vi "rio_veloster10.vi"() -> ()   [LabVIEW 2015]
uses:
  <vilib>/Analysis/Matrix/Datatypes/RealMatrix.ctl
  <vilib>/FPGAPlugInAG/cRIO-9113/niLvFpga_Open_cRIO-9113.vi
  <vilib>/rvi/interface/common/dynamic/niFpgaDynamicAddResources.vi
  <vilib>/FPGAPlugInAG/Dynamic/niLvFpga_Abort_Dynamic.vi
  <vilib>/FPGAPlugInAG/Dynamic/niLvFpga_Run_Dynamic.vi
  G_rio.vi
  <vilib>/Instr/_visa.llb/VISA Configure Serial Port (Instr).vi
  <vilib>/Utility/error.llb/Error Cluster From Error Code.vi
  <vilib>/rvi/errors/niLvFpgaAdjustHostInterfaceError.vi
  <vilib>/Analysis/Matrix/Numeric/Conversions/Array To Matrix - RA2.vi
  <vilib>/Analysis/Matrix/Numeric/Multiply/Multiply - RM,RM.vi
  <vilib>/Analysis/Matrix/Numeric/Add/Add - RM,RM.vi
  <vilib>/Analysis/baseanly.llb/Real Inverse Matrix.vi
  <vilib>/Analysis/Matrix/Numeric/Subtract/Subtract - RM,RM.vi
  <vilib>/Analysis/Matrix/Numeric/Conversions/Array To Matrix - RA.vi
  <vilib>/Analysis/Matrix/Numeric/Multiply/Multiply - R,RM.vi
  <vilib>/Analysis/Matrix/Numeric/Conversions/Matrix To Array - RM.vi
  <vilib>/rvi/interface/nirviOpenFPGA/nirviOpenFPGA.xnode
  FPGA Bitfiles/autonomous_FPGATarget2_fpga4_FZHAM7r+pqE.lvbitx
  fpga/fpga4.vi
  <vilib>/rvi/interface/nirviMethod/nirviMethod.xnode
  <vilib>/rvi/interface/nirviReadWriteControl/nirviReadWriteControl.xnode
  <vilib>/rvi/interface/Simulation/niFpgaSimulationCallBeginRW.vi
  <vilib>/rvi/errors/niLvFpgaMergeErrorWithErrorCode.vi
  NiFpgaLv.dll
  <vilib>/FPGAPlugInAG/Dynamic/niLvFpga_ReadFifo_Dynamic.vi
  <vilib>/Analysis/Matrix/NI_Matrix.lvlib
  <vilib>/Analysis/NI_AALBase.lvlib
panel:
  in  "map name":T1(ring)
  out "316H":u8[](array[numeric])
  out "FPGA":refnum<k20>
  out "Key":u8
  out "mdps torque":dbl(graph)
  out "battery voltage 2":dbl
  in  "steer limit":dbl=100.0
  in  "buzz":bool
  out "hcount":u64=1
  out "hbias":dbl
  out "vcount":u64=1
  out "vgain":dbl=1.0
  in  "heading gain":dbl=1.414
  in  "pos gain":dbl=4.0
  out "Pos_time 10":i32
  out "T PWM":u16
  out "B PWM":u16
  out "solenoid":bool
  out "brk enc":u8
  out "shift lever":dbl
  in  "LCM":bool=TRUE
  out "mobileye":u8[](array[numeric])
  out "timer":u32
  out "Mobileye_time 100":u32
  out "H_GPS":dbl
  out "pos":dbl[](array[numeric])
  out "pos error":dbl
  in  "GPS init":bool=TRUE
  in  "Gear Manual":i32(slide)=1 scale=-1.0..1.0
  out "map":i32=2
  out "P, R, D":i32
  out "heading error":dbl
  out "POS init":bool
  out "VS_CAN":dbl
  in  "brake":bool
  in  "Slide":dbl(slide)=1000.0 min=1000.0 max=2000.0 step=1500.0 scale=1000.0..2000.0
  out "novatel":refnum<visa-resource-name>
  in  "ublox":bool
  out "rest":u8[](array[numeric])
  out "GPS_novatel_time":u32
  out "GPS_time 100":u32
  out "Con_time 10":i32
  out "CAN_time 10":u32
  out "gps2":refnum<visa-resource-name>
  out "gps1":refnum<visa-resource-name>
  out "Heading":dbl
  out "ecef ref":dbl[](array[numeric])
  out "h_gps":dbl
  out "pos_gps":dbl[](array[numeric]) format="%#_19f"
  out "get heading":bool
  out "get position":bool
  out "dt":dbl
  out "rt":dbl
  out "CAN Comm Enabled":bool
  in  "SPAS Enable":bool=TRUE
  in  "file write":bool
  out "data write":refnum<file>
  out "file rw error":errorcluster
  out "Ref steer":dbl=1.0
  in  "Steer input":bool=TRUE
  in  "Ref steer manual":dbl(knob) scale=-550.0..550.0
  out "Ref vel":dbl=1.0
  in  "Ref vel manual":dbl
  in  "Velocity input":bool
  out "Auto":bool
  out "Run":bool
  out "E - STOP":bool
  out "Throttle Enable":bool=TRUE
  # "P"
  # "R"
  # "D"
  # "Ref steer manual"
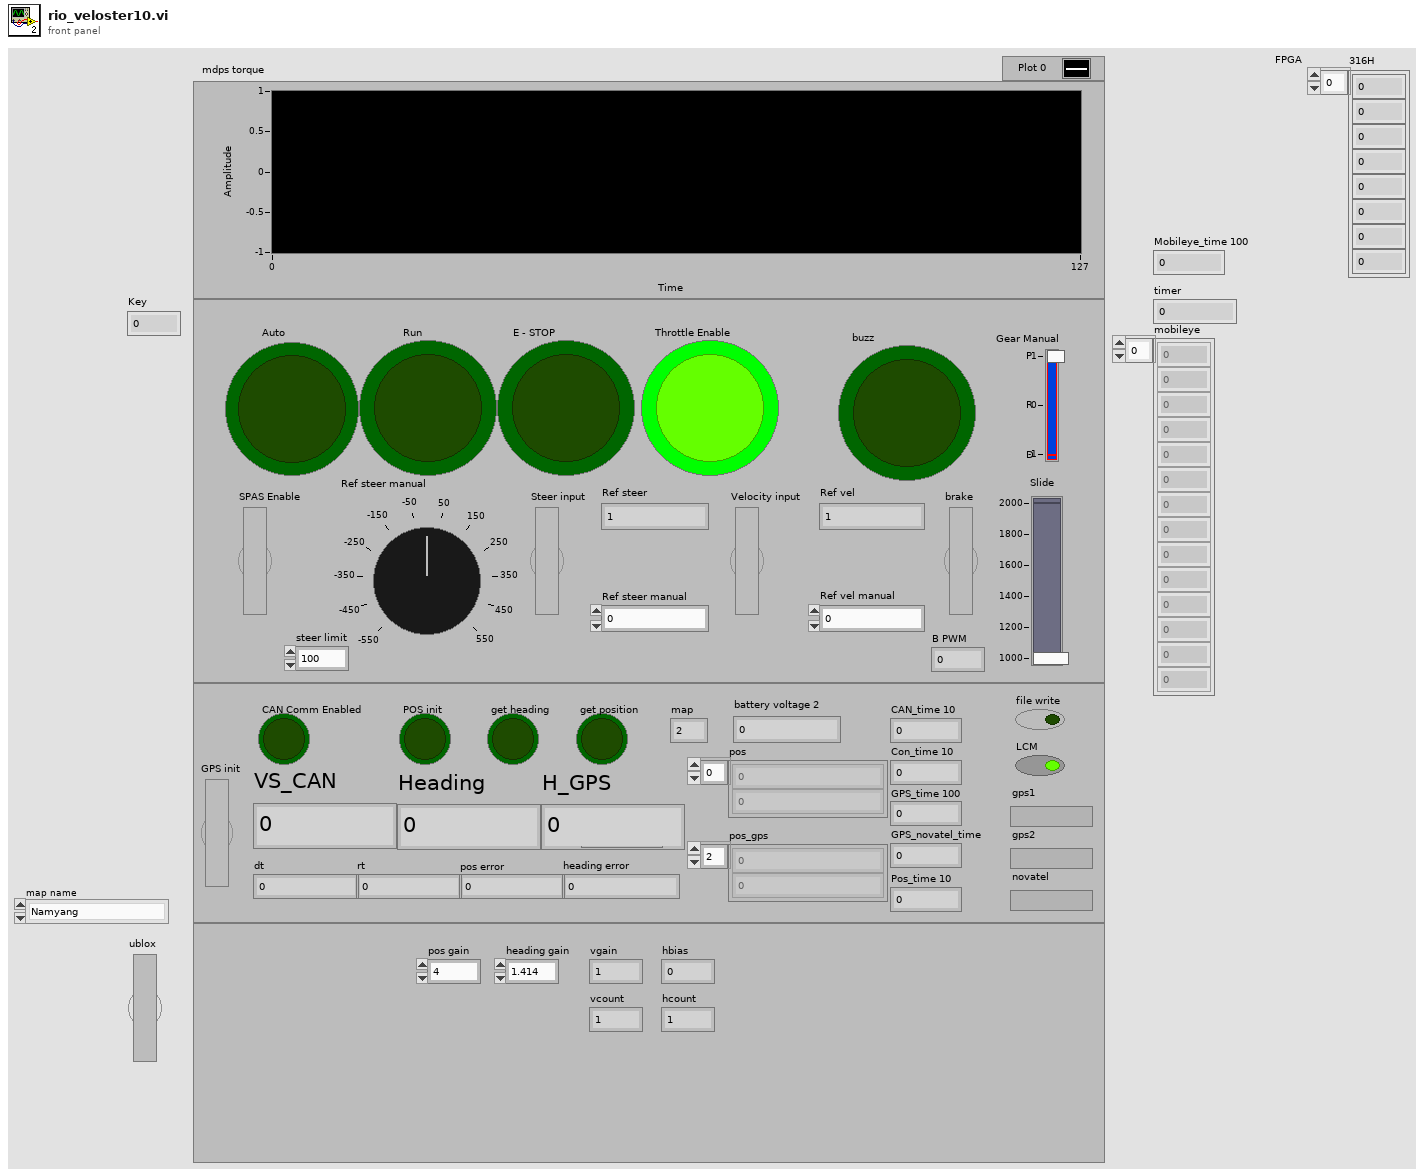
[diagram p1: front panel]
types:
  T1 = enum32{"Namyang", "Hyundai", "KAIST", "Ajou", "Munji", "Airforce", "Car", "KATRI", "Samsung", "Coex", "Gwangnaru", "Inje", "sinjin"}
  T2 = enum16{"open", "replace", "create", "open or create", "replace or create", "replace or create with confirmation"}
  T3 = cluster{"timestamp high":u32, "timestamp low":u32, "identifier":u32, "type":enum8{"Data Frame", "Remote Frame", "(reserved)", "(reserved) ", "(reserved)  ", "(reserved)   ", "Bus Error", "Transceiver Fault"}, "info A":u8, "info B":u8, "data length":u8, "data":u8[]}
  T4 = cluster{"connection ID":refnum<k16>, "net address":u32, "port":u16}
  T5 = cluster{"hash":i64, "sys time":i64, "mobileye":u8[]}
  T6 = cluster{"hash":i64, "sys time":i64, "n":i32, "error":i32[]}
  T7 = cluster{"hash":i64, "sys time":i64, "time":dbl, "yaw_rate":dbl, "mdps torque":dbl, "mdps str_ang":dbl, "VS_CAN":dbl, "lat_accel":dbl, "mcp":dbl, "accel pedal value":dbl, "tps":dbl, "odometer":dbl, "battery voltage":dbl, "WHL_SPD_RR":dbl, "WHL_SPD_RL":dbl, "WHL_SPD_FR":dbl, "WHL_SPD_FL":dbl}
  T8 = cluster{"hash":i64, "sys time":i64, "ref_vel":dbl, "ref_steer":dbl, "alert":u8}
  T9 = cluster{"hash":i64, "sys time":i64, "ref_vel":dbl, "ref_steer":dbl}
  T10 = cluster{"hash":i64, "sys time":i64, "Auto":bool, "Run":bool, "Solenoid":bool, "T lim":bool, "brk_enc":u8, "B PWM":u16, "T PWM":u16, "ref_vel":dbl, "ref_bkr_enc":dbl, "ref_apv":dbl, "ref_steer":dbl}
  T11 = typedef "NI_Matrix.lvlib/RealMatrix.ctl" = dbl[][]
  T12 = cluster{"hash":i64, "sys time":i64, "time":dbl, "x":dbl, "y":dbl, "h":dbl, "numSV":i32, "postype":i32, "lag":i32, "hordev":dbl, "lat":dbl, "lon":dbl, "hgt":dbl, "map_idx":i32}
  T13 = cluster{"LCC[0]":dbl, "LCC[1]":dbl, "LCC[2]":dbl, "LCC[3]":dbl, "LCC[4]":dbl, "LCC[5]":dbl, "LCC[6]":dbl, "LCC[7]":dbl, "LCC[8]":dbl, "LCC[9]":dbl, "LCC[10]":dbl, "LCC[11]":dbl, "LCC[12]":dbl, "LCC[13]":dbl, "LCC[14]":dbl}
  T14 = cluster{"hash":i64, "sys time":i64, "time":dbl, "speed":dbl, "heading":dbl, "lat":dbl, "lon":dbl}
  T15 = cluster{"vel[0]":dbl, "vel[1]":dbl, "vel[2]":dbl, "vel[3]":dbl, "vel[4]":dbl, "vel[5]":dbl, "vel[6]":dbl}
  T16 = cluster{"output[0]":dbl, "output[1]":dbl, "output[2]":dbl, "output[3]":dbl, "output[4]":dbl, "output[5]":dbl, "output[6]":dbl, "output[7]":dbl, "output[8]":dbl, "output[9]":dbl, "output[10]":dbl, "output[11]":dbl, "output[12]":dbl, "output[13]":dbl, "output[14]":dbl}
  T17 = cluster{"output[0]":dbl, "output[1]":dbl, "output[2]":dbl, "output[3]":dbl, "output[4]":dbl, "output[5]":dbl, "output[6]":dbl}
  T18 = cluster{"hash":i64, "sys time":i64, "dt":dbl, "x":dbl, "y":dbl, "speed":dbl, "heading":dbl, "yaw_rate":dbl}
  T19 = cluster{"Real 2D Array[0]":dbl, "Real 2D Array[1]":dbl, "Real 2D Array[2]":dbl, "Real 2D Array[3]":dbl, "Real 2D Array[4]":dbl}
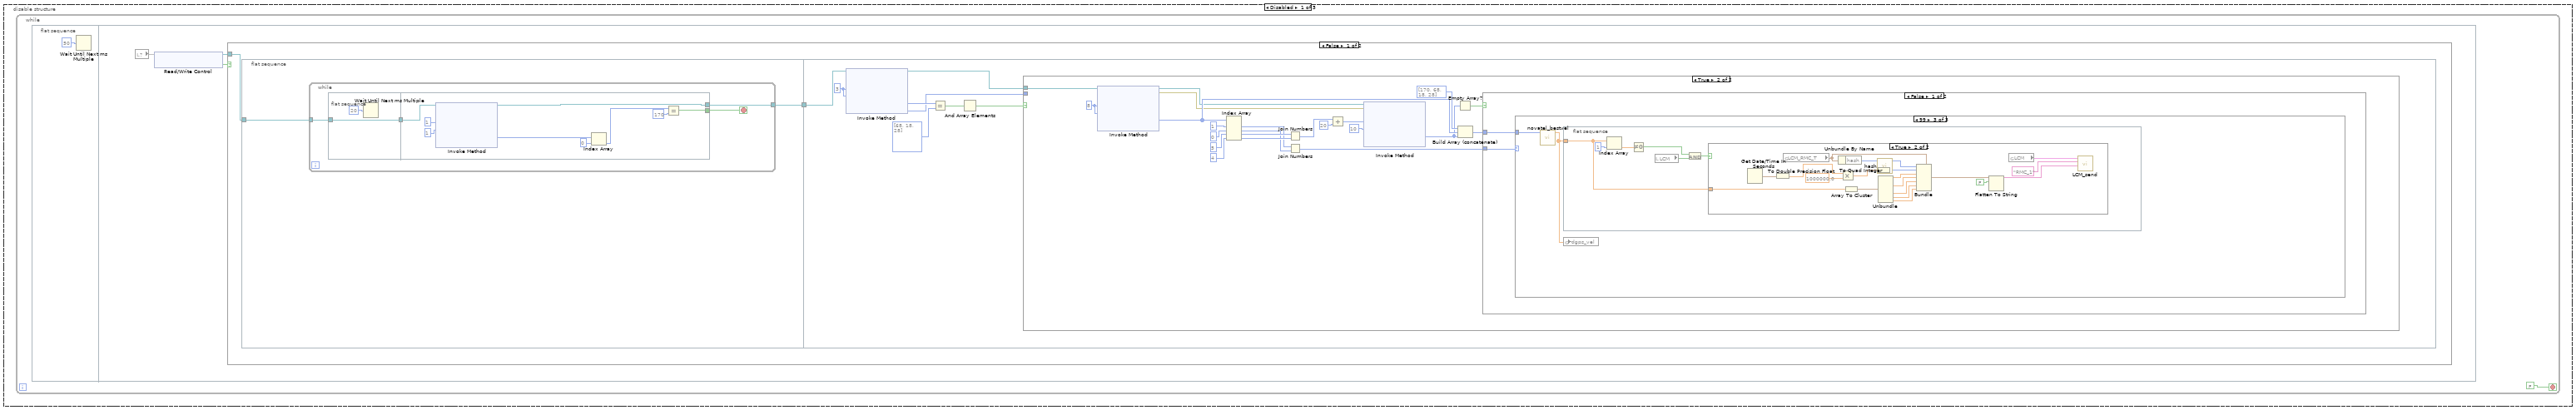
[diagram p2: hidden frame]
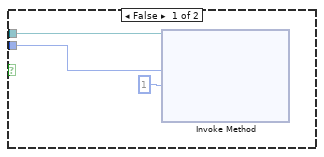
[diagram p3: hidden frame]
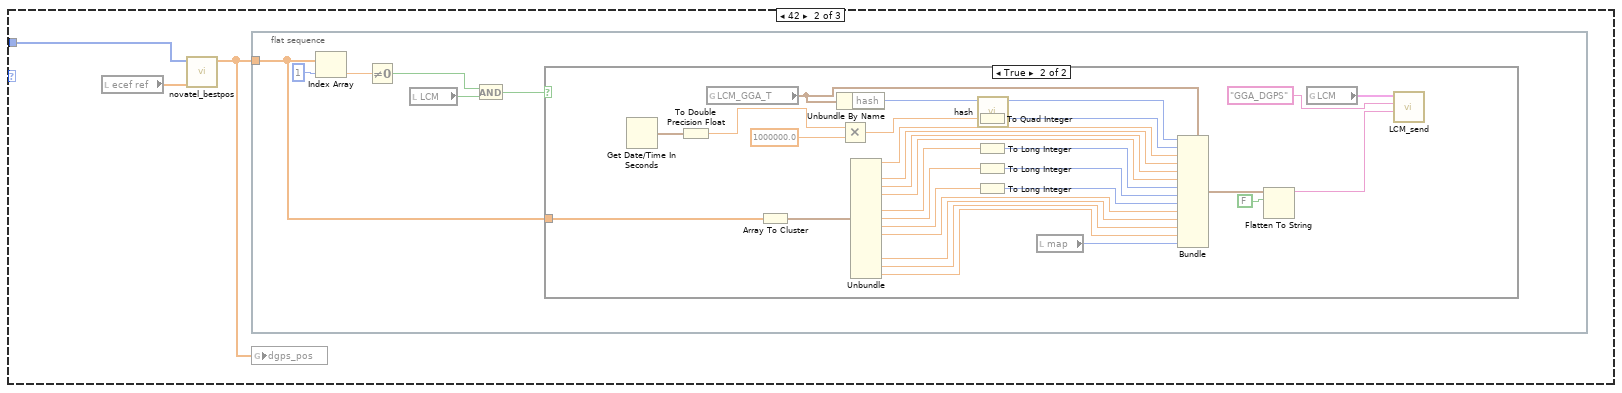
[diagram p5: hidden frame]
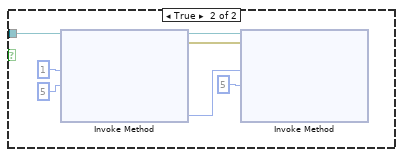
[diagram p9: hidden frame]
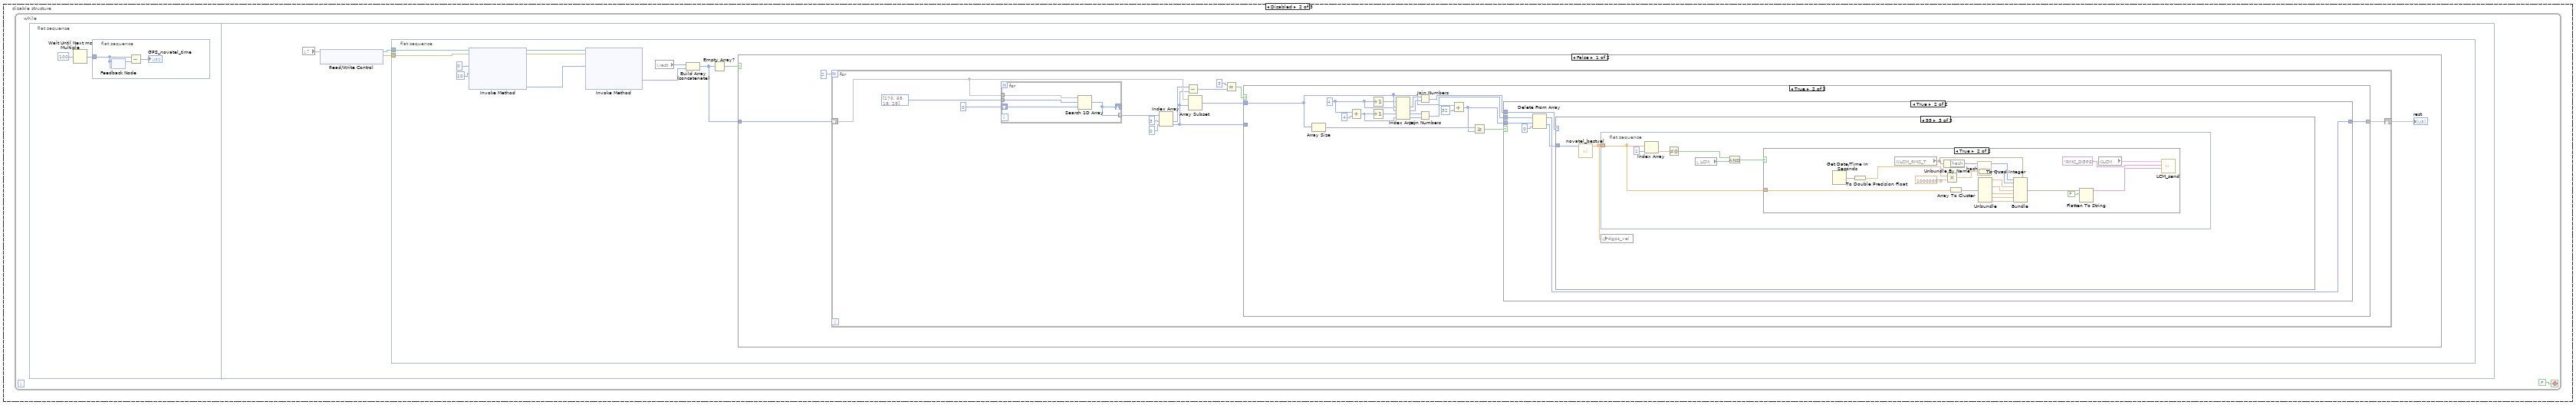
[diagram p10: hidden frame]
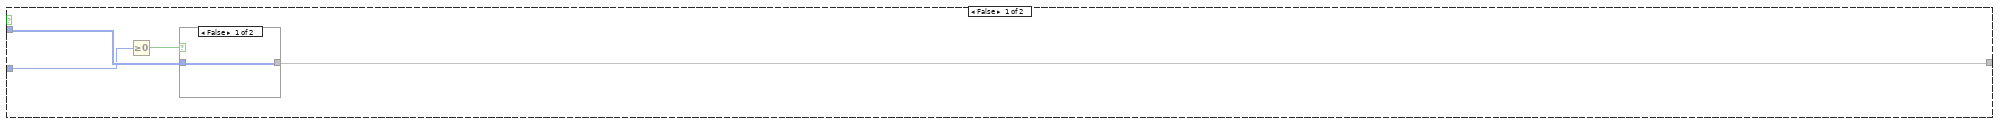
[diagram p11: hidden frame]
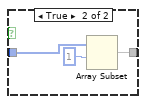
[diagram p12: hidden frame]
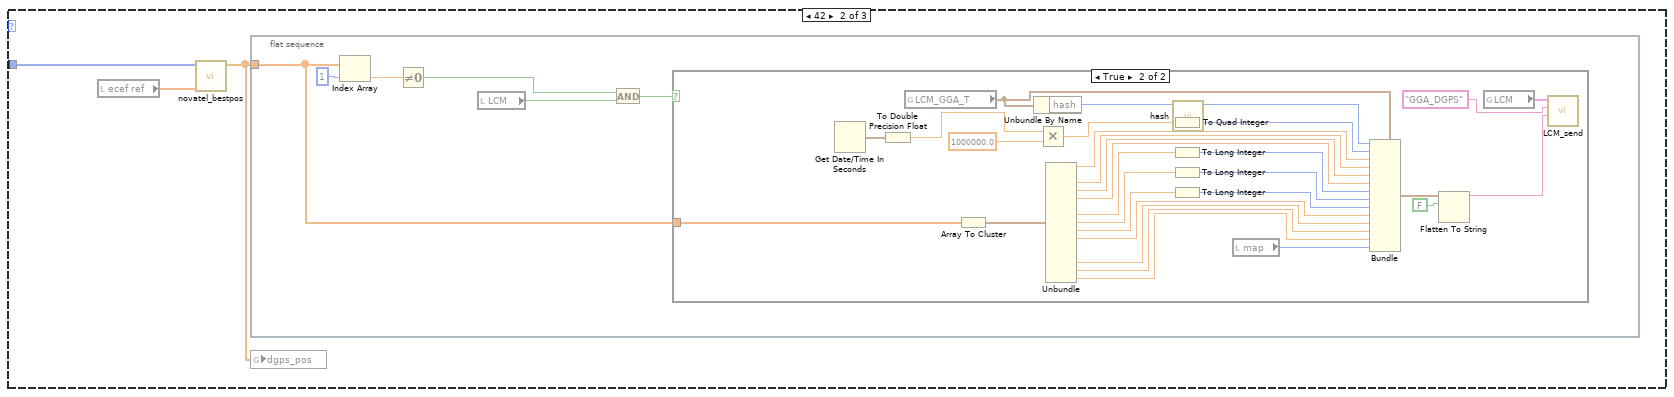
[diagram p15: hidden frame]
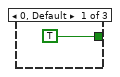
[diagram p19: hidden frame]
diagram:
  n1 = flat-sequence {
    frame #0 {
      w3 = u16 7668 ("port")
      w9 = u16 7667 ("port")
      n2 = xnode "Open FPGA VI Reference"() -> ("FPGA VI Reference Out"=w18:refnum<k20>, "error out"=w17:errorcluster)  [unwired: 2 in]
      n3 = global read "G_rio.vi" "LCM PC"() -> (w7:T4)
      n4 = Decrement(x=w9) -> (x-1=w8:u16)
      n5 = UDP Open(11:w3) -> (port=w5:refnum<k16>)  [unwired: 4 in, 2 out]
      n6 = xnode "Invoke Method"("FPGA VI Reference In"=w18, "error in"=w17) -> ("FPGA VI Reference Out"=w16:refnum<k20>, "error out"=w15:errorcluster)
      n7 = Bundle By Name(cluster=w7, "port"=w3, "connection ID"=w5, "net address"=u32 0) -> (w6:T4)
      n8 = UDP Open(11:w8) -> (port=w11:refnum<k16>)  [unwired: 4 in, 2 out]
      n9 = xnode "Invoke Method"("FPGA VI Reference In"=w16, "error in"=w15, "Wait Until Done (F)"=FALSE) -> ("FPGA VI Reference Out"=→"FPGA":refnum<k20>)  [unwired: 1 out]
      n10 = global read "G_rio.vi" "LCM"() -> (w13:T4)
      n11 = global write "G_rio.vi" "LCM PC"(w6) -> ()
      n12 = Bundle By Name(cluster=w13, "port"=w9, "connection ID"=w11, "net address"=u32 4294967295) -> (w12:T4)
      n13 = global write "G_rio.vi" "LCM"(w12) -> ()
    }
    frame #1 {
      n14 = flat-sequence {
        frame #0 {
          w60 = FALSE ("Auto")
          n15 = global write "G_rio.vi" "brake release"(FALSE ("brake release")) -> ()
          n16 = global write "G_rio.vi" "Auto"(w60) -> ()
          n17 = global write "G_rio.vi" "Auto SW"(w60) -> ()
        }
        frame #1 {
          w63 = FALSE ("GPS init")
          w64 = 0.0 ("Ref_vel_planner")
          n18 = global write "G_rio.vi" "T lim counter 2"(u16 300 ("T lim counter 2")) -> ()
          n19 = local write "Slide"(1500.0 ("Slide")) -> ()
          n20 = global write "G_rio.vi" "Ref_steer_planner"(w64) -> ()
          n21 = global write "G_rio.vi" "Ref_vel_planner"(w64) -> ()
          n22 = local write "brake"(w63) -> ()
          n23 = local write "rest"(u8[] [] ("rest")) -> ()
          n24 = local write "rest"(u8[] [] ("rest")) -> ()
          n25 = local write "Velocity input"(w63) -> ()
          n26 = local write "GPS init"(w63) -> ()
          "POS init" <- TRUE ("pos linit")
        }
      }
      n27 = disable-structure shown="Enabled" {
        frame Enabled {
          w23 = refnum<visa-resource-name> "ASRL1::INSTR" ("VISA resource name")
          w21 = refnum<visa-resource-name> "USB0::0x1546::0x01A6::NI-VISA-0::1::RAW" ("VISA resource name")
          w22 = refnum<visa-resource-name> "USB0::0x1546::0x01A6::NI-VISA-1::1::RAW" ("VISA resource name")
          n28 = call-poly "VISA Configure Serial Port"("VISA resource name"=w23, "timeout (10sec)"=u32 10, "baud rate (9600)"=u32 115200) -> ("VISA resource name out"=w25:refnum<visa-resource-name>, "error out"=w20:errorcluster)  [unwired: 11 in]
          n29 = case shown="Error" w20 {
            tunnel: [w38 w42] -> w24
            tunnel: w25 -> [w38 w41]
            tunnel: w23 -> [_ w39]
            frame No Error {
            }
            frame Error {
              n30 = VISA Close(VISA resource name=w41) -> (error out=w40:errorcluster)  [unwired: 1 in]
              n31 = call-poly "VISA Configure Serial Port"("VISA resource name"=w39, "timeout (10sec)"=u32 10, "baud rate (9600)"=u32 115200, "error in (no error)"=w40) -> ("VISA resource name out"=w42:refnum<visa-resource-name>)  [unwired: 10 in, 1 out]
            }
          }
          "novatel" <- w24
          n32 = call-poly "VISA Configure Serial Port"("VISA resource name"=w21, "timeout (10sec)"=u32 1, "baud rate (9600)"=u32 115200) -> ("VISA resource name out"=w28:refnum<visa-resource-name>, "error out"=w30:errorcluster)  [unwired: 11 in]
          n33 = call-poly "VISA Configure Serial Port"("VISA resource name"=w22, "timeout (10sec)"=u32 1, "baud rate (9600)"=u32 115200) -> ("VISA resource name out"=w26:refnum<visa-resource-name>, "error out"=w31:errorcluster)  [unwired: 11 in]
          n34 = case shown="Error" w30 {
            tunnel: [w45 w49] -> w29
            tunnel: w28 -> [w45 w48]
            tunnel: w21 -> [_ w46]
            frame No Error {
            }
            frame Error {
              n35 = VISA Close(VISA resource name=w48) -> (error out=w47:errorcluster)  [unwired: 1 in]
              n36 = call-poly "VISA Configure Serial Port"("VISA resource name"=w46, "timeout (10sec)"=u32 1, "baud rate (9600)"=u32 115200, "error in (no error)"=w47) -> ("VISA resource name out"=w49:refnum<visa-resource-name>)  [unwired: 10 in, 1 out]
            }
          }
          "gps2" <- w29
          n37 = case shown="Error" w31 {
            tunnel: [w52 w56] -> w27
            tunnel: w26 -> [w52 w55]
            tunnel: w22 -> [_ w53]
            frame No Error {
            }
            frame Error {
              n38 = VISA Close(VISA resource name=w55) -> (error out=w54:errorcluster)  [unwired: 1 in]
              n39 = call-poly "VISA Configure Serial Port"("VISA resource name"=w53, "timeout (10sec)"=u32 1, "baud rate (9600)"=u32 115200, "error in (no error)"=w54) -> ("VISA resource name out"=w56:refnum<visa-resource-name>)  [unwired: 10 in, 1 out]
            }
          }
          "gps1" <- w27
        }
        frame Disabled {
        }
      }
      n40 = case shown="True" "file write" {
        frame False {
        }
        frame True {
          n41 = Open/Create/Replace File(file path (use dialog)=path "c:/datasave", operation (0:open)=T2."replace or create", access (0:read/write)=enum16{"read/write", "read-only", "write-only"}."write-only") -> (refnum out=→"data write":refnum<file>, cancelled=w71:bool, error out=→"file rw error":errorcluster)  [unwired: 3 in]
          n42 = Not(x=w71) -> (.not. x?=w70:bool)
          n43 = local write "file write"(w70) -> ()
        }
      }
    }
    frame #2 {
      (unwired) FALSE
      n44 = disable-structure shown="Enabled" {
        frame Enabled {
          n45 = while {
            stop <- FALSE stop-if-true
            n46 = flat-sequence {
              frame #0 {
                n47 = Wait Until Next ms Multiple(millisecond multiple=u32 100) -> (millisecond timer value=w114:u32)
                n48 = flat-sequence {
                  tunnel: w114 -> [w116]
                  frame #0 {
                    n49 = feedback #1(w116) -> (w117:u32)
                    n50 = feedback-in #1(w116) -> ()
                    n51 = Subtract(x=w116, y=w117) -> (x-y=→"Mobileye_time 100":u32)
                  }
                }
              }
              frame #1 {
                n52 = local read "FPGA"() -> (w165:refnum<k20>)
                n53 = xnode "Read/Write Control"("FPGA VI Reference In"=w165) -> ("m 700"=w125:u8[], "m 760"=w161:u8[], "m 710"=w150:u8[], "m 711"=w146:u8[], "m 720"=w144:u8[], "m 721"=w143:u8[], "m 722"=w142:u8[], "m 723"=w141:u8[], "m 724"=w140:u8[], "m 725"=w139:u8[], "m 726"=w138:u8[], "m 727"=w137:u8[], "m 728"=w136:u8[], "m 729"=w135:u8[])  [unwired: 1 in, 2 out]
                n54 = Build Array(w144, w143, w142, w141, w140, w139, w138, w137, w136, w135) -> (w134:u8[][])
                n55 = Array Subset(array=w125, index=0, length=4) -> (w122:u8[])
                n56 = Array Subset(array=w146, index=6, length=6) -> (w145:u8[])
                n57 = Index Array(array=w125, index #1=4 ("index"), index #4=8 ("index"), index #5=11 ("index")) -> (element #1=w158:u8, element #2=w157:u8, element #3=w156:u8, element #4=w155:u8, element #5=w154:u8)  [unwired: 2 in]
                n58 = Index Array(array=w122, index #1=0 ("index")) -> (element #1=w131:u8, element #2=w130:u8, element #3=w129:u8, element #4=w128:u8)  [unwired: 3 in]
                n59 = Array Subset(array=w161, index=4, length=3) -> (w153:u8[])
                n60 = Array Subset(array=w150, index=5, length=7) -> (w149:u8[])
                n61 = Join Numbers(hi=w131, lo=w130) -> ((hi.lo)=w127:u16)
                n62 = Join Numbers(hi=w129, lo=w128) -> ((hi.lo)=w126:u16)
                n63 = Build Array (concatenate)(w122, w158, w157, w156, w155, w154, w153, w149, w145) -> (w133:u8[])
                n64 = for {
                  tunnel: w134 -> [w167] mode=indexing
                  shift-right: [w170] -> w121
                  shift-left: w133 -> [w171]
                  n65 = Array Subset(array=w167, index=4, length=8) -> (w166:u8[])
                  n66 = disable-structure shown="Enabled" {
                    disable-tunnel: [w174 TRUE ("lsb carry out")] -> w172
                    disable-tunnel: w166 -> [w173 _]
                    frame Disabled {
                      n67 = Index Array(array=w173, index=0) -> (element=w176:u8)
                      n68 = Rotate Right With Carry(2:w176, 3:FALSE ("carry")) -> (1:w174:bool)  [unwired: 1 out]
                    }
                    frame Enabled {
                    }
                  }
                  n69 = case shown="True" w172 {
                    tunnel: w171 -> [w179 w182]
                    tunnel: [w179 w181] -> w170
                    tunnel: w166 -> [_ w180]
                    frame False {
                    }
                    frame True {
                      n70 = Build Array (concatenate)(w182, w180) -> (w181:u8[])
                    }
                  }
                }
                "mobileye" <- w121
                n71 = Join Numbers(hi=w127, lo=w126) -> ((hi.lo)=w119:u32)
                "timer" <- w119
                n72 = feedback-in #2(w119) -> ()
                n73 = feedback #2(w119) -> (w120:u32)
                n74 = Not Equal?(x=w119, y=w120) -> (x != y?=w118:bool)
                n75 = global write "G_rio.vi" "A_camera"(w118) -> ()
              }
              frame #2 {
                n76 = local read "LCM"() -> (w183:bool)
                n77 = case shown="True" w183 {
                  frame False {
                    n78 = local read "mobileye"() -> (w184:u8[])
                    n79 = shared-variable "veloster\\sharedvari.lvlib\\mobileye"(w184) -> ()  [unwired: 1 in, 1 out]
                  }
                  frame True {
                    n80 = Get Date/Time In Seconds() -> (seconds since 1Jan1904=w189:timestamp)
                    n81 = To Double Precision Float(number=w189) -> (double precision float=w188:dbl)
                    n82 = global read "G_rio.vi" "LCM_EYE_RAW_T"() -> (w198:T5)
                    n83 = Unbundle By Name(w198) -> ("hash"=w197:i64)
                    n84 = Multiply(x=w188, y=1000000.0) -> (x*y=w186:dbl)
                    n85 = local read "mobileye"() -> (w190:u8[])
                    n86 = call "hash.vi"("input"=w197) -> ("output"=w196:i64)  [unwired: 10 in]
                    n87 = To Quad Integer(1:w186) -> (0:w185:i64)
                    n88 = Bundle By Name(cluster=w198, "hash"=w196, "sys time"=w185, "mobileye"=w190) -> (w195:T5)
                    n89 = Flatten To String(anything=w195, prepend array or string size? (T)=FALSE) -> (data string=w193:string)  [unwired: 2 in, 2 out]
                    n90 = global read "G_rio.vi" "LCM"() -> (w194:T4)
                    n91 = call "LCM_send.vi"("DATA"=w193, "ID"="EYE_RAW_T", "LCM"=w194) -> ()  [unwired: 7 in, 2 out]
                  }
                }
              }
            }
          }
        }
        frame Disabled {
        }
      }
      n92 = while {
        stop <- FALSE stop-if-true
        n93 = flat-sequence {
          frame #0 {
            n94 = global read "G_rio.vi" "PWM Brake"() -> (w76:dbl)
            n95 = global read "G_rio.vi" "PWM Brake"() -> (w92:dbl)
            n96 = Wait Until Next ms Multiple(millisecond multiple=u32 33 ("millisecond timer value")) -> ()  [unwired: 1 out]
            n97 = global read "G_rio.vi" "accel pedal value"() -> (w80:dbl)
            n98 = global read "G_rio.vi" "brake_act_can"() -> (w82:bool)
            n99 = global read "G_rio.vi" "Ref APS"() -> (w81:dbl)
            n100 = local read "Ref vel"() -> (w93:dbl)
            n101 = Greater?(x=w76, y=1000.0) -> (0:w84:bool)
            n102 = Greater?(x=w92, y=1000.0) -> (0:w89:bool)
            n103 = Not Equal To 0?(x=w81) -> (x != 0?=w79:bool)
            n104 = Equal To 0?(x=w80) -> (x = 0?=w78:bool)
            n105 = Not(x=w82) -> (.not. x?=w83:bool)
            n106 = Not Equal To 0?(x=w93) -> (x != 0?=w90:bool)
            n107 = Or(x=w90, y=w89) -> (x .or. y?=w88:bool)
            n108 = And(x=w79, y=w78) -> (x .and. y?=w85:bool)
            n109 = And(x=w84, y=w83) -> (x .and. y?=w86:bool)
            n110 = Not Or(1:w86, 2:w85) -> (0:w87:bool)
            n111 = global write "G_rio.vi" "Speed Cont"(w88) -> ()
            n112 = global write "G_rio.vi" "A_control"(w87) -> ()
          }
          frame #1 {
            n113 = disable-structure shown="Enabled" {
              frame Enabled {
                n114 = call "alertvisual.vi"() -> ()  [unwired: 12 in]
              }
              frame Disabled {
              }
            }
          }
          frame #2 {
            n115 = local read "LCM"() -> (w95:bool)
            n116 = case shown="True" w95 {
              frame False {
                n117 = local read "mobileye"() -> (w96:u8[])
                n118 = shared-variable "veloster\\sharedvari.lvlib\\mobileye"(w96) -> ()  [unwired: 1 in, 1 out]
              }
              frame True {
                n119 = Get Date/Time In Seconds() -> (seconds since 1Jan1904=w103:timestamp)
                n120 = To Double Precision Float(number=w103) -> (double precision float=w102:dbl)
                n121 = global read "G_rio.vi" "LCM_ERROR_T"() -> (w111:T6)
                n122 = global read "G_rio.vi" "error count"() -> (w97:i32[])
                n123 = Unbundle By Name(w111) -> ("hash"=w110:i64)
                n124 = Multiply(x=w102, y=1000000.0) -> (x*y=w100:dbl)
                n125 = Array Size(array=w97) -> (size(s)=w98:i32)
                n126 = To Quad Integer(1:w100) -> (0:w99:i64)
                n127 = call "hash.vi"("input"=w110) -> ("output"=w109:i64)  [unwired: 10 in]
                n128 = Bundle By Name(cluster=w111, "hash"=w109, "sys time"=w99, "n"=w98, "error"=w97) -> (w108:T6)
                n129 = Flatten To String(anything=w108, prepend array or string size? (T)=FALSE) -> (data string=w106:string)  [unwired: 2 in, 2 out]
                n130 = global read "G_rio.vi" "LCM"() -> (w107:T4)
                n131 = call "LCM_send.vi"("DATA"=w106, "ID"="ERROR_T", "LCM"=w107) -> ()  [unwired: 7 in, 2 out]
              }
            }
          }
        }
      }
      n132 = while {
        stop <- FALSE stop-if-true
        n133 = flat-sequence {
          frame #0 {
            n134 = Wait Until Next ms Multiple(millisecond multiple=u32 10) -> (millisecond timer value=w684:u32)
            n135 = flat-sequence {
              tunnel: w684 -> [w687]
              frame #0 {
                n136 = feedback #3(w687) -> (w688:u32)
                n137 = feedback-in #3(w687) -> ()
                n138 = Subtract(x=w687, y=w688) -> (x-y=→"CAN_time 10":u32)
              }
            }
          }
          frame #1 {
            n139 = disable-structure shown="Enabled" {
              disable-tunnel: [w691 _] -> w689
              frame Enabled {
                n140 = local read "FPGA"() -> (w690:refnum<k20>)
                n141 = for {
                  tunnel: u32[] [356, 544, 790, 809, 914, 1087, 1200, 1264, 1349, 1680] -> [w696] mode=indexing
                  tunnel: [w695] -> w692 mode=indexing
                  tunnel: w690 -> [w694]
                  n142 = case shown="4B0" w696 {
                    tunnel: [_ w698 w778 w810 w850 w910 w935 w1002 w1035 w1064] -> w695
                    tunnel: w694 -> [_ w697 w777 w809 w849 w909 w934 w1001 w1034 w1063]
                    frame 0, Default {
                    }
                    frame 544 {
                      n143 = flat-sequence {
                        tunnel: [w703] -> w698
                        tunnel: [w702] -> w699
                        tunnel: w697 -> [w700]
                        frame #0 {
                          n144 = xnode "Read/Write Control"("FPGA VI Reference In"=w700) -> ("can 220"=w707:u8[])  [unwired: 1 in, 2 out]
                          n145 = Index Array(array=w707, index #1=0 ("index")) -> (element #1=w713:u8, element #2=w712:u8, element #3=w711:u8, element #4=w710:u8)  [unwired: 3 in]
                          n146 = Join Numbers(hi=w713, lo=w712) -> ((hi.lo)=w709:u16)
                          n147 = Join Numbers(hi=w711, lo=w710) -> ((hi.lo)=w708:u16)
                          n148 = Join Numbers(hi=w709, lo=w708) -> ((hi.lo)=w701:u32)
                          n149 = disable-structure shown="Disabled" {
                            disable-tunnel: w701 -> [w715 _]
                            frame Disabled {
                              n150 = global write "G_rio.vi" "time"(w715) -> ()
                            }
                            frame Enabled {
                            }
                          }
                          n151 = feedback #4(u32 0) -> (w704:u32)
                          n152 = feedback-in #4(w701) -> ()
                          n153 = Not Equal?(x=w701, y=w704) -> (x != y?=w703:bool)
                          n154 = Array Subset(array=w707, index=4) -> (w702:u8[])  [unwired: 1 in]
                        }
                      }
                      n155 = case shown="True" w698 {
                        tunnel: w699 -> [_ w749]
                        frame False {
                        }
                        frame True {
                          w719 = u16 8191
                          w726 = u16 2047
                          n156 = Index Array(array=w749, index #1=5 ("index"), index #2=4 ("index"), index #3=1 ("index"), index #4=0 ("index"), index #5=7 ("index"), index #6=6 ("index")) -> (element #1=w742:u8, element #2=w741:u8, element #3=w740:u8, element #4=w739:u8, element #5=w738:u8, element #6=w737:u8)
                          n157 = Join Numbers(hi=w740, lo=w739) -> ((hi.lo)=w727:u16)
                          n158 = Join Numbers(hi=w738, lo=w737) -> ((hi.lo)=w718:u16)
                          n159 = And(x=w742, y=u8 15) -> (x .and. y?=w735:u8)
                          n160 = Logical Shift(y=i16 -6, x=w740) -> (x << y=w729:u8)
                          n161 = Logical Shift(y=i16 -6, x=w738) -> (x << y=w722:u8)
                          n162 = Equal To 0?(x=w729) -> (x = 0?=w730:bool)
                          n163 = Join Numbers(hi=w735, lo=w741) -> ((hi.lo)=w732:u16)
                          n164 = And(x=w726, y=w727) -> (x .and. y?=w725:u16)
                          n165 = And(x=w719, y=w718) -> (x .and. y?=w717:u16)
                          n166 = Not Equal?(x=w726, y=w725) -> (x != y?=w731:bool)
                          n167 = Not Equal?(x=w719, y=w717) -> (x != y?=w720:bool)
                          n168 = Equal To 0?(x=w722) -> (x = 0?=w721:bool)
                          n169 = Not Equal?(x=u16 4095, y=w732) -> (x != y?=w733:bool)
                          n170 = case shown="True" w733 {
                            tunnel: w732 -> [_ w776]
                            frame False {
                            }
                            frame True {
                              n171 = global write "G_rio.vi" "mcp"(w776) -> ()
                              n172 = Greater?(x=w776, y=u16 10) -> (0:w775:bool)
                              n173 = global write "G_rio.vi" "brake_act_can"(w775) -> ()
                            }
                          }
                          n174 = And(x=w730, y=w731) -> (x .and. y?=w724:bool)
                          n175 = And(x=w721, y=w720) -> (x .and. y?=w716:bool)
                          n176 = case shown="True" w724 {
                            tunnel: w725 -> [_ w773]
                            frame False {
                            }
                            frame True {
                              n177 = To Double Precision Float(number=w773) -> (double precision float=w772:dbl)
                              n178 = Multiply(x=w772, y=0.01) -> (x*y=w770:dbl)
                              n179 = Subtract(x=w770, y=10.23) -> (x-y=w768:dbl)
                              n180 = global write "G_rio.vi" "lat_accel"(w768) -> ()
                            }
                          }
                          n181 = case shown="True" w716 {
                            tunnel: w717 -> [_ w756]
                            frame False {
                            }
                            frame True {
                              n182 = To Double Precision Float(number=w756) -> (double precision float=w755:dbl)
                              n183 = Multiply(x=w755, y=0.01) -> (x*y=w753:dbl)
                              n184 = Subtract(x=w753, y=40.95) -> (x-y=w750:dbl)
                              n185 = disable-structure shown="Enabled" {
                                disable-tunnel: [w760 w765] -> w751
                                disable-tunnel: w750 -> [w758 w766]
                                frame Disabled {
                                n186 = Add(x=w758, y=-0.034) -> (x+y=w757:dbl)
                                n187 = Multiply(x=w757, y=1.045) -> (x*y=w761:dbl)
                                n188 = Add(x=w761, y=0.0) -> (x+y=w760:dbl)
                                }
                                frame Enabled {
                                n189 = Multiply(x=w766, y=1.007006684581104) -> (x*y=w765:dbl)
                                }
                              }
                              n190 = disable-structure shown="Enabled" {
                                disable-tunnel: w751 -> [w767 _]
                                frame Enabled {
                                n191 = global write "G_rio.vi" "yaw_rate"(w767) -> ()
                                }
                                frame Disabled {
                                }
                              }
                            }
                          }
                        }
                      }
                    }
                    frame 790 {
                      n192 = flat-sequence {
                        tunnel: [w783] -> w778
                        tunnel: [w782] -> w779
                        tunnel: w777 -> [w780]
                        frame #0 {
                          n193 = xnode "Read/Write Control"("FPGA VI Reference In"=w780) -> ("can 316"=w787:u8[])  [unwired: 1 in, 2 out]
                          n194 = Index Array(array=w787, index #1=0 ("index")) -> (element #1=w793:u8, element #2=w792:u8, element #3=w791:u8, element #4=w790:u8)  [unwired: 3 in]
                          n195 = Join Numbers(hi=w793, lo=w792) -> ((hi.lo)=w789:u16)
                          n196 = Join Numbers(hi=w791, lo=w790) -> ((hi.lo)=w788:u16)
                          n197 = Join Numbers(hi=w789, lo=w788) -> ((hi.lo)=w781:u32)
                          n198 = Array Subset(array=w787, index=4) -> (w782:u8[])  [unwired: 1 in]
                          n199 = feedback #5(u32 0) -> (w784:u32)
                          n200 = feedback-in #5(w781) -> ()
                          n201 = Not Equal?(x=w781, y=w784) -> (x != y?=w783:bool)
                        }
                      }
                      n202 = case shown="True" w778 {
                        tunnel: w779 -> [_ w807]
                        frame False {
                        }
                        frame True {
                          w798 = u8 1 ("x")
                          n203 = Index Array(array=w807, index #1=0 ("index"), index #2=3 ("index"), index #3=2 ("index")) -> (element #1=w801:u8, element #2=w804:u8, element #3=w803:u8)
                          n204 = Join Numbers(hi=w804, lo=w803) -> ((hi.lo)=w800:u16)
                          n205 = And(x=w798, y=w801) -> (x .and. y?=w799:u8)
                          n206 = Equal?(x=w798, y=w799) -> (x = y?=w797:bool)
                          n207 = Not Equal To 0?(x=w800) -> (x != 0?=w796:bool)
                          n208 = And(x=w797, y=w796) -> (x .and. y?=w795:bool)
                          n209 = case shown="False" w795 {
                            frame False {
                              n210 = global write "G_rio.vi" "Auto SW"(FALSE ("Auto SW")) -> ()
                            }
                            frame True {
                            }
                          }
                          "316H" <- w807
                        }
                      }
                    }
                    frame 809 {
                      n211 = flat-sequence {
                        tunnel: [w814] -> w810
                        tunnel: [w813] -> w811
                        tunnel: w809 -> [w812]
                        frame #0 {
                          n212 = xnode "Read/Write Control"("FPGA VI Reference In"=w812) -> ("can 329"=w819:u8[])  [unwired: 1 in, 2 out]
                          n213 = Index Array(array=w819, index #1=0 ("index")) -> (element #1=w825:u8, element #2=w824:u8, element #3=w823:u8, element #4=w822:u8)  [unwired: 3 in]
                          n214 = Join Numbers(hi=w825, lo=w824) -> ((hi.lo)=w821:u16)
                          n215 = Join Numbers(hi=w823, lo=w822) -> ((hi.lo)=w820:u16)
                          n216 = Join Numbers(hi=w821, lo=w820) -> ((hi.lo)=w815:u32)
                          n217 = Array Subset(array=w819, index=4) -> (w813:u8[])  [unwired: 1 in]
                          n218 = feedback #6(u32 0) -> (w816:u32)
                          n219 = feedback-in #6(w815) -> ()
                          n220 = Not Equal?(x=w815, y=w816) -> (x != y?=w814:bool)
                        }
                      }
                      n221 = case shown="True" w810 {
                        tunnel: w811 -> [_ w836]
                        frame False {
                        }
                        frame True {
                          # "10ms"
                          n222 = Index Array(array=w836, index #1=5 ("index"), index #2=6 ("index"), index #3=4 ("index")) -> (element #1=w833:u8, element #2=w830:u8)  [unwired: 1 out]
                          n223 = Not Equal?(x=w833, y=u8 255 ("x")) -> (x != y?=w829:bool)
                          n224 = Not Equal?(x=w830, y=u8 255 ("x")) -> (x != y?=w828:bool)
                          n225 = case shown="True" w829 {
                            tunnel: w833 -> [_ w848]
                            frame False {
                            }
                            frame True {
                              n226 = Subtract(x=w848, y=u8 32) -> (x-y=w846:u8)
                              n227 = To Double Precision Float(number=w846) -> (double precision float=w845:dbl)
                              n228 = Multiply(x=w845, y=100.0) -> (x*y=w843:dbl)
                              n229 = Divide(x=w843, y=213.0) -> (x/y=w841:dbl)
                              n230 = global write "G_rio.vi" "tps"(w841) -> ()
                            }
                          }
                          n231 = case shown="True" w828 {
                            tunnel: w830 -> [_ w840]
                            frame False {
                            }
                            frame True {
                              n232 = To Double Precision Float(number=w840) -> (double precision float=w839:dbl)
                              n233 = Multiply(x=w839, y=0.3906) -> (x*y=w838:dbl)
                              n234 = global write "G_rio.vi" "accel pedal value"(w838) -> ()
                            }
                          }
                        }
                      }
                    }
                    frame 914 {
                      n235 = flat-sequence {
                        tunnel: [w854] -> w850
                        tunnel: [w853] -> w851
                        tunnel: w849 -> [w852]
                        frame #0 {
                          n236 = xnode "Read/Write Control"("FPGA VI Reference In"=w852) -> ("can 392"=w859:u8[])  [unwired: 1 in, 2 out]
                          n237 = Index Array(array=w859, index #1=0 ("index")) -> (element #1=w865:u8, element #2=w864:u8, element #3=w863:u8, element #4=w862:u8)  [unwired: 3 in]
                          n238 = Join Numbers(hi=w865, lo=w864) -> ((hi.lo)=w861:u16)
                          n239 = Join Numbers(hi=w863, lo=w862) -> ((hi.lo)=w860:u16)
                          n240 = Join Numbers(hi=w861, lo=w860) -> ((hi.lo)=w855:u32)
                          n241 = feedback #7(u32 0) -> (w856:u32)
                          n242 = feedback-in #7(w855) -> ()
                          n243 = Not Equal?(x=w855, y=w856) -> (x != y?=w854:bool)
                          n244 = Array Subset(array=w859, index=4) -> (w853:u8[])  [unwired: 1 in]
                        }
                      }
                      n245 = case shown="True" w850 {
                        tunnel: w851 -> [_ w873]
                        frame False {
                        }
                        frame True {
                          # "20ms"
                          n246 = Array Subset(array=w873, index=0, length=7) -> (w870:u8[])
                          n247 = Index Array(array=w873, index #1=7 ("index"), index #2=2 ("index"), index #3=1 ("index"), index #4=4 ("index"), index #5=3 ("index")) -> (element #1=w867:u8, element #2=w879:u8, element #3=w878:u8, element #4=w875:u8, element #5=w874:u8)
                          n248 = Add Array Elements(numeric array=w870) -> (sum=w868:u8)
                          n249 = Equal?(x=w868, y=w867) -> (x = y?=w869:bool)
                          n250 = case shown="True" w869 {
                            tunnel: w879 -> [_ w893]
                            tunnel: w878 -> [_ w892]
                            tunnel: w875 -> [_ w889]
                            tunnel: w874 -> [_ w888]
                            frame False {
                            }
                            frame True {
                              w884 = u16 4095 ("y")
                              n251 = Join Numbers(hi=w893, lo=w892) -> ((hi.lo)=w885:u16)
                              n252 = Join Numbers(hi=w889, lo=w888) -> ((hi.lo)=w890:u16)
                              n253 = And(x=w884, y=w885) -> (x .and. y?=w883:u16)
                              n254 = Not Equal?(x=w890, y=u16 32767 ("x")) -> (x != y?=w886:bool)
                              n255 = Not Equal?(x=w884, y=w883) -> (x != y?=w887:bool)
                              n256 = case shown="True" w887 {
                                tunnel: w883 -> [_ w905]
                                frame False {
                                }
                                frame True {
                                n257 = To Double Precision Float(number=w905) -> (double precision float=w904:dbl)
                                n258 = Subtract(x=w904, y=2048.0) -> (x-y=w903:dbl)
                                n259 = Multiply(x=w903, y=0.01) -> (x*y=w906:dbl)
                                n260 = global write "G_rio.vi" "mdps torque"(w906) -> ()
                                }
                              }
                              n261 = case shown="True" w886 {
                                tunnel: w890 -> [_ w900]
                                frame False {
                                }
                                frame True {
                                n262 = To Double Precision Float(number=w900) -> (double precision float=w897:dbl)
                                n263 = Subtract(x=w897, y=65536.0) -> (x-y=w898:dbl)
                                n264 = Greater?(x=w897, y=32767.0 ("x")) -> (0:w901:bool)
                                n265 = Select(t=w898, s=w901, f=w897) -> (s? t:f=w896:dbl)
                                n266 = Multiply(x=w896, y=0.1) -> (x*y=w894:dbl)
                                n267 = global write "G_rio.vi" "mdps str_ang"(w894) -> ()
                                }
                              }
                            }
                          }
                        }
                      }
                    }
                    frame 1087 {
                      n268 = flat-sequence {
                        tunnel: [w914] -> w910
                        tunnel: [w913] -> w911
                        tunnel: w909 -> [w912]
                        frame #0 {
                          n269 = xnode "Read/Write Control"("FPGA VI Reference In"=w912) -> ("can 43F"=w919:u8[])  [unwired: 1 in, 2 out]
                          n270 = Index Array(array=w919, index #1=0 ("index")) -> (element #1=w925:u8, element #2=w924:u8, element #3=w923:u8, element #4=w922:u8)  [unwired: 3 in]
                          n271 = Join Numbers(hi=w925, lo=w924) -> ((hi.lo)=w921:u16)
                          n272 = Join Numbers(hi=w923, lo=w922) -> ((hi.lo)=w920:u16)
                          n273 = Join Numbers(hi=w921, lo=w920) -> ((hi.lo)=w915:u32)
                          n274 = Array Subset(array=w919, index=4) -> (w913:u8[])  [unwired: 1 in]
                          n275 = feedback #8(u32 0) -> (w916:u32)
                          n276 = feedback-in #8(w915) -> ()
                          n277 = Not Equal?(x=w915, y=w916) -> (x != y?=w914:bool)
                        }
                      }
                      n278 = case shown="True" w910 {
                        tunnel: w911 -> [_ w932]
                        frame False {
                        }
                        frame True {
                          w929 = u8 15 ("y")
                          # "10ms"
                          n279 = Index Array(array=w932, index=1) -> (element=w930:u8)
                          n280 = And(x=w930, y=w929) -> (x .and. y?=w928:u8)
                          n281 = Not Equal?(x=w928, y=w929) -> (x != y?=w927:bool)
                          n282 = case shown="True" w927 {
                            tunnel: w928 -> [_ w933]
                            frame False {
                            }
                            frame True {
                              n283 = global write "G_rio.vi" "gear selector disp"(w933) -> ()
                            }
                          }
                        }
                      }
                    }
                    frame 1200 {
                      n284 = flat-sequence {
                        tunnel: [w940] -> w935
                        tunnel: [w939] -> w936
                        tunnel: w934 -> [w938]
                        frame #0 {
                          n285 = xnode "Read/Write Control"("FPGA VI Reference In"=w938) -> ("can 4B0"=w944:u8[])  [unwired: 1 in, 2 out]
                          n286 = Index Array(array=w944, index #1=0 ("index")) -> (element #1=w950:u8, element #2=w949:u8, element #3=w948:u8, element #4=w947:u8)  [unwired: 3 in]
                          n287 = Join Numbers(hi=w950, lo=w949) -> ((hi.lo)=w946:u16)
                          n288 = Join Numbers(hi=w948, lo=w947) -> ((hi.lo)=w945:u16)
                          n289 = Join Numbers(hi=w946, lo=w945) -> ((hi.lo)=w937:u32)
                          n290 = Array Subset(array=w944, index=4) -> (w939:u8[])  [unwired: 1 in]
                          n291 = global write "G_rio.vi" "time"(w937) -> ()
                          n292 = feedback #9(u32 0) -> (w941:u32)
                          n293 = feedback-in #9(w937) -> ()
                          n294 = Not Equal?(x=w937, y=w941) -> (x != y?=w940:bool)
                        }
                      }
                      n295 = case shown="True" w935 {
                        tunnel: w936 -> [_ w981]
                        frame False {
                        }
                        frame True {
                          w955 = u16 16383 ("x")
                          w968 = u16 16383 ("x")
                          # "20ms"
                          n296 = Index Array(array=w981, index #1=1 ("index"), index #2=0 ("index"), index #3=3 ("index"), index #4=2 ("index"), index #5=5 ("index"), index #6=4 ("index"), index #7=7 ("index"), index #8=6 ("index")) -> (element #1=w960:u8, element #2=w959:u8, element #3=w958:u8, element #4=w957:u8, element #5=w978:u8, element #6=w977:u8, element #7=w973:u8, element #8=w972:u8)
                          n297 = Join Numbers(hi=w960, lo=w959) -> ((hi.lo)=w956:u16)
                          n298 = Join Numbers(hi=w958, lo=w957) -> ((hi.lo)=w954:u16)
                          n299 = Join Numbers(hi=w978, lo=w977) -> ((hi.lo)=w976:u16)
                          n300 = Join Numbers(hi=w973, lo=w972) -> ((hi.lo)=w969:u16)
                          n301 = And(x=w956, y=w955) -> (x .and. y?=w953:u16)
                          n302 = And(x=w955, y=w954) -> (x .and. y?=w952:u16)
                          n303 = And(x=w976, y=w968) -> (x .and. y?=w967:u16)
                          n304 = And(x=w968, y=w969) -> (x .and. y?=w966:u16)
                          n305 = Not Equal?(x=w967, y=w968) -> (x != y?=w971:bool)
                          n306 = Not Equal?(x=w968, y=w966) -> (x != y?=w970:bool)
                          n307 = And(x=w971, y=w970) -> (x .and. y?=w965:bool)
                          n308 = case shown="True" w965 {
                            tunnel: w967 -> [_ w1000]
                            tunnel: w966 -> [_ w999]
                            tunnel: w953 -> [_ w992]
                            tunnel: w952 -> [_ w991]
                            frame False {
                            }
                            frame True {
                              w987 = 0.03125 ("y")
                              w998 = 0.03125 ("y")
                              n309 = To Double Precision Float(number=w992) -> (double precision float=w989:dbl)
                              n310 = To Double Precision Float(number=w991) -> (double precision float=w986:dbl)
                              n311 = To Double Precision Float(number=w1000) -> (double precision float=w990:dbl)
                              n312 = To Double Precision Float(number=w999) -> (double precision float=w984:dbl)
                              n313 = Multiply(x=w989, y=w987) -> (x*y=w988:dbl)
                              n314 = Multiply(x=w987, y=w986) -> (x*y=w985:dbl)
                              n315 = Multiply(x=w990, y=w998) -> (x*y=w982:dbl)
                              n316 = Multiply(x=w998, y=w984) -> (x*y=w983:dbl)
                              n317 = global write "G_rio.vi" "WHL_SPD_FL"(w988) -> ()
                              n318 = global write "G_rio.vi" "WHL_SPD_FR"(w985) -> ()
                              n319 = global write "G_rio.vi" "WHL_SPD_RL"(w982) -> ()
                              n320 = global write "G_rio.vi" "WHL_SPD_RR"(w983) -> ()
                              n321 = Add(x=w982, y=w983) -> (x+y=w997:dbl)
                              n322 = Multiply(x=w997, y=0.5) -> (x*y=w994:dbl)
                              n323 = Multiply(x=w994, y=1.028) -> (x*y=w993:dbl)
                              n324 = global write "G_rio.vi" "vs_esc"(w993) -> ()
                            }
                          }
                        }
                      }
                    }
                    frame 1264 {
                      n325 = flat-sequence {
                        tunnel: [w1006] -> w1002
                        tunnel: [w1005] -> w1003
                        tunnel: w1001 -> [w1004]
                        frame #0 {
                          n326 = xnode "Read/Write Control"("FPGA VI Reference In"=w1004) -> ("can 4F0"=w1011:u8[])  [unwired: 1 in, 2 out]
                          n327 = Index Array(array=w1011, index #1=0 ("index")) -> (element #1=w1017:u8, element #2=w1016:u8, element #3=w1015:u8, element #4=w1014:u8)  [unwired: 3 in]
                          n328 = Join Numbers(hi=w1017, lo=w1016) -> ((hi.lo)=w1013:u16)
                          n329 = Join Numbers(hi=w1015, lo=w1014) -> ((hi.lo)=w1012:u16)
                          n330 = Join Numbers(hi=w1013, lo=w1012) -> ((hi.lo)=w1007:u32)
                          n331 = Array Subset(array=w1011, index=4) -> (w1005:u8[])  [unwired: 1 in]
                          n332 = feedback #10(u32 0) -> (w1008:u32)
                          n333 = feedback-in #10(w1007) -> ()
                          n334 = Not Equal?(x=w1007, y=w1008) -> (x != y?=w1006:bool)
                        }
                      }
                      n335 = case shown="True" w1002 {
                        tunnel: w1003 -> [_ w1031]
                        frame False {
                        }
                        frame True {
                          # "20 ms"
                          n336 = Index Array(array=w1031, index #1=7 ("index"), index #2=6 ("index"), index #3=5 ("index")) -> (element #1=w1025:u8, element #2=w1027:u8, element #3=w1026:u8)
                          n337 = Join Numbers(hi=w1027, lo=w1026) -> ((hi.lo)=w1022:u16)
                          n338 = Join Numbers(hi=u8 0, lo=w1025) -> ((hi.lo)=w1023:u16)
                          n339 = Join Numbers(hi=w1023, lo=w1022) -> ((hi.lo)=w1020:u32)
                          n340 = Not Equal?(x=u32 16777215, y=w1020) -> (x != y?=w1019:bool)
                          n341 = case shown="True" w1019 {
                            tunnel: w1020 -> [_ w1033]
                            frame False {
                            }
                            frame True {
                              n342 = To Double Precision Float(number=w1033) -> (double precision float=w1032:dbl)
                              n343 = global write "G_rio.vi" "odometer"(w1032) -> ()
                            }
                          }
                        }
                      }
                    }
                    frame 1349 {
                      n344 = flat-sequence {
                        tunnel: [w1039] -> w1035
                        tunnel: [w1038] -> w1036
                        tunnel: w1034 -> [w1037]
                        frame #0 {
                          n345 = xnode "Read/Write Control"("FPGA VI Reference In"=w1037) -> ("can 545"=w1044:u8[])  [unwired: 1 in, 2 out]
                          n346 = Index Array(array=w1044, index #1=0 ("index")) -> (element #1=w1050:u8, element #2=w1049:u8, element #3=w1048:u8, element #4=w1047:u8)  [unwired: 3 in]
                          n347 = Join Numbers(hi=w1050, lo=w1049) -> ((hi.lo)=w1046:u16)
                          n348 = Join Numbers(hi=w1048, lo=w1047) -> ((hi.lo)=w1045:u16)
                          n349 = Join Numbers(hi=w1046, lo=w1045) -> ((hi.lo)=w1040:u32)
                          n350 = Array Subset(array=w1044, index=4) -> (w1038:u8[])  [unwired: 1 in]
                          n351 = feedback #11(u32 0) -> (w1041:u32)
                          n352 = feedback-in #11(w1040) -> ()
                          n353 = Not Equal?(x=w1040, y=w1041) -> (x != y?=w1039:bool)
                        }
                      }
                      n354 = case shown="True" w1035 {
                        tunnel: w1036 -> [_ w1052]
                        frame False {
                        }
                        frame True {
                          n355 = Index Array(array=w1052, index=3) -> (element=w1054:u8)
                          n356 = Not Equal?(x=w1054, y=u8 255 ("x")) -> (x != y?=w1056:bool)
                          n357 = case shown="True" w1056 {
                            tunnel: w1054 -> [_ w1062]
                            frame False {
                            }
                            frame True {
                              n358 = To Double Precision Float(number=w1062) -> (double precision float=w1061:dbl)
                              n359 = Multiply(x=26.0, y=w1061) -> (x*y=w1059:dbl)
                              n360 = Divide(x=w1059, y=256.0) -> (x/y=w1057:dbl)
                              "battery voltage 2" <- w1057
                              n361 = global write "G_rio.vi" "battery voltage"(w1057) -> ()
                            }
                          }
                        }
                      }
                    }
                    frame 1680 {
                      n362 = flat-sequence {
                        tunnel: [w1068] -> w1064
                        tunnel: [w1067] -> w1065
                        tunnel: w1063 -> [w1066]
                        frame #0 {
                          n363 = xnode "Read/Write Control"("FPGA VI Reference In"=w1066) -> ("can 690"=w1073:u8[])  [unwired: 1 in, 2 out]
                          n364 = Index Array(array=w1073, index #1=0 ("index")) -> (element #1=w1079:u8, element #2=w1078:u8, element #3=w1077:u8, element #4=w1076:u8)  [unwired: 3 in]
                          n365 = Join Numbers(hi=w1079, lo=w1078) -> ((hi.lo)=w1075:u16)
                          n366 = Join Numbers(hi=w1077, lo=w1076) -> ((hi.lo)=w1074:u16)
                          n367 = Join Numbers(hi=w1075, lo=w1074) -> ((hi.lo)=w1069:u32)
                          n368 = Array Subset(array=w1073, index=4) -> (w1067:u8[])  [unwired: 1 in]
                          n369 = feedback #12(u32 0) -> (w1070:u32)
                          n370 = feedback-in #12(w1069) -> ()
                          n371 = Not Equal?(x=w1069, y=w1070) -> (x != y?=w1068:bool)
                        }
                      }
                      n372 = case shown="True" w1064 {
                        tunnel: w1065 -> [_ w1085]
                        frame False {
                        }
                        frame True {
                          n373 = Index Array(array=w1085, index=0) -> (element=w1082:u8)
                          n374 = And(x=u8 3, y=w1082) -> (x .and. y?=→"Key":u8)
                        }
                      }
                    }
                  }
                }
                n375 = Or Array Elements(Boolean array=w692) -> (logical OR=w691:bool)
              }
              frame Disabled {
              }
            }
            "CAN Comm Enabled" <- w689
            n376 = global write "G_rio.vi" "A_CAN"(w689) -> ()
          }
          frame #2 {
            n377 = global read "G_rio.vi" "gear selector disp"() -> (w1090:i8)
            n378 = global read "G_rio.vi" "vs_esc"() -> (w1086:dbl)
            n379 = Negate(x=w1086) -> (-x=w1088:dbl)
            n380 = Equal?(x=w1090, y=u8 7) -> (x = y?=w1089:bool)
            n381 = Select(t=w1088, s=w1089, f=w1086) -> (s? t:f=w1087:dbl)
            "VS_CAN" <- w1087
            n382 = global write "G_rio.vi" "VS_CAN"(w1087) -> ()
          }
          frame #3 {
            n383 = local read "CAN Comm Enabled"() -> (w1093:bool)
            n384 = local read "LCM"() -> (w1094:bool)
            n385 = And(x=w1094, y=w1093) -> (x .and. y?=w1092:bool)
            n386 = case shown="True" w1092 {
              frame False {
              }
              frame True {
                n387 = Get Date/Time In Seconds() -> (seconds since 1Jan1904=w1103:timestamp)
                n388 = global read "G_rio.vi" "LCM_CAN_T"() -> (w1120:T7)
                n389 = To Double Precision Float(number=w1103) -> (double precision float=w1102:dbl)
                n390 = global read "G_rio.vi" "accel pedal value"() -> (w1110:dbl)
                n391 = global read "G_rio.vi" "battery voltage"() -> (w1109:dbl)
                n392 = global read "G_rio.vi" "time"() -> (w1122:u32)
                n393 = global read "G_rio.vi" "mcp"() -> (w1121:u16)
                n394 = Unbundle By Name(w1120) -> ("hash"=w1119:i64)
                n395 = global read "G_rio.vi" "mdps str_ang"() -> (w1114:dbl)
                n396 = global read "G_rio.vi" "WHL_SPD_RR"() -> (w1098:dbl)
                n397 = global read "G_rio.vi" "WHL_SPD_RL"() -> (w1097:dbl)
                n398 = global read "G_rio.vi" "WHL_SPD_FR"() -> (w1096:dbl)
                n399 = global read "G_rio.vi" "WHL_SPD_FL"() -> (w1095:dbl)
                n400 = Multiply(x=w1102, y=1000000.0) -> (x*y=w1100:dbl)
                n401 = global read "G_rio.vi" "mdps torque"() -> (w1115:dbl)
                n402 = global read "G_rio.vi" "odometer"() -> (w1107:dbl)
                n403 = global read "G_rio.vi" "yaw_rate"() -> (w1116:dbl)
                n404 = global read "G_rio.vi" "lat_accel"() -> (w1113:dbl)
                n405 = global read "G_rio.vi" "VS_CAN"() -> (w1108:dbl)
                n406 = call "hash.vi"("input"=w1119) -> ("output"=w1118:i64)  [unwired: 10 in]
                n407 = To Quad Integer(1:w1100) -> (0:w1099:i64)
                n408 = To Double Precision Float(number=w1122) -> (double precision float=w1117:dbl)
                n409 = To Double Precision Float(number=w1121) -> (double precision float=w1112:dbl)
                n410 = global read "G_rio.vi" "tps"() -> (w1111:dbl)
                n411 = Bundle By Name(cluster=w1120, "hash"=w1118, "sys time"=w1099, "time"=w1117, "yaw_rate"=w1116, "mdps torque"=w1115, "mdps str_ang"=w1114, "VS_CAN"=w1108, "lat_accel"=w1113, "mcp"=w1112, "accel pedal value"=w1110, "tps"=w1111, "odometer"=w1107, "battery voltage"=w1109, "WHL_SPD_RR"=w1098, "WHL_SPD_RL"=w1097, "WHL_SPD_FR"=w1096, "WHL_SPD_FL"=w1095) -> (w1106:T7)
                n412 = Flatten To String(anything=w1106, prepend array or string size? (T)=FALSE) -> (data string=w1105:string)  [unwired: 2 in, 2 out]
                n413 = disable-structure shown="Enabled" {
                  disable-tunnel: w1105 -> [w1124 _]
                  frame Enabled {
                    n414 = global read "G_rio.vi" "LCM"() -> (w1125:T4)
                    n415 = call "LCM_send.vi"("DATA"=w1124, "ID"="CAN_T", "LCM"=w1125) -> ()  [unwired: 7 in, 2 out]
                  }
                  frame Disabled {
                  }
                }
              }
            }
          }
        }
      }
      n416 = while {
        stop <- FALSE stop-if-true
        n417 = flat-sequence {
          frame #0 {
            n418 = Wait Until Next ms Multiple(millisecond multiple=u32 10) -> (millisecond timer value=w200:u32)
            n419 = flat-sequence {
              tunnel: w200 -> [w204]
              frame #0 {
                n420 = feedback #13(w204) -> (w205:u32)
                n421 = feedback-in #13(w204) -> ()
                n422 = Subtract(x=w204, y=w205) -> (x-y=w203:u32)
                n423 = To Long Integer(number=w203) -> (32bit integer=→"Con_time 10":i32)
              }
            }
          }
          frame #1 {
            n424 = disable-structure shown="Enabled" {
              disable-tunnel: [w228 TRUE ("Auto SW")] -> w209
              frame Disabled {
                n425 = global read "G_rio.vi" "Auto SW"() -> (w228:bool)
              }
              frame Enabled {
              }
            }
            n426 = flat-sequence {
              frame #0 {
                n427 = local read "LCM"() -> (w240:bool)
                n428 = case shown="True" w240 {
                  frame False {
                    n429 = shared-variable "veloster\\sharedvari.lvlib\\vs_des"() -> (w247:dbl)  [unwired: 1 in, 1 out]
                    n430 = global read "G_rio.vi" "Ref_vel_planner"() -> (w246:dbl)
                    n431 = shared-variable "veloster\\sharedvari.lvlib\\steer_input"() -> (w244:dbl)  [unwired: 1 in, 1 out]
                    n432 = global read "G_rio.vi" "Ref_steer_planner"() -> (w245:dbl)
                    n433 = Not A Number/Path/Refnum?(number/path/refnum=w247) -> (NaN/Path/Refnum?=w248:bool)
                    n434 = Select(t=w246, s=w248, f=w247) -> (s? t:f=w241:dbl)
                    n435 = Not A Number/Path/Refnum?(number/path/refnum=w244) -> (NaN/Path/Refnum?=w243:bool)
                    n436 = global write "G_rio.vi" "Ref_vel_planner"(w241) -> ()
                    n437 = Select(t=w245, s=w243, f=w244) -> (s? t:f=w242:dbl)
                    n438 = global write "G_rio.vi" "Ref_steer_planner"(w242) -> ()
                  }
                  frame True {
                    n439 = global read "G_rio.vi" "LCM PC"() -> (w251:T4)
                    n440 = call "LCM_read.vi"("LCM"=w251) -> ("data"=w249:string, "ID"=w250:string)  [unwired: 7 in, 2 out]
                    n441 = case shown="\"CON_INPUT_T\"" w250 {
                      tunnel: w249 -> [_ w252]
                      frame "False", Default {
                      }
                      frame "CON_INPUT_T" {
                        n442 = global read "G_rio.vi" "CON_INPUT_T 2"() -> (w254:T8)
                        n443 = Unflatten From String(type=w254, binary string=w252, data includes array or string size? (T)=FALSE) -> (value=w253:T8, error out=w255:errorcluster)  [unwired: 2 in, 1 out]
                        n444 = case shown="No Error" w255 {
                          tunnel: w253 -> [w263 _]
                          tunnel: w252 -> [_ w264]
                          frame No Error {
                            w259 = u8 1 ("y")
                            n445 = Unbundle By Name(w263) -> ("ref_vel"=w262:dbl, "ref_steer"=w261:dbl, "alert"=w260:u8)
                            n446 = And(x=w260, y=w259) -> (x .and. y?=w258:u8)
                            n447 = global write "G_rio.vi" "Ref_vel_planner"(w262) -> ()
                            n448 = global write "G_rio.vi" "Ref_steer_planner"(w261) -> ()
                            n449 = Equal?(x=w258, y=w259) -> (x = y?=w257:bool)
                            n450 = global write "G_rio.vi" "A_laser"(w257) -> ()
                          }
                          frame Error {
                            n451 = global read "G_rio.vi" "CON_INPUT_T"() -> (w267:T9)
                            n452 = Unflatten From String(type=w267, binary string=w264, data includes array or string size? (T)=FALSE) -> (value=w269:T9)  [unwired: 2 in, 2 out]
                            n453 = Unbundle By Name(w269) -> ("ref_vel"=w266:dbl, "ref_steer"=w265:dbl)
                            n454 = global write "G_rio.vi" "Ref_vel_planner"(w266) -> ()
                            n455 = global write "G_rio.vi" "Ref_steer_planner"(w265) -> ()
                          }
                        }
                      }
                    }
                  }
                }
              }
            }
            n456 = global read "G_rio.vi" "Throttle_Enable"() -> (→"Throttle Enable":bool)
            n457 = local read "FPGA"() -> (w225:refnum<k20>)
            n458 = xnode "Read/Write Control"("FPGA VI Reference In"=w225) -> ("Auto"=w208:bool, "Run"=w224:bool, "T Lim"=w226:bool, "brk enc"=w214:u8)  [unwired: 1 in, 2 out]
            "brk enc" <- w214
            n459 = global write "G_rio.vi" "T Lim"(w226) -> ()
            n460 = case shown="True" w209 {
              tunnel: w208 -> [w235 w238]
              tunnel: [_ w237] -> w207
              frame False {
                n461 = case shown="False" w235 {
                  frame False {
                    n462 = global write "G_rio.vi" "Auto SW"(TRUE ("Auto SW")) -> ()
                  }
                  frame True {
                  }
                }
              }
              frame True {
                n463 = case shown="True" w238 {
                  tunnel: [_ TRUE] -> w237
                  frame False {
                  }
                  frame True {
                  }
                }
              }
            }
            "Auto" <- w207
            n464 = To Double Precision Float(number=w214) -> (double precision float=w222:dbl)
            n465 = Subtract(x=w222, y=220.0) -> (x-y=w220:dbl)
            n466 = Multiply(x=w220, y=-100.0) -> (x*y=w217:dbl)
            n467 = Divide(x=w217, y=175.0) -> (x/y=w216:dbl)
            n468 = In Range and Coerce(upper limit=100.0, x=w216, lower limit=0.0) -> (coerced(x)=w213:dbl)  [unwired: 1 out]
            n469 = global write "G_rio.vi" "Auto"(w207) -> ()
            n470 = global write "G_rio.vi" "brake encoder"(w213) -> ()
            n471 = case shown="False" w207 {
              tunnel: [_ w231] -> w206
              frame False {
                n472 = global write "G_rio.vi" "Auto SW counter"(u16 0 ("Auto SW counter")) -> ()
              }
              frame True {
                n473 = global read "G_rio.vi" "brake_act_can"() -> (w234:bool)
                n474 = global read "G_rio.vi" "brake release"() -> (w232:bool)
                n475 = Not(x=w234) -> (.not. x?=w233:bool)
                n476 = Or(x=w232, y=w233) -> (x .or. y?=w231:bool)
              }
            }
            n477 = And(x=w207, y=w224) -> (x .and. y?=w211:bool)
            "Run" <- w211
            n478 = global write "G_rio.vi" "Run"(w211) -> ()
            n479 = Not(x=w211) -> (.not. x?=w210:bool)
            n480 = And(x=w207, y=w210) -> (x .and. y?=→"E - STOP":bool)
            n481 = global write "G_rio.vi" "brake release"(w206) -> ()
          }
          frame #2 {
            n482 = flat-sequence {
              frame #0 {
                n483 = global read "G_rio.vi" "Ref_vel_planner"() -> (w328:dbl)
                n484 = Select(t=w328, s="Velocity input", f="Ref vel manual") -> (s? t:f=w331:dbl)
                n485 = To Long Integer(number=w331) -> (32bit integer=w330:i32)
                n486 = Sign(1:w330) -> (0:w329:i32)
                "P, R, D" <- w329
                n487 = case shown="1" w329 {
                  tunnel: [w335 _ w342] -> w332
                  tunnel: w331 -> [w337 _ w341]
                  frame -1 {
                    n488 = global read "G_rio.vi" "gear selector disp"() -> (w340:i8)
                    n489 = Equal?(x=w340, y=u8 7) -> (x = y?=w338:bool)
                    n490 = Select(t=w337, s=w338, f=0.0) -> (s? t:f=w335:dbl)
                  }
                  frame 0, Default {
                  }
                  frame 1 {
                    n491 = global read "G_rio.vi" "gear selector disp"() -> (w343:i8)
                    n492 = case shown="4, 5" w343 {
                      tunnel: [_ w344] -> w342
                      tunnel: w341 -> [_ w344]
                      frame 0, Default {
                      }
                      frame 4, 5 {
                      }
                    }
                  }
                }
                "Ref vel" <- w332
              }
            }
            n493 = disable-structure shown="Enabled" {
              disable-tunnel: [w272 TRUE ("Steer input")] -> w270
              frame Disabled {
                n494 = feedback #14(FALSE ("Steer input")) -> (w272:bool)
                n495 = Not(x=w272) -> (.not. x?=w271:bool)
                n496 = feedback-in #14(w271) -> ()
              }
              frame Enabled {
              }
            }
            n497 = case shown="True" w270 {
              frame False {
              }
              frame True {
                n498 = flat-sequence {
                  frame #0 {
                    n499 = global read "G_rio.vi" "Ref_steer_planner"() -> (w278:dbl)
                    n500 = global read "G_rio.vi" "mdps str_ang"() -> (w281:dbl)
                    n501 = global read "G_rio.vi" "mdps str_ang"() -> (w280:dbl)
                    n502 = Negate(x="Ref steer manual") -> (-x=w276:dbl)
                    n503 = Add(x=w281, y="steer limit") -> (x+y=w283:dbl)
                    n504 = Select(t=w278, s="Steer input", f=w276) -> (s? t:f=w279:dbl)
                    n505 = Subtract(x=w280, y="steer limit") -> (x-y=w282:dbl)
                    n506 = In Range and Coerce(upper limit=w283, x=w279, lower limit=w282) -> (coerced(x)=→"Ref steer":dbl)  [unwired: 1 out]
                  }
                  frame #1 {
                    w289 = u8 0 ("element")
                    n507 = local read "Ref steer"() -> (w291:dbl)
                    n508 = Multiply(x=w291, y=10.0) -> (x*y=w300:dbl)
                    n509 = Greater Than 0?(x=w300) -> (x > 0?=w301:bool)
                    n510 = Add(x=w300, y=65536.0) -> (x+y=w298:dbl)
                    n511 = Select(t=w300, s=w301, f=w298) -> (s? t:f=w297:dbl)
                    n512 = To Unsigned Word Integer(number=w297) -> (unsigned 16bit integer=w288:u16)
                    n513 = Split Number(x=w288) -> (hi(x)=w296:u8, lo(x)=w295:u8)
                    n514 = Build Array(u8 0 ("Con steer status"), w295, w296, w289, w289, w289, w289) -> (w293:u8[])
                    n515 = global read "G_rio.vi" "Auto"() -> (w303:bool)
                    n516 = Add Array Elements(numeric array=w293) -> (sum=w294:u8)
                    n517 = And(x=w303, y="SPAS Enable") -> (x .and. y?=w286:bool)
                    n518 = Build Array (concatenate)(w293, w294) -> (w290:u8[])
                    n519 = global write "G_rio.vi" "Steering Cont"(w286) -> ()
                    n520 = local read "FPGA"() -> (w287:refnum<k20>)
                    n521 = case shown="True" w286 {
                      tunnel: w290 -> [_ w308]
                      tunnel: w287 -> [w305 w307]
                      frame False {
                        n522 = xnode "Read/Write Control"("FPGA VI Reference In"=w305, "send can"=FALSE) -> ()  [unwired: 1 in, 2 out]
                      }
                      frame True {
                        n523 = disable-structure shown="Enabled" {
                          disable-tunnel: w308 -> [w313 _]
                          disable-tunnel: w307 -> [w309 _]
                          frame Enabled {
                            n524 = flat-sequence {
                              tunnel: w313 -> [w317]
                              tunnel: [w317] -> w312
                              tunnel: [w315] -> w311
                              tunnel: w309 -> [w314]
                              tunnel: w312 -> [w322]
                              tunnel: w311 -> [w320]
                              tunnel: [w319] -> w310
                              tunnel: w310 -> [w325]
                              frame #0 {
                                n525 = xnode "Read/Write Control"("FPGA VI Reference In"=w314, "send can"=TRUE) -> ("FPGA VI Reference Out"=w315:refnum<k20>)  [unwired: 1 in, 1 out]
                              }
                              frame #1 {
                                n526 = Bundle By Name(cluster=T3 {"timestamp high"=0, "timestamp low"=0, "identifier"=0, "type"=enum."Data Frame", "info A"=0, "info B"=0, "data length"=8, "data"=[0, 0, 0, 0, 0, 0, 0, 0]} ("Mod4/CAN1 input"), "identifier"=u32 912, "data"=w322, "data length"=u8 8) -> (w321:T3)
                                n527 = xnode "Read/Write Control"("FPGA VI Reference In"=w320, "Mod4/CAN1 input"=w321) -> ("FPGA VI Reference Out"=w319:refnum<k20>)  [unwired: 1 in, 1 out]
                              }
                              frame #2 {
                                n528 = disable-structure shown="Disabled" {
                                disable-tunnel: w325 -> [w327 _]
                                frame Disabled {
                                n529 = xnode "Read/Write Control"("FPGA VI Reference In"=w327, "send can"=FALSE) -> ()  [unwired: 1 in, 2 out]
                                }
                                frame Enabled {
                                }
                                }
                              }
                            }
                          }
                          frame Disabled {
                          }
                        }
                      }
                    }
                  }
                }
              }
            }
          }
          frame #3 {
            n530 = flat-sequence {
              frame #0 {
                n531 = global read "G_rio.vi" "VS_CAN"() -> (w399:dbl)
                n532 = local read "Ref vel"() -> (w398:dbl)
                n533 = call "T_control.vi"("Ref vel"=w398, "VS_CAN"=w399, "pid gain"=dbl[] [3.0, 0.0, 0.10000000000000003] ("pid gain 1")) -> ("Ref APS"=w401:dbl)  [unwired: 16 in]
                n534 = global write "G_rio.vi" "Ref APS"(w401) -> ()
              }
            }
            n535 = global read "G_rio.vi" "Auto"() -> (w345:bool)
            n536 = case shown="False" w345 {
              tunnel: [w347 w381] -> w346
              frame False {
                n537 = global read "G_rio.vi" "VS_CAN"() -> (w351:dbl)
                n538 = Absolute Value(x=w351) -> (abs(x)=w350:dbl)
                n539 = Less?(x=w350, y=0.05) -> (x < y?=w348:bool)
                n540 = case shown="True" w348 {
                  tunnel: [_ w354] -> w347
                  frame False {
                  }
                  frame True {
                    n541 = Sign(1:"Gear Manual") -> (0:w355:i32)
                    n542 = To Long Integer(number=w355) -> (32bit integer=w353:i32)
                    n543 = case shown="0" w353 {
                      tunnel: [w362 w366 w370] -> w354
                      frame 0 {
                        n544 = global read "G_rio.vi" "gear selector disp"() -> (w360:i8)
                        n545 = Equal To 0?(x=w360) -> (x = 0?=w359:bool)
                        n546 = Equal?(x=u8 7 ("y"), y=w360) -> (x = y?=w364:bool)
                        n547 = Select(t=-1.0, s=w359, f=1.0) -> (s? t:f=w358:dbl)
                        n548 = Select(t=0.0, s=w364, f=w358) -> (s? t:f=w362:dbl)
                      }
                      frame 1, Default {
                        n549 = global read "G_rio.vi" "gear selector disp"() -> (w369:i8)
                        n550 = Equal To 0?(x=w369) -> (x = 0?=w368:bool)
                        n551 = Select(t=0.0, s=w368, f=1.0 ("t")) -> (s? t:f=w366:dbl)
                      }
                      frame -1 {
                        n552 = global read "G_rio.vi" "gear selector disp"() -> (w371:i8)
                        n553 = case shown="3..5, Default" w371 {
                          tunnel: [-1.0 1.0 0.0] -> w370
                          frame 0, 6, 7 {
                          }
                          frame 1, 2 {
                          }
                          frame 3..5, Default {
                          }
                        }
                      }
                    }
                  }
                }
              }
              frame True {
                n554 = global read "G_rio.vi" "VS_CAN"() -> (w378:dbl)
                n555 = Absolute Value(x=w378) -> (abs(x)=w377:dbl)
                n556 = Less?(x=w377, y=0.05) -> (x < y?=w375:bool)
                n557 = global read "G_rio.vi" "Run"() -> (w380:bool)
                n558 = And(x=w375, y=w380) -> (x .and. y?=w379:bool)
                n559 = case shown="True" w379 {
                  tunnel: [_ w383] -> w381
                  frame False {
                  }
                  frame True {
                    n560 = local read "P, R, D"() -> (w382:i32)
                    n561 = case shown="-1" w382 {
                      tunnel: [w384 w389 w393] -> w383
                      frame -1 {
                        n562 = global read "G_rio.vi" "gear selector disp"() -> (w385:i8)
                        n563 = case shown="0" w385 {
                          tunnel: [-1.0 ("t") 1.0 ("t") _ _] -> w384
                          frame 0 {
                          }
                          frame 1, Default {
                          }
                          frame 4, 8 {
                          }
                          frame 7 {
                          }
                        }
                      }
                      frame 0, Default {
                        n564 = global read "G_rio.vi" "gear selector disp"() -> (w392:i8)
                        n565 = Equal To 0?(x=w392) -> (x = 0?=w391:bool)
                        n566 = Select(t=0.0, s=w391, f=1.0 ("t")) -> (s? t:f=w389:dbl)
                      }
                      frame 1 {
                        n567 = global read "G_rio.vi" "gear selector disp"() -> (w394:i8)
                        n568 = case shown="1, 2" w394 {
                          tunnel: [-1.0 1.0 0.0] -> w393
                          frame 0, 6, 7 {
                          }
                          frame 1, 2 {
                          }
                          frame 3..5, Default {
                          }
                        }
                      }
                    }
                  }
                }
              }
            }
            "shift lever" <- w346
          }
          frame #4 {
            n569 = flat-sequence {
              tunnel: [w407] -> w403
              tunnel: [w406] -> w402
              tunnel: w403 -> [w630]
              tunnel: w402 -> [w631]
              frame #0 {
                n570 = flat-sequence {
                  tunnel: [w463] -> w408
                  frame #0 {
                    n571 = global read "G_rio.vi" "accel pedal value"() -> (w455:dbl)
                    n572 = Equal To 0?(x=w455) -> (x = 0?=w454:bool)
                    n573 = case shown="True" w454 {
                      tunnel: [TRUE w466] -> w457
                      frame False {
                        n574 = global write "G_rio.vi" "T lim counter 2"(u16 300 ("T lim counter 2")) -> ()
                      }
                      frame True {
                        n575 = global read "G_rio.vi" "T lim counter 2"() -> (w468:u16)
                        n576 = Decrement(x=w468) -> (x-1=w469:u16)
                        n577 = Max & Min(x=u16 0, y=w469) -> (max(x,y)=w467:u16)  [unwired: 1 out]
                        n578 = global write "G_rio.vi" "T lim counter 2"(w467) -> ()
                        n579 = Not Equal To 0?(x=w467) -> (x != 0?=w466:bool)
                      }
                    }
                    n580 = global read "G_rio.vi" "brake_act_can"() -> (w456:bool)
                    n581 = global read "G_rio.vi" "Throttle_Enable"() -> (w460:bool)
                    n582 = local read "Ref vel"() -> (w453:dbl)
                    n583 = Not Equal To 0?(x=w453) -> (x != 0?=w462:bool)
                    n584 = Not(x=w456) -> (.not. x?=w461:bool)
                    n585 = global read "G_rio.vi" "Auto"() -> (w458:bool)
                    n586 = global read "G_rio.vi" "Run"() -> (w459:bool)
                    n587 = Compound Arithmetic op=AND(w458, w459, w462, w461, w460, w457) -> (w463:bool)
                  }
                }
                n588 = global read "G_rio.vi" "Auto"() -> (w404:bool)
                n589 = case shown="True" w404 {
                  tunnel: [1000.0 ("f") w413] -> w405
                  frame False {
                  }
                  frame True {
                    n590 = global read "G_rio.vi" "VS_CAN"() -> (w411:dbl)
                    n591 = local read "Ref vel"() -> (w416:dbl)
                    n592 = Subtract(x=w416, y=w411) -> (x-y=w415:dbl)
                    n593 = Less?(x=w415, y=-2.0 ("lower limit")) -> (x < y?=w417:bool)
                    n594 = case shown="True" w417 {
                      tunnel: w415 -> [w420 w450]
                      tunnel: [w421 w440] -> w414
                      tunnel: w416 -> [w425 w441]
                      frame False {
                        n595 = Equal To 0?(x=w425) -> (x = 0?=w424:bool)
                        n596 = global read "G_rio.vi" "PWM Brake"() -> (w419:dbl)
                        n597 = Greater?(x=w420, y=1.0) -> (0:w429:bool)
                        n598 = Multiply(x=w419, y=0.999) -> (x*y=w431:dbl)
                        n599 = Max & Min(x=w431, y=1000.0) -> (max(x,y)=w427:dbl)  [unwired: 1 out]
                        n600 = Select(t=1000.0, s=w429, f=w427) -> (s? t:f=w422:dbl)
                        n601 = Select(t=2000.0, s=w424, f=w422) -> (s? t:f=w421:dbl)
                      }
                      frame True {
                        w438 = 0.5 ("gain brake")
                        w447 = 10.0 ("y")
                        n602 = Absolute Value(x=w450) -> (abs(x)=w449:dbl)
                        n603 = Add(x=w449, y=w447) -> (x+y=w448:dbl)
                        n604 = Multiply(x=w448, y=w447) -> (x*y=w446:dbl)
                        n605 = Threshold 1D Array(2:w446, 3:dbl[] [10.0, 15.0, 25.0, 50.0, 80.0, 120.0, 170.0, 230.0, 290.0, 350.0, 420.0]) -> (0:w444:dbl)  [unwired: 1 in]
                        n606 = global read "G_rio.vi" "PWM Brake"() -> (w433:dbl)
                        n607 = Interpolate 1D Array(1:w444, 2:dbl[] [1000.0, 1100.0, 1200.0, 1300.0, 1400.0, 1500.0, 1600.0, 1700.0, 1800.0, 1900.0, 2000.0]) -> (0:w439:dbl)
                        n608 = Decrement(x=w438) -> (x-1=w437:dbl)
                        n609 = Multiply(x=w439, y=w438) -> (x*y=w435:dbl)
                        n610 = Multiply(x=w437, y=w433) -> (x*y=w436:dbl)
                        n611 = Subtract(x=w435, y=w436) -> (x-y=w434:dbl)
                        n612 = Equal To 0?(x=w441) -> (x = 0?=w442:bool)
                        n613 = Select(t=2000.0, s=w442, f=w434) -> (s? t:f=w440:dbl)
                      }
                    }
                    n614 = global read "G_rio.vi" "Run"() -> (w410:bool)
                    n615 = Select(t=w414, s=w410, f=2000.0) -> (s? t:f=w413:dbl)
                  }
                }
                n616 = case shown="True" w408 {
                  tunnel: [_ TRUE] -> w407
                  tunnel: [w471 w490] -> w406
                  frame False {
                    n617 = flat-sequence {
                      tunnel: [w481] -> w471
                      frame #0 {
                        n618 = global read "G_rio.vi" "T Lim"() -> (w472:bool)
                        n619 = case shown="True" w472 {
                          selector: w472 -> [_ w479]
                          frame False {
                            n620 = global write "G_rio.vi" "T lim counter"(u16 0 ("T lim counter")) -> ()
                          }
                          frame True {
                            n621 = global write "G_rio.vi" "T lim once"(w479) -> ()
                            n622 = global write "G_rio.vi" "T lim counter 2"(u16 300 ("T lim counter 2")) -> ()
                            n623 = global read "G_rio.vi" "T lim counter"() -> (w478:u16)
                            n624 = Increment(x=w478) -> (x+1=w477:u16)
                            n625 = Max & Min(x=u16 100, y=w477) -> (min(x,y)=w476:u16)  [unwired: 1 out]
                            n626 = global write "G_rio.vi" "T lim counter"(w476) -> ()
                          }
                        }
                      }
                      frame #1 {
                        n627 = global read "G_rio.vi" "T lim once"() -> (w480:bool)
                        n628 = case shown="True" w480 {
                          tunnel: [-1.0 ("t") w486] -> w481
                          frame False {
                          }
                          frame True {
                            n629 = global read "G_rio.vi" "T lim counter"() -> (w485:u16)
                            n630 = Equal?(x=w485, y=u16 100) -> (x = y?=w484:bool)
                            n631 = Select(t=0.0, s=w484, f=-0.15) -> (s? t:f=w486:dbl)
                          }
                        }
                        n632 = global write "G_rio.vi" "Throttle_Enable"(w480) -> ()
                      }
                    }
                  }
                  frame True {
                    n633 = disable-structure shown="Enabled" {
                      disable-tunnel: [w509 w565] -> w490
                      frame Enabled {
                        n634 = global read "G_rio.vi" "accel pedal value"() -> (w513:dbl)
                        n635 = global read "G_rio.vi" "Ref APS"() -> (w514:dbl)
                        n636 = global read "G_rio.vi" "accel pedal value"() -> (w512:dbl)
                        n637 = global read "G_rio.vi" "accel pedal value"() -> (w501:dbl)
                        n638 = Subtract(x=w514, y=w513) -> (x-y=w500:dbl)
                        n639 = flat-sequence {
                          tunnel: w500 -> [w535]
                          tunnel: [w532] -> w508
                          frame #0 {
                            n640 = feedback #15(0.0) -> (w540:dbl)
                            n641 = feedback-in #15(w535) -> ()
                            n642 = Multiply(x=w535, y=0.01) -> (x*y=w536:dbl)
                            n643 = Subtract(x=w535, y=w540) -> (x-y=w539:dbl)
                            n644 = feedback #16(0.0) -> (w531:dbl)
                            n645 = Multiply(x=0.999, y=w531) -> (x*y=w530:dbl)
                            n646 = Divide(x=w539, y=0.01) -> (x/y=w526:dbl)
                            n647 = Add(x=w536, y=w530) -> (x+y=w527:dbl)
                            n648 = feedback-in #16(w527) -> ()
                            n649 = Build Array(w535, w527, w526) -> (w534:dbl[])
                            n650 = Multiply(x=w534, y=dbl[] [8.0, 0.02, 0.4] ("pid gain 2")) -> (x*y=w533:dbl[])
                            n651 = Add Array Elements(numeric array=w533) -> (sum=w532:dbl)
                          }
                        }
                        n652 = Greater Than 0?(x=w500) -> (x > 0?=w502:bool)
                        n653 = Less Than 0?(x=w500) -> (x < 0?=w494:bool)
                        n654 = Equal To 0?(x=w501) -> (x = 0?=w493:bool)
                        n655 = Greater?(x=w512, y=95.0) -> (0:w503:bool)
                        n656 = And(x=w503, y=w502) -> (x .and. y?=w498:bool)
                        n657 = And(x=w493, y=w494) -> (x .and. y?=w499:bool)
                        n658 = Or(x=w498, y=w499) -> (x .or. y?=w497:bool)
                        n659 = Multiply(x=w508, y=0.01) -> (x*y=w506:dbl)
                        n660 = In Range and Coerce(upper limit=1.0 ("x"), x=w506, lower limit=-1.0) -> (coerced(x)=w496:dbl)  [unwired: 1 out]
                        n661 = flat-sequence {
                          tunnel: w496 -> [w516]
                          tunnel: [w522] -> w495
                          frame #0 {
                            w515 = 0.5 ("x")
                            n662 = Multiply(x=w516, y=w515) -> (x*y=w520:dbl)
                            n663 = Subtract(x=1.0, y=w515) -> (x-y=w518:dbl)
                            n664 = feedback #17(0.0) -> (w517:dbl)
                            n665 = Multiply(x=w518, y=w517) -> (x*y=w519:dbl)
                            n666 = Add(x=w520, y=w519) -> (x+y=w522:dbl)
                            n667 = feedback-in #17(w522) -> ()
                          }
                        }
                        n668 = Select(t=0.0 ("f"), s=w497, f=w495) -> (s? t:f=w509:dbl)
                      }
                      frame Disabled {
                        n669 = global read "G_rio.vi" "VS_CAN"() -> (w567:dbl)
                        n670 = global read "G_rio.vi" "VS_CAN"() -> (w553:dbl)
                        n671 = local read "Ref vel"() -> (w568:dbl)
                        n672 = Divide(x=w553, y=3.6) -> (x/y=w551:dbl)
                        n673 = Subtract(x=w568, y=w567) -> (x-y=w546:dbl)
                        n674 = feedback #18(0.0 ("y")) -> (w558:dbl)
                        n675 = feedback-in #18(w551) -> ()
                        n676 = Subtract(x=w551, y=w558) -> (x-y=w557:dbl)
                        n677 = Divide(x=w546, y=3.6) -> (x/y=w542:dbl)
                        n678 = Divide(x=dbl[] [-100.0, -3.0, -1.0, 1.0, 3.0, 100.0] ("array_x"), y=3.6) -> (x/y=w543:dbl[])
                        n679 = call "lookuptable.vi"("array_y"=dbl[] [-0.5, -0.1, -0.01, 0.01, 0.1, 0.5] ("array_x"), "array_x"=w543, "x"=w542) -> ("y"=w561:dbl)  [unwired: 8 in]
                        n680 = Multiply(x=100.0, y=w557) -> (x*y=w555:dbl)
                        n681 = Multiply(x=1.0 ("P_gain"), y=w561) -> (x*y=w550:dbl)
                        n682 = Multiply(x=0.0 ("D_gain"), y=w555) -> (x*y=w549:dbl)
                        n683 = Subtract(x=w550, y=w549) -> (x-y=w548:dbl)
                        n684 = flat-sequence {
                          tunnel: w548 -> [w570]
                          tunnel: [w569] -> w541
                          frame #0 {
                            n685 = feedback #19(0.0 ("y")) -> (w577:dbl)
                            n686 = Multiply(x=-0.01, y=999.0) -> (x*y=w576:dbl)
                            n687 = Multiply(x=0.7 ("Rate"), y=0.01 ("x")) -> (x*y=w572:dbl)
                            n688 = Add(x=w577, y=w576) -> (x+y=w578:dbl)
                            n689 = Add(x=w572, y=w577) -> (x+y=w579:dbl)
                            n690 = In Range and Coerce(upper limit=w579, x=w570, lower limit=w578) -> (coerced(x)=w569:dbl)  [unwired: 1 out]
                            n691 = feedback-in #19(w569) -> ()
                          }
                        }
                        n692 = In Range and Coerce(upper limit=1.0, x=w541, lower limit=-1.0) -> (coerced(x)=w562:dbl)  [unwired: 1 out]
                        n693 = flat-sequence {
                          tunnel: w562 -> [w582]
                          tunnel: [w581] -> w565
                          frame #0 {
                            n694 = Greater Than 0?(x=w582) -> (x > 0?=w590:bool)
                            n695 = global read "G_rio.vi" "accel pedal value"() -> (w593:dbl)
                            n696 = global read "G_rio.vi" "accel pedal value"() -> (w589:dbl)
                            n697 = Less Than 0?(x=w582) -> (x < 0?=w588:bool)
                            n698 = Equal To 0?(x=w589) -> (x = 0?=w587:bool)
                            n699 = Greater?(x=w593, y=95.0) -> (0:w591:bool)
                            n700 = And(x=w591, y=w590) -> (x .and. y?=w586:bool)
                            n701 = And(x=w588, y=w587) -> (x .and. y?=w585:bool)
                            n702 = Or(x=w586, y=w585) -> (x .or. y?=w584:bool)
                            n703 = Select(t=0.0, s=w584, f=w582) -> (s? t:f=w581:dbl)
                          }
                        }
                      }
                    }
                    n704 = global write "G_rio.vi" "T lim counter"(u16 0 ("T lim counter")) -> ()
                    n705 = global write "G_rio.vi" "T lim once"(FALSE ("T lim once")) -> ()
                  }
                }
                n706 = disable-structure shown="Enabled" {
                  disable-tunnel: w405 -> [w452 _]
                  frame Enabled {
                    n707 = global write "G_rio.vi" "PWM Brake"(w452) -> ()
                  }
                  frame Disabled {
                  }
                }
              }
              frame #1 {
                n708 = local read "shift lever"() -> (w610:dbl)
                n709 = disable-structure shown="Enabled" {
                  disable-tunnel: [w632 w637] -> w599
                  frame Disabled {
                    n710 = global read "G_rio.vi" "accel pedal value"() -> (w635:dbl)
                    n711 = global read "G_rio.vi" "Ref APS"() -> (w636:dbl)
                    n712 = Equal To 0?(x=w636) -> (x = 0?=w633:bool)
                    n713 = Not Equal To 0?(x=w635) -> (x != 0?=w634:bool)
                    n714 = And(x=w633, y=w634) -> (x .and. y?=w632:bool)
                  }
                  frame Enabled {
                    n715 = global read "G_rio.vi" "accel pedal value"() -> (w638:dbl)
                    n716 = global read "G_rio.vi" "Ref APS"() -> (w639:dbl)
                    n717 = Subtract(x=w638, y=w639) -> (x-y=w640:dbl)
                    n718 = Greater?(x=w640, y=5.0) -> (0:w637:bool)
                  }
                }
                n719 = Multiply(x=w631, y=500.0 ("T gain")) -> (x*y=w628:dbl)
                n720 = disable-structure shown="Enabled" {
                  disable-tunnel: [w649 _] -> w609
                  frame Enabled {
                    n721 = global read "G_rio.vi" "Auto"() -> (w653:bool)
                    n722 = global read "G_rio.vi" "Run"() -> (w652:bool)
                    n723 = Compound Arithmetic op=AND(w653, w652) -> (w651:bool)
                    n724 = And(x=w651, y="buzz") -> (x .and. y?=w649:bool)
                  }
                  frame Disabled {
                  }
                }
                n725 = Multiply(x=w610, y=250.0 ("S gain")) -> (x*y=w618:dbl)
                n726 = In Range and Coerce(upper limit=500.0, x=w628, lower limit=-500.0) -> (coerced(x)=w612:dbl)  [unwired: 1 out]
                n727 = global read "G_rio.vi" "PWM Brake"() -> (w605:dbl)
                n728 = global read "G_rio.vi" "PWM Brake"() -> (w607:dbl)
                n729 = In Range and Coerce(upper limit=500.0, x=w618, lower limit=-500.0) -> (coerced(x)=w621:dbl)  [unwired: 1 out]
                n730 = global read "G_rio.vi" "mdps torque"() -> (w597:dbl)
                n731 = Add(x=w612, y=1500.0) -> (x+y=w624:dbl)
                n732 = global read "G_rio.vi" "brake_act_can"() -> (w602:bool)
                n733 = global read "G_rio.vi" "brake release"() -> (w601:bool)
                n734 = Equal?(x=w605, y=1000.0) -> (x = y?=w603:bool)
                n735 = Add(x=w621, y=1500.0) -> (x+y=w623:dbl)
                n736 = Select(t=w607, s="brake", f="Slide") -> (s? t:f=w606:dbl)
                n737 = Absolute Value(x=w597) -> (abs(x)=w594:dbl)
                "mdps torque" <- w594
                n738 = To Unsigned Word Integer(number=w624) -> (unsigned 16bit integer=w608:u16)
                "T PWM" <- w608
                n739 = Compound Arithmetic op=AND(w603, w602, w601) -> (w600:bool)
                n740 = To Unsigned Word Integer(number=w623) -> (unsigned 16bit integer=w611:u16)
                n741 = To Unsigned Word Integer(number=w606) -> (unsigned 16bit integer=w615:u16)
                "B PWM" <- w615
                n742 = Greater?(x=w594, y=5.0) -> (0:w595:bool)
                n743 = local read "FPGA"() -> (w616:refnum<k20>)
                n744 = Compound Arithmetic op=OR(w595, w600, w599) -> (w598:bool)
                n745 = case shown="True" w598 {
                  frame False {
                    n746 = global write "G_rio.vi" "Auto SW counter"(u16 0 ("Auto SW counter")) -> ()
                  }
                  frame True {
                    w645 = u16 40 ("x")
                    n747 = global read "G_rio.vi" "Auto SW counter"() -> (w647:u16)
                    n748 = Increment(x=w647) -> (x+1=w646:u16)
                    n749 = Max & Min(x=w645, y=w646) -> (min(x,y)=w644:u16)  [unwired: 1 out]
                    n750 = Equal?(x=w645, y=w644) -> (x = y?=w643:bool)
                    n751 = global write "G_rio.vi" "Auto SW counter"(w644) -> ()
                    n752 = case shown="True" w643 {
                      frame False {
                      }
                      frame True {
                        n753 = global write "G_rio.vi" "Auto SW"(FALSE ("Auto SW")) -> ()
                      }
                    }
                  }
                }
                n754 = xnode "Read/Write Control"("FPGA VI Reference In"=w616, "Buzz"=w609, "S Pwm 1"=w611, "S Pwm 2"=w611, "B Pwm"=w615, "T Pwm"=w608, "Solenoid"=w630) -> ()  [unwired: 1 in, 2 out]
                "solenoid" <- w630
              }
              frame #2 {
                n755 = local read "LCM"() -> (w654:bool)
                n756 = case shown="True" w654 {
                  frame False {
                    n757 = global read "G_rio.vi" "Auto"() -> (w655:bool)
                    n758 = global read "G_rio.vi" "Run"() -> (w656:bool)
                    n759 = global read "G_rio.vi" "VS_CAN"() -> (w658:dbl)
                    n760 = global read "G_rio.vi" "mdps str_ang"() -> (w657:dbl)
                    n761 = shared-variable "veloster\\sharedvari.lvlib\\run"(w656) -> ()  [unwired: 1 in, 1 out]
                    n762 = shared-variable "veloster\\sharedvari.lvlib\\auto"(w655) -> ()  [unwired: 1 in, 1 out]
                    n763 = shared-variable "veloster\\sharedvari.lvlib\\vs_can"(w658) -> ()  [unwired: 1 in, 1 out]
                    n764 = shared-variable "veloster\\sharedvari.lvlib\\steer_output"(w657) -> ()  [unwired: 1 in, 1 out]
                  }
                  frame True {
                    n765 = Get Date/Time In Seconds() -> (seconds since 1Jan1904=w663:timestamp)
                    n766 = global read "G_rio.vi" "LCM_CON_T"() -> (w682:T10)
                    n767 = To Double Precision Float(number=w663) -> (double precision float=w662:dbl)
                    n768 = Unbundle By Name(w682) -> ("hash"=w680:i64)
                    n769 = Multiply(x=w662, y=1000000.0) -> (x*y=w660:dbl)
                    n770 = global read "G_rio.vi" "Ref Brk Enc"() -> (w666:dbl)
                    n771 = local read "solenoid"() -> (w671:bool)
                    n772 = local read "Ref steer"() -> (w664:dbl)
                    n773 = global read "G_rio.vi" "Ref APS"() -> (w665:dbl)
                    n774 = local read "brk enc"() -> (w670:u8)
                    n775 = local read "B PWM"() -> (w669:u16)
                    n776 = local read "T PWM"() -> (w668:u16)
                    n777 = To Quad Integer(1:w660) -> (0:w659:i64)
                    n778 = call "hash.vi"("input"=w680) -> ("output"=w679:i64)  [unwired: 10 in]
                    n779 = local read "Ref vel"() -> (w667:dbl)
                    n780 = global read "G_rio.vi" "T Lim"() -> (w672:bool)
                    n781 = global read "G_rio.vi" "Auto"() -> (w674:bool)
                    n782 = global read "G_rio.vi" "Run"() -> (w673:bool)
                    n783 = Bundle(cluster=w682, "hash"=w679, "sys time"=w659, "Auto"=w674, "Run"=w673, "Solenoid"=w671, "T lim"=w672, "brk_enc"=w670, "B PWM"=w669, "T PWM"=w668, "ref_vel"=w667, "ref_bkr_enc"=w666, "ref_apv"=w665, "ref_steer"=w664) -> (w675:T10)
                    n784 = Flatten To String(anything=w675, prepend array or string size? (T)=FALSE) -> (data string=w677:string)  [unwired: 2 in, 2 out]
                    n785 = global read "G_rio.vi" "LCM"() -> (w676:T4)
                    n786 = call "LCM_send.vi"("DATA"=w677, "ID"="CON_T", "LCM"=w676) -> ()  [unwired: 7 in, 2 out]
                  }
                }
              }
            }
          }
        }
      }
    }
  }
  n787 = flat-sequence {
    tunnel: [dbl[] [0.0, 0.0, 0.0, 0.0, 0.0] ("pos(i)")] -> w1
    tunnel: w1 -> [w1134]
    frame #0 {
      w1130 = FALSE ("get heading")
      w1133 = u64 1
      w1132 = 0.0 ("dh_hat")
      n788 = local write "GPS init"(w1130) -> ()
      n789 = call "getecefdcmref.vi"("map name"="map name") -> ("XYZ"=→"ecef ref":dbl[])  [unwired: 10 in, 4 out]
      "vgain" <- 1.0 ("initH")
      "vcount" <- w1133
      "hbias" <- 0.02314872284554697 ("hbias")
      "hcount" <- w1133
      "get heading" <- w1130
      "get position" <- w1130
      "heading error" <- w1132
      "h_gps" <- w1132
      "rt" <- w1132
      "pos error" <- w1132
      "map" <- "map name"
    }
    frame #1 {
      n790 = disable-structure shown="Enabled" {
        frame Disabled {
          n791 = while {
            stop <- FALSE stop-if-true
            n792 = flat-sequence {
              frame #0 {
                n793 = Wait Until Next ms Multiple(millisecond multiple=u32 50) -> ()  [unwired: 1 out]
              }
              frame #1 {
                n794 = local read item#-1() -> (w1139)
                n795 = xnode "Read/Write Control"("FPGA VI Reference In"=w1139) -> ("FPGA VI Reference Out"=w1137:refnum<k20>, "Connection error GPS 1"=w1138:bool)  [unwired: 1 in, 1 out]
                n796 = case shown="False" w1138 {
                  tunnel: w1137 -> [w1141 w1261]
                  frame False {
                    n797 = flat-sequence {
                      tunnel: w1141 -> [w1143]
                      tunnel: [w1142] -> w1140
                      tunnel: w1140 -> [w1162]
                      frame #0 {
                        n798 = while {
                          tunnel: w1143 -> [w1147]
                          tunnel: [w1145] -> w1142
                          stop <- w1146 stop-if-true
                          n799 = flat-sequence {
                            tunnel: w1147 -> [w1149]
                            tunnel: [w1149] -> w1144
                            tunnel: [w1152] -> w1146
                            tunnel: [w1151] -> w1145
                            tunnel: w1144 -> [w1158]
                            frame #0 {
                              n800 = Wait Until Next ms Multiple(millisecond multiple=u32 20) -> ()  [unwired: 1 out]
                            }
                            frame #1 {
                              n801 = xnode "Invoke Method"("FPGA VI Reference In"=w1158, "Number of Elements"=u32 1, "Timeout (ms)"=1) -> ("FPGA VI Reference Out"=w1151:refnum<k20>, "Data"=w1153:u8[])  [unwired: 1 in, 2 out]
                              n802 = Index Array(array=w1153, index=0) -> (element=w1155:u8)
                              n803 = Equal?(x=w1155, y=u8 170) -> (x = y?=w1152:bool)
                            }
                          }
                        }
                      }
                      frame #1 {
                        w1163 = u32 3 ("Number of Elements")
                        n804 = xnode "Invoke Method"("FPGA VI Reference In"=w1162, "Number of Elements"=w1163, "Timeout (ms)"=w1163) -> ("FPGA VI Reference Out"=w1161:refnum<k20>, "Data"=w1165:u8[], "Elements Remaining"=w1159:u32)  [unwired: 1 in, 1 out]
                        n805 = Equal?(x=w1165, y=u8[] [68, 18, 28]) -> (x = y?=w1166:bool[])
                        n806 = And Array Elements(Boolean array=w1166) -> (logical AND=w1160:bool)
                        n807 = case shown="True" w1160 {
                          tunnel: w1161 -> [w1169 w1174]
                          tunnel: w1159 -> [w1168 _]
                          frame False {
                            n808 = xnode "Invoke Method"("FPGA VI Reference In"=w1169, "Number of Elements"=w1168, "Timeout (ms)"=1) -> ()  [unwired: 1 in, 4 out]
                          }
                          frame True {
                            w1170 = u32 8 ("Number of Elements")
                            n809 = xnode "Invoke Method"("FPGA VI Reference In"=w1174, "Number of Elements"=w1170, "Timeout (ms)"=w1170) -> ("FPGA VI Reference Out"=w1187:refnum<k20>, "error out"=w1188:errorcluster, "Data"=w1190:u8[])  [unwired: 1 in, 1 out]
                            n810 = Index Array(array=w1190, index #1=1 ("index"), index #2=0 ("index"), index #3=5 ("index"), index #4=4 ("index")) -> (element #1=w1177:u8, element #2=w1178:u8, element #3=w1182:u8, element #4=w1183:u8)
                            n811 = Join Numbers(hi=w1182, lo=w1183) -> ((hi.lo)=w1184:u16)
                            n812 = Join Numbers(hi=w1177, lo=w1178) -> ((hi.lo)=w1179:u16)
                            n813 = Add(x=w1184, y=u16 20) -> (x+y=w1186:u16)
                            n814 = xnode "Invoke Method"("FPGA VI Reference In"=w1187, "error in"=w1188, "Number of Elements"=w1186, "Timeout (ms)"=10) -> ("Data"=w1172:u8[])  [unwired: 3 out]
                            n815 = Empty Array?(array=w1172) -> (empty?=w1171:bool)
                            n816 = Build Array (concatenate)(u8[] [170, 68, 18, 28], w1190, w1172) -> (w1191:u8[])
                            n817 = case shown="False" w1171 {
                              tunnel: w1191 -> [w1193 _]
                              tunnel: w1179 -> [w1192 _]
                              frame False {
                                n818 = case shown="99" w1192 {
                                tunnel: w1193 -> [_ w1196 w1234]
                                frame 0, Default {
                                }
                                frame 42 {
                                n819 = local read "ecef ref"() -> (w1195:dbl[])
                                n820 = call "novatel_bestpos.vi"("ecef ref"=w1195, "gps_data"=w1196) -> ("LCC"=w1194:dbl[])  [unwired: 9 in]
                                n821 = flat-sequence {
                                tunnel: w1194 -> [w1199]
                                frame #0 {
                                n822 = Index Array(array=w1199, index=1) -> (element=w1202:dbl)
                                n823 = Not Equal To 0?(x=w1202) -> (x != 0?=w1198:bool)
                                n824 = local read "LCM"() -> (w1201:bool)
                                n825 = And(x=w1198, y=w1201) -> (x .and. y?=w1197:bool)
                                n826 = case shown="True" w1197 {
                                tunnel: w1199 -> [_ w1222]
                                frame False {
                                }
                                frame True {
                                n827 = Get Date/Time In Seconds() -> (seconds since 1Jan1904=w1207:timestamp)
                                n828 = To Double Precision Float(number=w1207) -> (double precision float=w1206:dbl)
                                n829 = global read "G_rio.vi" "LCM_GGA_T"() -> (w1231:T12)
                                n830 = Array To Cluster(array=w1222) -> (cluster=w1230:T13)
                                n831 = Unbundle By Name(w1231) -> ("hash"=w1227:i64)
                                n832 = Multiply(x=w1206, y=1000000.0) -> (x*y=w1204:dbl)
                                n833 = Unbundle(w1230) -> ("LCC[0]"=w1232:dbl, "LCC[2]"=w1221:dbl, "LCC[3]"=w1220:dbl, "LCC[4]"=w1219:dbl, "LCC[6]"=w1218:dbl, "LCC[7]"=w1216:dbl, "LCC[8]"=w1214:dbl, "LCC[9]"=w1212:dbl, "LCC[12]"=w1211:dbl, "LCC[13]"=w1210:dbl, "LCC[14]"=w1209:dbl)  [unwired: 4 out]
                                n834 = To Quad Integer(1:w1204) -> (0:w1203:i64)
                                n835 = To Long Integer(number=w1218) -> (32bit integer=w1217:i32)
                                n836 = To Long Integer(number=w1216) -> (32bit integer=w1215:i32)
                                n837 = To Long Integer(number=w1214) -> (32bit integer=w1213:i32)
                                n838 = call "hash.vi"("input"=w1227) -> ("output"=w1226:i64)  [unwired: 10 in]
                                n839 = local read "map"() -> (w1208:i32)
                                n840 = Bundle(cluster=w1231, "hash"=w1226, "sys time"=w1203, "time"=w1232, "x"=w1221, "y"=w1220, "h"=w1219, "numSV"=w1217, "postype"=w1215, "lag"=w1213, "hordev"=w1212, "lat"=w1211, "lon"=w1210, "hgt"=w1209, "map_idx"=w1208) -> (w1228:T12)
                                n841 = Flatten To String(anything=w1228, prepend array or string size? (T)=FALSE) -> (data string=w1224:string)  [unwired: 2 in, 2 out]
                                n842 = global read "G_rio.vi" "LCM"() -> (w1223:T4)
                                n843 = call "LCM_send.vi"("DATA"=w1224, "ID"="GGA_DGPS", "LCM"=w1223) -> ()  [unwired: 7 in, 2 out]
                                }
                                }
                                }
                                }
                                n844 = global write "G_rio.vi" "dgps_pos"(w1194) -> ()
                                }
                                frame 99 {
                                n845 = call "novatel_bestvel.vi"("gps_data"=w1234) -> ("vel"=w1233:dbl[])  [unwired: 10 in]
                                n846 = flat-sequence {
                                tunnel: w1233 -> [w1236]
                                frame #0 {
                                n847 = Index Array(array=w1236, index=1) -> (element=w1239:dbl)
                                n848 = Not Equal To 0?(x=w1239) -> (x != 0?=w1240:bool)
                                n849 = local read "LCM"() -> (w1238:bool)
                                n850 = And(x=w1240, y=w1238) -> (x .and. y?=w1235:bool)
                                n851 = case shown="True" w1235 {
                                tunnel: w1236 -> [_ w1259]
                                frame False {
                                }
                                frame True {
                                n852 = Get Date/Time In Seconds() -> (seconds since 1Jan1904=w1245:timestamp)
                                n853 = To Double Precision Float(number=w1245) -> (double precision float=w1244:dbl)
                                n854 = global read "G_rio.vi" "LCM_RMC_T"() -> (w1260:T14)
                                n855 = Unbundle By Name(w1260) -> ("hash"=w1256:i64)
                                n856 = Multiply(x=w1244, y=1000000.0) -> (x*y=w1242:dbl)
                                n857 = Array To Cluster(array=w1259) -> (cluster=w1258:T15)
                                n858 = To Quad Integer(1:w1242) -> (0:w1241:i64)
                                n859 = call "hash.vi"("input"=w1256) -> ("output"=w1255:i64)  [unwired: 10 in]
                                n860 = Unbundle(w1258) -> ("vel[0]"=w1250:dbl, "vel[2]"=w1249:dbl, "vel[4]"=w1248:dbl, "vel[5]"=w1247:dbl, "vel[6]"=w1246:dbl)  [unwired: 2 out]
                                n861 = Bundle(cluster=w1260, "hash"=w1255, "sys time"=w1241, "time"=w1250, "speed"=w1249, "heading"=w1248, "lat"=w1247, "lon"=w1246) -> (w1251:T14)
                                n862 = Flatten To String(anything=w1251, prepend array or string size? (T)=FALSE) -> (data string=w1253:string)  [unwired: 2 in, 2 out]
                                n863 = global read "G_rio.vi" "LCM"() -> (w1252:T4)
                                n864 = call "LCM_send.vi"("DATA"=w1253, "ID"="RMC_1", "LCM"=w1252) -> ()  [unwired: 7 in, 2 out]
                                }
                                }
                                }
                                }
                                n865 = global write "G_rio.vi" "dgps_vel"(w1233) -> ()
                                }
                                }
                              }
                              frame True {
                              }
                            }
                          }
                        }
                      }
                    }
                  }
                  frame True {
                    n866 = xnode "Invoke Method"("FPGA VI Reference In"=w1261, "Number of Elements"=u32 1, "Timeout (ms)"=5) -> ("FPGA VI Reference Out"=w1265:refnum<k20>, "error out"=w1266:errorcluster, "Elements Remaining"=w1267:u32)  [unwired: 1 in, 1 out]
                    n867 = xnode "Invoke Method"("FPGA VI Reference In"=w1265, "error in"=w1266, "Number of Elements"=w1267, "Timeout (ms)"=5) -> ()  [unwired: 4 out]
                  }
                }
              }
            }
          }
        }
        frame Disabled {
          n868 = while {
            stop <- FALSE stop-if-true
            n869 = flat-sequence {
              frame #0 {
                n870 = Wait Until Next ms Multiple(millisecond multiple=u32 100) -> (millisecond timer value=w1269:u32)
                n871 = flat-sequence {
                  tunnel: w1269 -> [w1272]
                  frame #0 {
                    n872 = feedback #20(w1272) -> (w1273:u32)
                    n873 = feedback-in #20(w1272) -> ()
                    n874 = Subtract(x=w1272, y=w1273) -> (x-y=→"GPS_novatel_time":u32)
                  }
                }
              }
              frame #1 {
                n875 = local read item#-1() -> (w1276)
                n876 = xnode "Read/Write Control"("FPGA VI Reference In"=w1276) -> ("FPGA VI Reference Out"=w1275:refnum<k20>, "error out"=w1274:errorcluster)  [unwired: 1 in, 1 out]
                n877 = flat-sequence {
                  tunnel: w1275 -> [w1287]
                  tunnel: w1274 -> [w1286]
                  frame #0 {
                    n878 = xnode "Invoke Method"("FPGA VI Reference In"=w1287, "error in"=w1286, "Number of Elements"=u32 0, "Timeout (ms)"=10) -> ("FPGA VI Reference Out"=w1285:refnum<k20>, "error out"=w1284:errorcluster, "Elements Remaining"=w1283:u32)  [unwired: 1 out]
                    n879 = xnode "Invoke Method"("FPGA VI Reference In"=w1285, "error in"=w1284, "Number of Elements"=w1283) -> ("Data"=w1277:u8[])  [unwired: 1 in, 3 out]
                    n880 = local read "rest"() -> (w1279:u8[])
                    n881 = Build Array (concatenate)(w1279, w1277) -> (w1278:u8[])
                    n882 = Empty Array?(array=w1278) -> (empty?=w1280:bool)
                    n883 = case shown="False" w1280 {
                      tunnel: w1278 -> [w1290 _]
                      frame False {
                        n884 = for {
                          N: 2 -> [_]
                          shift-right: [w1294] -> w1288
                          shift-left: w1290 -> [w1292]
                          n885 = for {
                            tunnel: w1292 -> [w1405]
                            tunnel: u8[] [170, 68, 18, 28] -> [w1403] mode=indexing
                            shift-right: [w1402] -> _
                            shift-left: 0 ("start index (0)") -> [w1404]
                            tunnel: [w1402] -> w1301 mode=indexing
                            n886 = Search 1D Array(1D array=w1405, element=w1403, start index (0)=w1404) -> (index of element=w1402:i32)
                          }
                          n887 = Index Array(array=w1301, index #1=3 ("index"), index #2=0 ("index")) -> (element #1=w1298:i32, element #2=w1291:i32)
                          n888 = Subtract(x=w1298, y=w1291) -> (x-y=w1297:i32)
                          n889 = Array Subset(array=w1292, index=w1291) -> (w1293:u8[])  [unwired: 1 in]
                          n890 = Equal?(x=3, y=w1297) -> (x = y?=w1295:bool)
                          n891 = case shown="True" w1295 {
                            tunnel: w1293 -> [w1307 w1316]
                            tunnel: [w1306 w1313] -> w1294
                            tunnel: w1291 -> [w1305 _]
                            frame False {
                              n892 = Greater Or Equal To 0?(x=w1305) -> (x >= 0?=w1304:bool)
                              n893 = case shown="False" w1304 {
                                tunnel: w1307 -> [w1308 w1311]
                                tunnel: [w1308 w1309] -> w1306
                                frame False {
                                }
                                frame True {
                                n894 = Array Subset(array=w1311, index=1 ("length")) -> (w1309:u8[])  [unwired: 1 in]
                                }
                              }
                            }
                            frame True {
                              w1312 = 4 ("index")
                              n895 = Array Size(array=w1316) -> (size(s)=w1318:i32)
                              n896 = Add(x=w1312, y=4) -> (x+y=w1325:i32)
                              n897 = Increment(x=w1312) -> (x+1=w1328:i32)
                              n898 = Increment(x=w1325) -> (x+1=w1326:i32)
                              n899 = Index Array(array=w1316, index #1=w1328, index #2=w1312, index #3=w1326, index #4=w1325) -> (element #1=w1324:u8, element #2=w1323:u8, element #3=w1322:u8, element #4=w1321:u8)
                              n900 = Join Numbers(hi=w1324, lo=w1323) -> ((hi.lo)=w1314:u16)
                              n901 = Join Numbers(hi=w1322, lo=w1321) -> ((hi.lo)=w1320:u16)
                              n902 = Add(x=w1320, y=u16 32) -> (x+y=w1315:u16)
                              n903 = Greater Or Equal?(x=w1318, y=w1315) -> (x >= y?=w1317:bool)
                              n904 = case shown="True" w1317 {
                                tunnel: w1316 -> [_ w1334]
                                tunnel: w1315 -> [_ w1333]
                                tunnel: w1314 -> [_ w1330]
                                tunnel: [_ w1329] -> w1313
                                frame False {
                                }
                                frame True {
                                n905 = Delete From Array(array=w1334, length=w1333, index=0) -> (deleted portion=w1331:u8[], array with subset deleted=w1329:u8[])
                                n906 = case shown="99" w1330 {
                                tunnel: w1331 -> [_ w1337 w1375]
                                frame 0, Default {
                                }
                                frame 42 {
                                n907 = local read "ecef ref"() -> (w1336:dbl[])
                                n908 = call "novatel_bestpos.vi"("ecef ref"=w1336, "gps_data"=w1337) -> ("LCC"=w1335:dbl[])  [unwired: 9 in]
                                n909 = flat-sequence {
                                tunnel: w1335 -> [w1340]
                                frame #0 {
                                n910 = Index Array(array=w1340, index=1) -> (element=w1343:dbl)
                                n911 = Not Equal To 0?(x=w1343) -> (x != 0?=w1339:bool)
                                n912 = local read "LCM"() -> (w1342:bool)
                                n913 = And(x=w1339, y=w1342) -> (x .and. y?=w1338:bool)
                                n914 = case shown="True" w1338 {
                                tunnel: w1340 -> [_ w1363]
                                frame False {
                                }
                                frame True {
                                n915 = Get Date/Time In Seconds() -> (seconds since 1Jan1904=w1348:timestamp)
                                n916 = To Double Precision Float(number=w1348) -> (double precision float=w1347:dbl)
                                n917 = global read "G_rio.vi" "LCM_GGA_T"() -> (w1372:T12)
                                n918 = Array To Cluster(array=w1363) -> (cluster=w1371:T13)
                                n919 = Unbundle By Name(w1372) -> ("hash"=w1368:i64)
                                n920 = Multiply(x=w1347, y=1000000.0) -> (x*y=w1345:dbl)
                                n921 = Unbundle(w1371) -> ("LCC[0]"=w1373:dbl, "LCC[2]"=w1362:dbl, "LCC[3]"=w1361:dbl, "LCC[4]"=w1360:dbl, "LCC[6]"=w1359:dbl, "LCC[7]"=w1357:dbl, "LCC[8]"=w1355:dbl, "LCC[9]"=w1353:dbl, "LCC[12]"=w1352:dbl, "LCC[13]"=w1351:dbl, "LCC[14]"=w1350:dbl)  [unwired: 4 out]
                                n922 = To Quad Integer(1:w1345) -> (0:w1344:i64)
                                n923 = To Long Integer(number=w1359) -> (32bit integer=w1358:i32)
                                n924 = To Long Integer(number=w1357) -> (32bit integer=w1356:i32)
                                n925 = To Long Integer(number=w1355) -> (32bit integer=w1354:i32)
                                n926 = call "hash.vi"("input"=w1368) -> ("output"=w1367:i64)  [unwired: 10 in]
                                n927 = local read "map"() -> (w1349:i32)
                                n928 = Bundle(cluster=w1372, "hash"=w1367, "sys time"=w1344, "time"=w1373, "x"=w1362, "y"=w1361, "h"=w1360, "numSV"=w1358, "postype"=w1356, "lag"=w1354, "hordev"=w1353, "lat"=w1352, "lon"=w1351, "hgt"=w1350, "map_idx"=w1349) -> (w1369:T12)
                                n929 = Flatten To String(anything=w1369, prepend array or string size? (T)=FALSE) -> (data string=w1365:string)  [unwired: 2 in, 2 out]
                                n930 = global read "G_rio.vi" "LCM"() -> (w1364:T4)
                                n931 = call "LCM_send.vi"("DATA"=w1365, "ID"="GGA_DGPS", "LCM"=w1364) -> ()  [unwired: 7 in, 2 out]
                                }
                                }
                                }
                                }
                                n932 = global write "G_rio.vi" "dgps_pos"(w1335) -> ()
                                }
                                frame 99 {
                                n933 = call "novatel_bestvel.vi"("gps_data"=w1375) -> ("vel"=w1374:dbl[])  [unwired: 10 in]
                                n934 = flat-sequence {
                                tunnel: w1374 -> [w1378]
                                frame #0 {
                                n935 = Index Array(array=w1378, index=1) -> (element=w1380:dbl)
                                n936 = Not Equal To 0?(x=w1380) -> (x != 0?=w1381:bool)
                                n937 = local read "LCM"() -> (w1376:bool)
                                n938 = And(x=w1381, y=w1376) -> (x .and. y?=w1377:bool)
                                n939 = case shown="True" w1377 {
                                tunnel: w1378 -> [_ w1400]
                                frame False {
                                }
                                frame True {
                                n940 = Get Date/Time In Seconds() -> (seconds since 1Jan1904=w1386:timestamp)
                                n941 = To Double Precision Float(number=w1386) -> (double precision float=w1385:dbl)
                                n942 = global read "G_rio.vi" "LCM_RMC_T"() -> (w1401:T14)
                                n943 = Unbundle By Name(w1401) -> ("hash"=w1397:i64)
                                n944 = Multiply(x=w1385, y=1000000.0) -> (x*y=w1383:dbl)
                                n945 = Array To Cluster(array=w1400) -> (cluster=w1399:T15)
                                n946 = To Quad Integer(1:w1383) -> (0:w1382:i64)
                                n947 = call "hash.vi"("input"=w1397) -> ("output"=w1396:i64)  [unwired: 10 in]
                                n948 = Unbundle(w1399) -> ("vel[0]"=w1391:dbl, "vel[2]"=w1390:dbl, "vel[4]"=w1389:dbl, "vel[5]"=w1388:dbl, "vel[6]"=w1387:dbl)  [unwired: 2 out]
                                n949 = Bundle(cluster=w1401, "hash"=w1396, "sys time"=w1382, "time"=w1391, "speed"=w1390, "heading"=w1389, "lat"=w1388, "lon"=w1387) -> (w1392:T14)
                                n950 = Flatten To String(anything=w1392, prepend array or string size? (T)=FALSE) -> (data string=w1394:string)  [unwired: 2 in, 2 out]
                                n951 = global read "G_rio.vi" "LCM"() -> (w1393:T4)
                                n952 = call "LCM_send.vi"("DATA"=w1394, "ID"="RMC_DGPS", "LCM"=w1393) -> ()  [unwired: 7 in, 2 out]
                                }
                                }
                                }
                                }
                                n953 = global write "G_rio.vi" "dgps_vel"(w1374) -> ()
                                }
                                }
                                }
                              }
                            }
                          }
                        }
                        "rest" <- w1288
                      }
                      frame True {
                      }
                    }
                  }
                }
              }
            }
          }
        }
        frame Enabled {
          n954 = while {
            stop <- FALSE stop-if-true
            n955 = flat-sequence {
              tunnel: [w1408] -> w1406
              tunnel: w1406 -> [w1413]
              frame #0 {
                n956 = Wait Until Next ms Multiple(millisecond multiple=u32 50) -> (millisecond timer value=w1411:u32)
                n957 = feedback #21(w1411) -> (w1410:u32)
                n958 = feedback-in #21(w1411) -> ()
                n959 = Subtract(x=w1411, y=w1410) -> (x-y=→"GPS_time 100":u32)
                n960 = local read "ublox"() -> (w1408:bool)
              }
              frame #1 {
                n961 = case shown="False" w1413 {
                  frame False {
                    n962 = First Call?() -> (First Call?: T/F=w1414:bool)
                    n963 = case shown="False" w1414 {
                      frame False {
                        n964 = for {
                          N: 5 -> [_]
                          stop <- w1420 stop-if-true
                          n965 = local read "novatel"() -> (w1416:refnum<visa-resource-name>)
                          n966 = VISA Read(VISA resource name=w1416, byte count=u32 150) -> (read buffer=w1422:string, error out=w1421:errorcluster)  [unwired: 1 in, 2 out]
                          n967 = local read "ecef ref"() -> (w1423:dbl[])
                          n968 = Unbundle By Name(w1421) -> ("code"=w1419:i32, "status"=w1420:bool)
                          n969 = call "nmea.vi"("ecef ref"=w1423, "NMEA"=w1422) -> ("output"=w1425:dbl[], "type"=w1424:u32)  [unwired: 8 in]
                          n970 = case shown="1" w1424 {
                            tunnel: w1425 -> [_ w1434 w1469]
                            frame 0, Default {
                            }
                            frame 1 {
                              n971 = global write "G_rio.vi" "dgps_pos"(w1434) -> ()
                              n972 = Index Array(array=w1434, index=1) -> (element=w1437:dbl)
                              n973 = Not Equal To 0?(x=w1437) -> (x != 0?=w1438:bool)
                              n974 = local read "LCM"() -> (w1436:bool)
                              n975 = And(x=w1438, y=w1436) -> (x .and. y?=w1433:bool)
                              n976 = case shown="True" w1433 {
                                tunnel: w1434 -> [_ w1458]
                                frame False {
                                }
                                frame True {
                                n977 = Get Date/Time In Seconds() -> (seconds since 1Jan1904=w1443:timestamp)
                                n978 = To Double Precision Float(number=w1443) -> (double precision float=w1442:dbl)
                                n979 = global read "G_rio.vi" "LCM_GGA_T"() -> (w1467:T12)
                                n980 = Array To Cluster(array=w1458) -> (cluster=w1466:T16)
                                n981 = Unbundle By Name(w1467) -> ("hash"=w1463:i64)
                                n982 = Multiply(x=w1442, y=1000000.0) -> (x*y=w1440:dbl)
                                n983 = Unbundle(w1466) -> ("output[0]"=w1468:dbl, "output[2]"=w1457:dbl, "output[3]"=w1456:dbl, "output[4]"=w1455:dbl, "output[6]"=w1454:dbl, "output[7]"=w1452:dbl, "output[8]"=w1450:dbl, "output[9]"=w1448:dbl, "output[12]"=w1447:dbl, "output[13]"=w1446:dbl, "output[14]"=w1445:dbl)  [unwired: 4 out]
                                n984 = call "hash.vi"("input"=w1463) -> ("output"=w1462:i64)  [unwired: 10 in]
                                n985 = To Quad Integer(1:w1440) -> (0:w1439:i64)
                                n986 = To Long Integer(number=w1454) -> (32bit integer=w1453:i32)
                                n987 = To Long Integer(number=w1452) -> (32bit integer=w1451:i32)
                                n988 = To Long Integer(number=w1450) -> (32bit integer=w1449:i32)
                                n989 = local read "map"() -> (w1444:i32)
                                n990 = Bundle(cluster=w1467, "hash"=w1462, "sys time"=w1439, "time"=w1468, "x"=w1457, "y"=w1456, "h"=w1455, "numSV"=w1453, "postype"=w1451, "lag"=w1449, "hordev"=w1448, "lat"=w1447, "lon"=w1446, "hgt"=w1445, "map_idx"=w1444) -> (w1464:T12)
                                n991 = Flatten To String(anything=w1464, prepend array or string size? (T)=FALSE) -> (data string=w1460:string)  [unwired: 2 in, 2 out]
                                n992 = global read "G_rio.vi" "LCM"() -> (w1459:T4)
                                n993 = call "LCM_send.vi"("DATA"=w1460, "ID"="GGA_1", "LCM"=w1459) -> ()  [unwired: 7 in, 2 out]
                                }
                              }
                            }
                            frame 2 {
                              n994 = flat-sequence {
                                tunnel: w1469 -> [w1471]
                                frame #0 {
                                n995 = Index Array(array=w1471, index=1) -> (element=w1474:dbl)
                                n996 = Not Equal To 0?(x=w1474) -> (x != 0?=w1475:bool)
                                n997 = local read "LCM"() -> (w1473:bool)
                                n998 = And(x=w1475, y=w1473) -> (x .and. y?=w1470:bool)
                                n999 = case shown="True" w1470 {
                                tunnel: w1471 -> [_ w1494]
                                frame False {
                                }
                                frame True {
                                n1000 = Get Date/Time In Seconds() -> (seconds since 1Jan1904=w1480:timestamp)
                                n1001 = To Double Precision Float(number=w1480) -> (double precision float=w1479:dbl)
                                n1002 = global read "G_rio.vi" "LCM_RMC_T"() -> (w1495:T14)
                                n1003 = Unbundle By Name(w1495) -> ("hash"=w1491:i64)
                                n1004 = Multiply(x=w1479, y=1000000.0) -> (x*y=w1477:dbl)
                                n1005 = Array To Cluster(array=w1494) -> (cluster=w1493:T17)
                                n1006 = To Quad Integer(1:w1477) -> (0:w1476:i64)
                                n1007 = call "hash.vi"("input"=w1491) -> ("output"=w1490:i64)  [unwired: 10 in]
                                n1008 = Unbundle(w1493) -> ("output[0]"=w1485:dbl, "output[2]"=w1484:dbl, "output[4]"=w1483:dbl, "output[5]"=w1482:dbl, "output[6]"=w1481:dbl)  [unwired: 2 out]
                                n1009 = Bundle(cluster=w1495, "hash"=w1490, "sys time"=w1476, "time"=w1485, "speed"=w1484, "heading"=w1483, "lat"=w1482, "lon"=w1481) -> (w1486:T14)
                                n1010 = Flatten To String(anything=w1486, prepend array or string size? (T)=FALSE) -> (data string=w1488:string)  [unwired: 2 in, 2 out]
                                n1011 = global read "G_rio.vi" "LCM"() -> (w1487:T4)
                                n1012 = call "LCM_send.vi"("DATA"=w1488, "ID"="RMC_1", "LCM"=w1487) -> ()  [unwired: 7 in, 2 out]
                                }
                                }
                                }
                              }
                              n1013 = global write "G_rio.vi" "dgps_vel"(w1469) -> ()
                            }
                          }
                          n1014 = case shown="-1073807194" w1419 {
                            tunnel: w1416 -> [_ _ w1429]
                            tunnel: [TRUE _ _] -> w1418
                            frame 0, Default {
                            }
                            frame -1073807343 {
                            }
                            frame -1073807194 {
                              n1015 = VISA Close(VISA resource name=w1429) -> (error out=w1430:errorcluster)  [unwired: 1 in]
                              n1016 = call-poly "VISA Configure Serial Port"("VISA resource name"=refnum<visa-resource-name> "ASRL1::INSTR", "timeout (10sec)"=u32 10, "baud rate (9600)"=u32 115200, "error in (no error)"=w1430) -> ("VISA resource name out"=w1428:refnum<visa-resource-name>)  [unwired: 10 in, 1 out]
                              n1017 = local write "novatel"(w1428) -> ()
                            }
                          }
                          n1018 = global write "G_rio.vi" "A_GPS 2"(w1418) -> ()
                          n1019 = global write "G_rio.vi" "A_GPS"(w1418) -> ()
                        }
                      }
                      frame True {
                        n1020 = global write "G_rio.vi" "R"(T11 [[5.0, 0.0, 0.0], [0.0, 5.0, 0.0], [0.0, 0.0, 0.5]] ("R")) -> ()
                      }
                    }
                  }
                  frame True {
                    n1021 = First Call?() -> (First Call?: T/F=w1497:bool)
                    n1022 = case shown="False" w1497 {
                      frame False {
                        n1023 = for {
                          N: 5 -> [_]
                          stop <- w1583 stop-if-true
                          n1024 = local read "gps2"() -> (w1584:refnum<visa-resource-name>)
                          n1025 = VISA Read(VISA resource name=w1584, byte count=u32 100) -> (VISA resource name out=w1581:refnum<visa-resource-name>, read buffer=w1590:string, error out=w1585:errorcluster)  [unwired: 1 in, 1 out]
                          n1026 = local read "ecef ref"() -> (w1589:dbl[])
                          n1027 = Unbundle By Name(w1585) -> ("code"=w1582:i32, "status"=w1583:bool)
                          n1028 = call "nmea.vi"("ecef ref"=w1589, "NMEA"=w1590) -> ("output"=w1587:dbl[], "type"=w1588:u32)  [unwired: 8 in]
                          n1029 = case shown="1" w1588 {
                            tunnel: w1587 -> [_ w1601 w1641]
                            frame 0, Default {
                            }
                            frame 1 {
                              n1030 = global write "G_rio.vi" "gps_pos 2"(w1601) -> ()
                              n1031 = Index Array(array=w1601, index=1) -> (element=w1602:dbl)
                              n1032 = Not Equal To 0?(x=w1602) -> (x != 0?=w1600:bool)
                              n1033 = local read "LCM"() -> (w1603:bool)
                              n1034 = And(x=w1600, y=w1603) -> (x .and. y?=w1605:bool)
                              n1035 = case shown="True" w1605 {
                                tunnel: w1601 -> [_ w1625]
                                frame False {
                                }
                                frame True {
                                n1036 = Get Date/Time In Seconds() -> (seconds since 1Jan1904=w1610:timestamp)
                                n1037 = To Double Precision Float(number=w1610) -> (double precision float=w1609:dbl)
                                n1038 = global read "G_rio.vi" "LCM_GGA_T"() -> (w1634:T12)
                                n1039 = Array To Cluster(array=w1625) -> (cluster=w1633:T16)
                                n1040 = Unbundle By Name(w1634) -> ("hash"=w1630:i64)
                                n1041 = Multiply(x=w1609, y=1000000.0) -> (x*y=w1607:dbl)
                                n1042 = Unbundle(w1633) -> ("output[0]"=w1635:dbl, "output[2]"=w1624:dbl, "output[3]"=w1623:dbl, "output[4]"=w1622:dbl, "output[6]"=w1621:dbl, "output[7]"=w1619:dbl, "output[8]"=w1617:dbl, "output[9]"=w1615:dbl, "output[12]"=w1614:dbl, "output[13]"=w1613:dbl, "output[14]"=w1612:dbl)  [unwired: 4 out]
                                n1043 = call "hash.vi"("input"=w1630) -> ("output"=w1629:i64)  [unwired: 10 in]
                                n1044 = To Quad Integer(1:w1607) -> (0:w1606:i64)
                                n1045 = To Long Integer(number=w1621) -> (32bit integer=w1620:i32)
                                n1046 = To Long Integer(number=w1619) -> (32bit integer=w1618:i32)
                                n1047 = To Long Integer(number=w1617) -> (32bit integer=w1616:i32)
                                n1048 = local read "map"() -> (w1611:i32)
                                n1049 = Bundle(cluster=w1634, "hash"=w1629, "sys time"=w1606, "time"=w1635, "x"=w1624, "y"=w1623, "h"=w1622, "numSV"=w1620, "postype"=w1618, "lag"=w1616, "hordev"=w1615, "lat"=w1614, "lon"=w1613, "hgt"=w1612, "map_idx"=w1611) -> (w1631:T12)
                                n1050 = Flatten To String(anything=w1631, prepend array or string size? (T)=FALSE) -> (data string=w1627:string)  [unwired: 2 in, 2 out]
                                n1051 = global read "G_rio.vi" "LCM"() -> (w1626:T4)
                                n1052 = call "LCM_send.vi"("DATA"=w1627, "ID"="GGA_2", "LCM"=w1626) -> ()  [unwired: 7 in, 2 out]
                                }
                              }
                            }
                            frame 2 {
                              n1053 = global write "G_rio.vi" "gps_vel 2"(w1641) -> ()
                              n1054 = Index Array(array=w1641, index=1) -> (element=w1638:dbl)
                              n1055 = Not Equal To 0?(x=w1638) -> (x != 0?=w1637:bool)
                              n1056 = local read "LCM"() -> (w1639:bool)
                              n1057 = And(x=w1637, y=w1639) -> (x .and. y?=w1636:bool)
                              n1058 = case shown="True" w1636 {
                                tunnel: w1641 -> [_ w1652]
                                frame False {
                                }
                                frame True {
                                n1059 = Get Date/Time In Seconds() -> (seconds since 1Jan1904=w1646:timestamp)
                                n1060 = To Double Precision Float(number=w1646) -> (double precision float=w1645:dbl)
                                n1061 = global read "G_rio.vi" "LCM_RMC_T"() -> (w1653:T14)
                                n1062 = Unbundle By Name(w1653) -> ("hash"=w1657:i64)
                                n1063 = Multiply(x=w1645, y=1000000.0) -> (x*y=w1643:dbl)
                                n1064 = Array To Cluster(array=w1652) -> (cluster=w1654:T17)
                                n1065 = call "hash.vi"("input"=w1657) -> ("output"=w1658:i64)  [unwired: 10 in]
                                n1066 = To Quad Integer(1:w1643) -> (0:w1642:i64)
                                n1067 = Unbundle(w1654) -> ("output[0]"=w1651:dbl, "output[2]"=w1650:dbl, "output[4]"=w1649:dbl, "output[5]"=w1648:dbl, "output[6]"=w1647:dbl)  [unwired: 2 out]
                                n1068 = Bundle(cluster=w1653, "hash"=w1658, "sys time"=w1642, "time"=w1651, "speed"=w1650, "heading"=w1649, "lat"=w1648, "lon"=w1647) -> (w1656:T14)
                                n1069 = Flatten To String(anything=w1656, prepend array or string size? (T)=FALSE) -> (data string=w1660:string)  [unwired: 2 in, 2 out]
                                n1070 = global read "G_rio.vi" "LCM"() -> (w1661:T4)
                                n1071 = call "LCM_send.vi"("DATA"=w1660, "ID"="RMC_2", "LCM"=w1661) -> ()  [unwired: 7 in, 2 out]
                                }
                              }
                            }
                          }
                          n1072 = case shown="0, Default" w1582 {
                            tunnel: w1581 -> [_ _ w1595]
                            tunnel: [TRUE FALSE FALSE] -> w1580
                            frame 0, Default {
                            }
                            frame -1073807343 {
                            }
                            frame -1073807194 {
                              n1073 = VISA Close(VISA resource name=w1595) -> (error out=w1596:errorcluster)  [unwired: 1 in]
                              n1074 = call-poly "VISA Configure Serial Port"("VISA resource name"=refnum<visa-resource-name> "USB0::0x1546::0x01A6::NI-VISA-0::1::RAW", "timeout (10sec)"=u32 1, "baud rate (9600)"=u32 115200, "error in (no error)"=w1596) -> ("VISA resource name out"=w1594:refnum<visa-resource-name>)  [unwired: 10 in, 1 out]
                              n1075 = local write "gps2"(w1594) -> ()
                            }
                          }
                          n1076 = global write "G_rio.vi" "A_GPS 2"(w1580) -> ()
                        }
                        n1077 = for {
                          N: 5 -> [_]
                          stop <- w1503 stop-if-true
                          n1078 = local read "gps1"() -> (w1502:refnum<visa-resource-name>)
                          n1079 = VISA Read(VISA resource name=w1502, byte count=u32 100) -> (read buffer=w1506:string, error out=w1504:errorcluster)  [unwired: 1 in, 2 out]
                          n1080 = local read "ecef ref"() -> (w1507:dbl[])
                          n1081 = Unbundle By Name(w1504) -> ("code"=w1501:i32, "status"=w1503:bool)
                          n1082 = call "nmea.vi"("ecef ref"=w1507, "NMEA"=w1506) -> ("output"=w1509:dbl[], "type"=w1508:u32)  [unwired: 8 in]
                          n1083 = case shown="0, Default" w1508 {
                            tunnel: w1509 -> [_ w1518 w1553]
                            frame 0, Default {
                            }
                            frame 1 {
                              n1084 = global write "G_rio.vi" "gps_pos 1"(w1518) -> ()
                              n1085 = Index Array(array=w1518, index=1) -> (element=w1521:dbl)
                              n1086 = Not Equal To 0?(x=w1521) -> (x != 0?=w1522:bool)
                              n1087 = local read "LCM"() -> (w1520:bool)
                              n1088 = And(x=w1522, y=w1520) -> (x .and. y?=w1517:bool)
                              n1089 = case shown="True" w1517 {
                                tunnel: w1518 -> [_ w1542]
                                frame False {
                                }
                                frame True {
                                n1090 = Get Date/Time In Seconds() -> (seconds since 1Jan1904=w1527:timestamp)
                                n1091 = To Double Precision Float(number=w1527) -> (double precision float=w1526:dbl)
                                n1092 = global read "G_rio.vi" "LCM_GGA_T"() -> (w1551:T12)
                                n1093 = Array To Cluster(array=w1542) -> (cluster=w1550:T16)
                                n1094 = Unbundle By Name(w1551) -> ("hash"=w1547:i64)
                                n1095 = Multiply(x=w1526, y=1000000.0) -> (x*y=w1524:dbl)
                                n1096 = Unbundle(w1550) -> ("output[0]"=w1552:dbl, "output[2]"=w1541:dbl, "output[3]"=w1540:dbl, "output[4]"=w1539:dbl, "output[6]"=w1538:dbl, "output[7]"=w1536:dbl, "output[8]"=w1534:dbl, "output[9]"=w1532:dbl, "output[12]"=w1531:dbl, "output[13]"=w1530:dbl, "output[14]"=w1529:dbl)  [unwired: 4 out]
                                n1097 = call "hash.vi"("input"=w1547) -> ("output"=w1546:i64)  [unwired: 10 in]
                                n1098 = To Quad Integer(1:w1524) -> (0:w1523:i64)
                                n1099 = To Long Integer(number=w1538) -> (32bit integer=w1537:i32)
                                n1100 = To Long Integer(number=w1536) -> (32bit integer=w1535:i32)
                                n1101 = To Long Integer(number=w1534) -> (32bit integer=w1533:i32)
                                n1102 = local read "map"() -> (w1528:i32)
                                n1103 = Bundle(cluster=w1551, "hash"=w1546, "sys time"=w1523, "time"=w1552, "x"=w1541, "y"=w1540, "h"=w1539, "numSV"=w1537, "postype"=w1535, "lag"=w1533, "hordev"=w1532, "lat"=w1531, "lon"=w1530, "hgt"=w1529, "map_idx"=w1528) -> (w1548:T12)
                                n1104 = Flatten To String(anything=w1548, prepend array or string size? (T)=FALSE) -> (data string=w1544:string)  [unwired: 2 in, 2 out]
                                n1105 = global read "G_rio.vi" "LCM"() -> (w1543:T4)
                                n1106 = call "LCM_send.vi"("DATA"=w1544, "ID"="GGA_1", "LCM"=w1543) -> ()  [unwired: 7 in, 2 out]
                                }
                              }
                            }
                            frame 2 {
                              n1107 = flat-sequence {
                                tunnel: w1553 -> [w1555]
                                frame #0 {
                                n1108 = Index Array(array=w1555, index=1) -> (element=w1558:dbl)
                                n1109 = Not Equal To 0?(x=w1558) -> (x != 0?=w1559:bool)
                                n1110 = local read "LCM"() -> (w1557:bool)
                                n1111 = And(x=w1559, y=w1557) -> (x .and. y?=w1554:bool)
                                n1112 = case shown="True" w1554 {
                                tunnel: w1555 -> [_ w1578]
                                frame False {
                                }
                                frame True {
                                n1113 = Get Date/Time In Seconds() -> (seconds since 1Jan1904=w1564:timestamp)
                                n1114 = To Double Precision Float(number=w1564) -> (double precision float=w1563:dbl)
                                n1115 = global read "G_rio.vi" "LCM_RMC_T"() -> (w1579:T14)
                                n1116 = Unbundle By Name(w1579) -> ("hash"=w1575:i64)
                                n1117 = Multiply(x=w1563, y=1000000.0) -> (x*y=w1561:dbl)
                                n1118 = Array To Cluster(array=w1578) -> (cluster=w1577:T17)
                                n1119 = call "hash.vi"("input"=w1575) -> ("output"=w1574:i64)  [unwired: 10 in]
                                n1120 = To Quad Integer(1:w1561) -> (0:w1560:i64)
                                n1121 = Unbundle(w1577) -> ("output[0]"=w1569:dbl, "output[2]"=w1568:dbl, "output[4]"=w1567:dbl, "output[5]"=w1566:dbl, "output[6]"=w1565:dbl)  [unwired: 2 out]
                                n1122 = Bundle(cluster=w1579, "hash"=w1574, "sys time"=w1560, "time"=w1569, "speed"=w1568, "heading"=w1567, "lat"=w1566, "lon"=w1565) -> (w1570:T14)
                                n1123 = Flatten To String(anything=w1570, prepend array or string size? (T)=FALSE) -> (data string=w1572:string)  [unwired: 2 in, 2 out]
                                n1124 = global read "G_rio.vi" "LCM"() -> (w1571:T4)
                                n1125 = call "LCM_send.vi"("DATA"=w1572, "ID"="RMC_1", "LCM"=w1571) -> ()  [unwired: 7 in, 2 out]
                                }
                                }
                                }
                              }
                              n1126 = global write "G_rio.vi" "gps_vel 1"(w1553) -> ()
                            }
                          }
                          n1127 = case shown="-1073807343" w1501 {
                            tunnel: w1502 -> [_ _ w1512]
                            tunnel: [TRUE _ _] -> w1500
                            frame 0, Default {
                            }
                            frame -1073807343 {
                            }
                            frame -1073807194 {
                              n1128 = VISA Close(VISA resource name=w1512) -> (error out=w1513:errorcluster)  [unwired: 1 in]
                              n1129 = call-poly "VISA Configure Serial Port"("VISA resource name"=refnum<visa-resource-name> "USB0::0x1546::0x01A6::NI-VISA-1::1::RAW", "timeout (10sec)"=u32 1, "baud rate (9600)"=u32 115200, "error in (no error)"=w1513) -> ("VISA resource name out"=w1511:refnum<visa-resource-name>)  [unwired: 10 in, 1 out]
                              n1130 = local write "gps1"(w1511) -> ()
                            }
                          }
                          n1131 = global write "G_rio.vi" "A_GPS"(w1500) -> ()
                        }
                      }
                      frame True {
                        n1132 = global write "G_rio.vi" "R"(T11 [[10.0, 0.0, 0.0], [0.0, 10.0, 0.0], [0.0, 0.0, 0.5]] ("R")) -> ()
                      }
                    }
                  }
                }
              }
            }
          }
        }
      }
      n1133 = while {
        shift-right: [w1668] -> _
        shift-left: w1134 -> [w1667]
        stop <- FALSE stop-if-true
        n1134 = flat-sequence {
          tunnel: [w1677] -> w1664
          tunnel: w1667 -> [w1677]
          tunnel: w1664 -> [w1683]
          tunnel: [w1684] -> w1665
          tunnel: [w1682] -> w1663
          tunnel: [w2383] -> w1668
          tunnel: w1665 -> [w2384]
          tunnel: w1663 -> [w2383]
          frame #0 {
            n1135 = global read "G_rio.vi" "time"() -> (w1670:u32)
            n1136 = Wait Until Next ms Multiple(millisecond multiple=u32 10) -> (millisecond timer value=w1675:u32)
            n1137 = feedback #22(w1670) -> (w1669:u32)
            n1138 = feedback-in #22(w1670) -> ()
            n1139 = Subtract(x=w1670, y=w1669) -> (x-y=w1671:u32)
            n1140 = flat-sequence {
              tunnel: w1675 -> [w1680]
              frame #0 {
                n1141 = feedback #23(w1680) -> (w1681:u32)
                n1142 = feedback-in #23(w1680) -> ()
                n1143 = Subtract(x=w1680, y=w1681) -> (x-y=w1679:u32)
                n1144 = To Long Integer(number=w1679) -> (32bit integer=→"Pos_time 10":i32)
              }
            }
            n1145 = To Double Precision Float(number=w1671) -> (double precision float=w1672:dbl)
            n1146 = Multiply(x=w1672, y=1e-07) -> (x*y=→"dt":dbl)
          }
          frame #1 {
            n1147 = disable-structure shown="Enabled" {
              disable-tunnel: [w1685 w2090] -> w1684
              disable-tunnel: w1683 -> [w1686 w2112]
              disable-tunnel: [w1685 w2099] -> w1682
              frame Enabled {
                n1148 = flat-sequence {
                  tunnel: w1686 -> [w1699]
                  tunnel: [w1699] -> w1687
                  tunnel: [w1821] -> w1685
                  tunnel: w1687 -> [w1822]
                  frame #0 {
                    n1149 = case shown="True" "ublox" {
                      tunnel: [w1793 w1811] -> w1688
                      tunnel: [w1792 w1812] -> w1690
                      frame True {
                        n1150 = global read "G_rio.vi" "gps_pos 1"() -> (w1808:dbl[])
                        n1151 = global read "G_rio.vi" "gps_pos 2"() -> (w1795:dbl[])
                        n1152 = Add(x=w1808, y=w1795) -> (x+y=w1810:dbl[])
                        n1153 = Index Array(array=w1808, index #1=0 ("index")) -> (element #1=w1807:dbl, element #2=w1806:dbl)  [unwired: 1 in]
                        n1154 = Index Array(array=w1795, index #1=0 ("index")) -> (element #1=w1796:dbl, element #2=w1797:dbl)  [unwired: 1 in]
                        n1155 = feedback #24(w1807) -> (w1805:dbl)
                        n1156 = feedback-in #24(w1807) -> ()
                        n1157 = feedback #25(w1796) -> (w1798:dbl)
                        n1158 = feedback-in #25(w1796) -> ()
                        n1159 = Not Equal?(x=w1807, y=w1805) -> (x != y?=w1804:bool)
                        n1160 = Not Equal?(x=w1796, y=w1798) -> (x != y?=w1799:bool)
                        n1161 = Not Equal To 0?(x=w1806) -> (x != 0?=w1803:bool)
                        n1162 = Not Equal To 0?(x=w1797) -> (x != 0?=w1800:bool)
                        n1163 = And(x=w1804, y=w1803) -> (x .and. y?=w1791:bool)
                        n1164 = And(x=w1799, y=w1800) -> (x .and. y?=w1794:bool)
                        n1165 = And(x=w1791, y=w1794) -> (x .and. y?=w1793:bool)
                        n1166 = Multiply(x=w1810, y=0.5) -> (x*y=w1792:dbl[])
                      }
                      frame False {
                        n1167 = global read "G_rio.vi" "dgps_pos"() -> (w1812:dbl[])
                        n1168 = Index Array(array=w1812, index #1=0 ("index")) -> (element #1=w1818:dbl, element #2=w1817:dbl)  [unwired: 1 in]
                        n1169 = feedback #26(w1818) -> (w1816:dbl)
                        n1170 = feedback-in #26(w1818) -> ()
                        n1171 = Not Equal?(x=w1818, y=w1816) -> (x != y?=w1815:bool)
                        n1172 = Not Equal To 0?(x=w1817) -> (x != 0?=w1814:bool)
                        n1173 = And(x=w1815, y=w1814) -> (x .and. y?=w1811:bool)
                      }
                    }
                    n1174 = case shown="False" "ublox" {
                      tunnel: [w1700 w1757] -> w1689
                      tunnel: [w1718 w1758] -> w1693
                      frame True {
                        n1175 = global read "G_rio.vi" "gps_vel 1"() -> (w1745:dbl[])
                        n1176 = global read "G_rio.vi" "gps_vel 2"() -> (w1724:dbl[])
                        n1177 = Index Array(array=w1745, index #1=0 ("index"), index #2=1 ("index"), index #3=4 ("index"), index #4=2 ("index")) -> (element #1=w1736:dbl, element #2=w1741:dbl, element #3=w1738:dbl, element #4=w1708:dbl)
                        n1178 = Index Array(array=w1724, index #1=0 ("index"), index #2=1 ("index"), index #3=4 ("index"), index #4=2 ("index")) -> (element #1=w1733:dbl, element #2=w1728:dbl, element #3=w1731:dbl, element #4=w1707:dbl)
                        n1179 = global read "G_rio.vi" "VS_CAN"() -> (w1703:dbl)
                        n1180 = Add(x=w1708, y=w1707) -> (x+y=w1706:dbl)
                        n1181 = Not Equal To 0?(x=w1728) -> (x != 0?=w1729:bool)
                        n1182 = call "angleconv.vi"("deg"=w1738) -> ("rad"=w1721:dbl)  [unwired: 9 in, 1 out]
                        n1183 = call "angleconv.vi"("deg"=w1731) -> ("rad"=w1720:dbl)  [unwired: 9 in, 1 out]
                        n1184 = feedback #27(0.0 ("Real Matrix Element")) -> (w1735:dbl)
                        n1185 = feedback-in #27(w1736) -> ()
                        n1186 = feedback #28(0.0 ("Real Matrix Element")) -> (w1734:dbl)
                        n1187 = feedback-in #28(w1733) -> ()
                        n1188 = Not Equal?(x=w1736, y=w1735) -> (x != y?=w1742:bool)
                        n1189 = Not Equal?(x=w1733, y=w1734) -> (x != y?=w1727:bool)
                        n1190 = call "headingweightsum.vi"("a"=0.5, "h1"=w1720, "h2"=w1721) -> ("a*h2+(1-a)*h1"=w1718:dbl)  [unwired: 8 in]
                        n1191 = Absolute Value(x=w1703) -> (abs(x)=w1715:dbl)
                        n1192 = Not Equal To 0?(x=w1741) -> (x != 0?=w1740:bool)
                        n1193 = Multiply(x=w1706, y=0.5) -> (x*y=w1716:dbl)
                        n1194 = And(x=w1742, y=w1740) -> (x .and. y?=w1723:bool)
                        n1195 = And(x=w1727, y=w1729) -> (x .and. y?=w1722:bool)
                        n1196 = Divide(x=w1716, y=w1715) -> (x/y=w1717:dbl)
                        n1197 = And(x=w1723, y=w1722) -> (x .and. y?=w1700:bool)
                        n1198 = Decrement(x=w1717) -> (x-1=w1712:dbl)
                        n1199 = Absolute Value(x=w1712) -> (abs(x)=w1713:dbl)
                        n1200 = Greater?(x=w1703, y=15.0) -> (0:w1701:bool)
                        n1201 = Less?(x=w1713, y=0.05) -> (x < y?=w1705:bool)
                        n1202 = Compound Arithmetic op=AND(w1701, w1705, w1700) -> (w1704:bool)
                        n1203 = case shown="True" w1704 {
                          tunnel: w1717 -> [_ w1753]
                          frame False {
                          }
                          frame True {
                            w1747 = u64 18446744073709551615
                            n1204 = local read "vcount"() -> (w1750:u64)
                            n1205 = local read "vgain"() -> (w1755:dbl)
                            n1206 = Increment(x=w1750) -> (x+1=w1749:u64)
                            n1207 = Multiply(x=w1755, y=w1750) -> (x*y=w1754:dbl)
                            n1208 = Not Equal?(x=w1750, y=w1747) -> (x != y?=w1748:bool)
                            n1209 = Add(x=w1753, y=w1754) -> (x+y=w1752:dbl)
                            n1210 = Select(t=w1749, s=w1748, f=w1747) -> (s? t:f=w1746:u64)
                            n1211 = local write "vcount"(w1746) -> ()
                            n1212 = Divide(x=w1752, y=w1746) -> (x/y=w1751:dbl)
                            n1213 = local write "vgain"(w1751) -> ()
                          }
                        }
                      }
                      frame False {
                        n1214 = global read "G_rio.vi" "dgps_vel"() -> (w1780:dbl[])
                        n1215 = global read "G_rio.vi" "VS_CAN"() -> (w1761:dbl)
                        n1216 = Index Array(array=w1780, index #1=0 ("index"), index #2=1 ("index"), index #3=4 ("index"), index #4=2 ("index")) -> (element #1=w1771:dbl, element #2=w1776:dbl, element #3=w1773:dbl, element #4=w1756:dbl)
                        n1217 = Absolute Value(x=w1761) -> (abs(x)=w1768:dbl)
                        n1218 = Divide(x=w1756, y=w1768) -> (x/y=w1769:dbl)
                        n1219 = feedback #29(0.0 ("Real Matrix Element")) -> (w1770:dbl)
                        n1220 = feedback-in #29(w1771) -> ()
                        n1221 = Not Equal?(x=w1771, y=w1770) -> (x != y?=w1777:bool)
                        n1222 = Decrement(x=w1769) -> (x-1=w1765:dbl)
                        n1223 = Not Equal To 0?(x=w1776) -> (x != 0?=w1775:bool)
                        n1224 = And(x=w1777, y=w1775) -> (x .and. y?=w1757:bool)
                        n1225 = Absolute Value(x=w1765) -> (abs(x)=w1766:dbl)
                        n1226 = Greater?(x=w1761, y=15.0) -> (0:w1759:bool)
                        n1227 = Less?(x=w1766, y=0.05) -> (x < y?=w1763:bool)
                        n1228 = Compound Arithmetic op=AND(w1759, w1763, w1757) -> (w1762:bool)
                        n1229 = case shown="True" w1762 {
                          tunnel: w1769 -> [_ w1788]
                          frame False {
                          }
                          frame True {
                            w1782 = u64 18446744073709551615
                            n1230 = local read "vcount"() -> (w1785:u64)
                            n1231 = local read "vgain"() -> (w1790:dbl)
                            n1232 = Increment(x=w1785) -> (x+1=w1784:u64)
                            n1233 = Multiply(x=w1790, y=w1785) -> (x*y=w1789:dbl)
                            n1234 = Not Equal?(x=w1785, y=w1782) -> (x != y?=w1783:bool)
                            n1235 = Add(x=w1788, y=w1789) -> (x+y=w1787:dbl)
                            n1236 = Select(t=w1784, s=w1783, f=w1782) -> (s? t:f=w1781:u64)
                            n1237 = local write "vcount"(w1781) -> ()
                            n1238 = Divide(x=w1787, y=w1781) -> (x/y=w1786:dbl)
                            n1239 = local write "vgain"(w1786) -> ()
                          }
                        }
                        n1240 = call "angleconv.vi"("deg"=w1773) -> ("rad"=w1758:dbl)  [unwired: 9 in, 1 out]
                      }
                    }
                    n1241 = local write "pos_gps"(w1690) -> ()
                    n1242 = local write "get position"(w1688) -> ()
                    n1243 = global read "G_rio.vi" "VS_CAN"() -> (w1694:dbl)
                    n1244 = Greater Or Equal To 0?(x=w1694) -> (x >= 0?=w1695:bool)
                    n1245 = Select(t=0.0, s=w1695, f=3.141592653589793) -> (s? t:f=w1692:dbl)
                    n1246 = local write "get heading"(w1689) -> ()
                    n1247 = call "headingoperater.vi"("h1"=w1692, "h2"=w1693) -> ("h2-h1"=w1691:dbl)  [unwired: 8 in, 1 out]
                    n1248 = local write "h_gps"(w1691) -> ()
                  }
                  frame #1 {
                    n1249 = local read "dt"() -> (w1820:dbl)
                    n1250 = Greater Than 0?(x=w1820) -> (x > 0?=w1819:bool)
                    n1251 = case shown="True" w1819 {
                      tunnel: w1822 -> [w1823 w1826]
                      tunnel: [w1823 w1825] -> w1821
                      frame False {
                      }
                      frame True {
                        n1252 = flat-sequence {
                          tunnel: w1826 -> [w1860]
                          tunnel: [w1838] -> w1824
                          tunnel: [w1889] -> w1825
                          tunnel: w1824 -> [w1888]
                          frame #0 {
                            n1253 = global read "G_rio.vi" "VS_CAN"() -> (w1828:dbl)
                            n1254 = Equal To 0?(x=w1828) -> (x = 0?=w1829:bool)
                            n1255 = case shown="True" w1829 {
                              tunnel: [w1861 _] -> w1827
                              frame False {
                                n1256 = global read "G_rio.vi" "yaw_rate"() -> (w1864:dbl)
                                n1257 = local read "hbias"() -> (w1865:dbl)
                                n1258 = Subtract(x=w1864, y=w1865) -> (x-y=w1862:dbl)
                                n1259 = Negate(x=w1862) -> (-x=w1863:dbl)
                                n1260 = call "angleconv.vi"("deg"=w1863) -> ("rad"=w1861:dbl)  [unwired: 9 in, 1 out]
                              }
                              frame True {
                                n1261 = disable-structure shown="Enabled" {
                                disable-tunnel: [w1868 _] -> w1866
                                frame Enabled {
                                w1870 = u64 18446744073709551615
                                n1262 = local read "hcount"() -> (w1873:u64)
                                n1263 = local read "hbias"() -> (w1876:dbl)
                                n1264 = Not Equal?(x=w1873, y=w1870) -> (x != y?=w1871:bool)
                                n1265 = Increment(x=w1873) -> (x+1=w1872:u64)
                                n1266 = global read "G_rio.vi" "yaw_rate"() -> (w1867:dbl)
                                n1267 = Multiply(x=w1876, y=w1873) -> (x*y=w1875:dbl)
                                n1268 = Select(t=w1872, s=w1871, f=w1870) -> (s? t:f=w1869:u64)
                                n1269 = local write "hcount"(w1869) -> ()
                                n1270 = Add(x=w1867, y=w1875) -> (x+y=w1874:dbl)
                                n1271 = Divide(x=w1874, y=w1869) -> (x/y=w1868:dbl)
                                }
                                frame Disabled {
                                }
                                }
                                n1272 = local write "hbias"(w1866) -> ()
                              }
                            }
                            n1273 = global read "G_rio.vi" "VS_CAN"() -> (w1832:dbl)
                            n1274 = local read "vgain"() -> (w1833:dbl)
                            n1275 = Multiply(x=w1832, y=w1833) -> (x*y=w1831:dbl)
                            n1276 = Divide(x=w1831, y=3.6) -> (x/y=w1830:dbl)
                            n1277 = Index Array(array=w1860, index #1=0 ("index"), index #2=3 ("index"), index #3=1 ("index"), index #4=3 ("index")) -> (element #1=w1854:dbl, element #2=w1852:dbl, element #3=w1848:dbl, element #4=w1843:dbl)
                            n1278 = local read "dt"() -> (w1857:dbl)
                            n1279 = local read "dt"() -> (w1841:dbl)
                            n1280 = Multiply(x=w1830, y=w1857) -> (x*y=w1853:dbl)
                            n1281 = Multiply(x=w1841, y=w1827) -> (x*y=w1834:dbl)
                            n1282 = Cosine(x=w1852) -> (cos(x)=w1858:dbl)
                            n1283 = Sine(x=w1852) -> (sin(x)=w1851:dbl)
                            n1284 = local write "rt"(w1834) -> ()
                            n1285 = Multiply(x=w1858, y=w1853) -> (x*y=w1855:dbl)
                            n1286 = Multiply(x=w1853, y=w1851) -> (x*y=w1850:dbl)
                            n1287 = Add(x=w1854, y=w1855) -> (x+y=w1847:dbl)
                            n1288 = Add(x=w1850, y=w1848) -> (x+y=w1846:dbl)
                            n1289 = call "headingoperater.vi"("h1"=w1834, "h2"=w1843) -> ("h2+h1"=w1842:dbl)  [unwired: 8 in, 1 out]
                            n1290 = Build Array(w1847, w1846, w1830, w1842, w1827) -> (w1838:dbl[])
                            n1291 = Index Array(array=w1838, index=3) -> (element=w1837:dbl)
                            n1292 = local read "h_gps"() -> (w1836:dbl)
                            n1293 = call "headingoperater.vi"("h1"=w1837, "h2"=w1836) -> ("h2-h1"=w1840:dbl)  [unwired: 8 in, 1 out]
                            n1294 = Absolute Value(x=w1840) -> (abs(x)=w1835:dbl)
                            n1295 = local write "heading error"(w1835) -> ()
                          }
                          frame #1 {
                            n1296 = local read "get heading"() -> (w1896:bool)
                            n1297 = local read "get position"() -> (w1895:bool)
                            n1298 = local read "POS init"() -> (w1881:bool)
                            n1299 = case shown="True" w1881 {
                              tunnel: w1896 -> [w1899 w1906]
                              tunnel: w1895 -> [w1903 w1905]
                              tunnel: [w1897 w1904] -> w1891
                              frame False {
                                n1300 = local read "heading error"() -> (w1900:dbl)
                                n1301 = Less?(x=w1900, y=0.05) -> (x < y?=w1901:bool)
                                n1302 = And(x=w1899, y=w1901) -> (x .and. y?=w1898:bool)
                                n1303 = Or(x=w1898, y=w1903) -> (x .or. y?=w1897:bool)
                              }
                              frame True {
                                n1304 = disable-structure shown="Enabled" {
                                disable-tunnel: w1906 -> [w1909 w1911]
                                disable-tunnel: w1905 -> [w1908 w1910]
                                disable-tunnel: [w1907 w1912] -> w1904
                                frame Disabled {
                                n1305 = And(x=w1909, y=w1908) -> (x .and. y?=w1907:bool)
                                }
                                frame Enabled {
                                n1306 = Or(x=w1911, y=w1910) -> (x .or. y?=w1912:bool)
                                }
                                }
                              }
                            }
                            n1307 = global read "G_rio.vi" "VS_CAN"() -> (w1894:dbl)
                            n1308 = local read "heading error"() -> (w1884:dbl)
                            n1309 = Absolute Value(x=w1894) -> (abs(x)=w1893:dbl)
                            n1310 = local read "POS init"() -> (w1882:bool)
                            n1311 = Greater?(x=w1893, y=5.0) -> (0:w1890:bool)
                            n1312 = Less?(x=w1884, y=1.0) -> (x < y?=w1883:bool)
                            n1313 = Or(x=w1883, y=w1882) -> (x .or. y?=w1885:bool)
                            n1314 = And(x=w1891, y=w1890) -> (x .and. y?=w1886:bool)
                            n1315 = And(x=w1886, y=w1885) -> (x .and. y?=w1879:bool)
                            n1316 = Select(t=FALSE, s="GPS init", f=w1879) -> (s? t:f=w1878:bool)
                            n1317 = case shown="True" w1878 {
                              tunnel: [w1916 w1945] -> w1889
                              tunnel: w1888 -> [w1917 w1948]
                              frame False {
                                n1318 = global read "G_rio.vi" "VS_CAN"() -> (w1920:dbl)
                                n1319 = local read "POS init"() -> (w1919:bool)
                                n1320 = Equal To 0?(x=w1920) -> (x = 0?=w1918:bool)
                                n1321 = local read "GPS init"() -> (w1913:bool)
                                n1322 = And(x=w1919, y=w1918) -> (x .and. y?=w1915:bool)
                                n1323 = Or(x=w1915, y=w1913) -> (x .or. y?=w1914:bool)
                                n1324 = case shown="True" w1914 {
                                tunnel: w1917 -> [w1921 w1922]
                                tunnel: [w1921 w1924] -> w1916
                                tunnel: w1913 -> [_ w1923]
                                frame False {
                                }
                                frame True {
                                n1325 = case shown="True" w1923 {
                                tunnel: [w1935 w1944] -> w1924
                                tunnel: w1922 -> [w1930 w1938]
                                frame True {
                                n1326 = Index Array(array=w1930, index #1=2 ("index")) -> (element #2=w1925:dbl, element #3=w1928:dbl)  [unwired: 2 in, 1 out]
                                n1327 = local read "pos_gps"() -> (w1931:dbl[])
                                n1328 = local write "GPS init"(FALSE ("GPS init")) -> ()
                                n1329 = Index Array(array=w1931, index #1=2 ("index")) -> (element #1=w1933:dbl, element #2=w1932:dbl)  [unwired: 1 in]
                                n1330 = local read "h_gps"() -> (w1926:dbl)
                                n1331 = Build Array(w1933, w1932, w1925, w1926, w1928) -> (w1935:dbl[])
                                }
                                frame False {
                                w1937 = 0.0 ("element")
                                n1332 = Index Array(array=w1938, index=3) -> (element=w1936:dbl)
                                n1333 = local read "pos_gps"() -> (w1940:dbl[])
                                n1334 = Index Array(array=w1940, index #1=2 ("index")) -> (element #1=w1942:dbl, element #2=w1941:dbl)  [unwired: 1 in]
                                n1335 = Build Array(w1942, w1941, w1937, w1936, w1937) -> (w1944:dbl[])
                                }
                                }
                                }
                                }
                              }
                              frame True {
                                n1336 = flat-sequence {
                                tunnel: w1948 -> [w1949]
                                tunnel: [w1949] -> w1947
                                tunnel: w1947 -> [w1990]
                                tunnel: [w1990] -> w1946
                                tunnel: w1946 -> [w2017]
                                tunnel: [w2021] -> w1945
                                frame #0 {
                                w1958 = 0.0 ("element")
                                w1962 = 0.0 ("element")
                                w1964 = 0.0 ("element")
                                w1966 = 0.0 ("element")
                                w1968 = 0.0 ("element")
                                n1337 = Index Array(array=w1949, index #1=3 ("index"), index #2=2 ("index"), index #3=3 ("index"), index #4=2 ("index")) -> (element #1=w1978:dbl, element #2=w1980:dbl, element #3=w1983:dbl, element #4=w1972:dbl)
                                n1338 = Negate(x=w1980) -> (-x=w1979:dbl)
                                n1339 = Sine & Cosine(0:w1983) -> (1:w1975:dbl, 2:w1973:dbl)
                                n1340 = Multiply(x=w1979, y=w1975) -> (x*y=w1976:dbl)
                                n1341 = Multiply(x=w1973, y=w1972) -> (x*y=w1971:dbl)
                                n1342 = Cosine(x=w1978) -> (cos(x)=w1977:dbl)
                                n1343 = Build Array(w1968, w1968, w1977, w1976, 0.0 ("element")) -> (w1970:dbl[])
                                n1344 = Build Array(w1966, w1966, w1975, w1971, 0.0 ("element")) -> (w1969:dbl[])
                                n1345 = Build Array(w1964, w1964, w1964, w1964, w1964) -> (w1963:dbl[])
                                n1346 = Build Array(w1962, w1962, w1962, w1962, 1.0 ("element")) -> (w1960:dbl[])
                                n1347 = Build Array(w1958, w1958, w1958, w1958, w1958) -> (w1959:dbl[])
                                n1348 = Build Array(w1970, w1969, w1963, w1960, w1959) -> (w1956:dbl[][])
                                n1349 = call-poly <vilib>:"Array To Matrix.vi"("Real 2D Array"=w1956) -> ("Real Matrix"=w1954:T11)
                                n1350 = global read "G_rio.vi" "P"() -> (w1957:T11)
                                n1351 = Transpose Matrix(1:w1954) -> (0:w1953:T11)
                                n1352 = call-poly <vilib>:"Multiply.vi"("Real Matrix B"=w1957, "Real Matrix A"=w1954) -> ("A * B"=w1955:T11)
                                n1353 = call-poly <vilib>:"Multiply.vi"("Real Matrix B"=w1953, "Real Matrix A"=w1955) -> ("A * B"=w1952:T11)
                                n1354 = global read "G_rio.vi" "Q"() -> (w1951:T11)
                                n1355 = call-poly <vilib>:"Add.vi"("Real Matrix B"=w1951, "Real Matrix A"=w1952) -> ("A + B"=w1950:T11)
                                n1356 = global write "G_rio.vi" "Pp"(w1950) -> ()
                                }
                                frame #1 {
                                n1357 = global read "G_rio.vi" "Pp"() -> (w2015:T11)
                                n1358 = global read "G_rio.vi" "H"() -> (w2014:T11)
                                n1359 = Array Subset(array=w1990, index=0, length=2) -> (w1997:dbl[])
                                n1360 = local read "pos_gps"() -> (w1993:dbl[])
                                n1361 = call-poly <vilib>:"Multiply.vi"("Real Matrix B"=w2015, "Real Matrix A"=w2014) -> ("A * B"=w2013:T11)
                                n1362 = Transpose Matrix(1:w2014) -> (0:w2012:T11)
                                n1363 = call-poly <vilib>:"Multiply.vi"("Real Matrix B"=w2012, "Real Matrix A"=w2013) -> ("A * B"=w2011:T11)
                                n1364 = Array Subset(array=w1993, index=2, length=2) -> (w1996:dbl[])
                                n1365 = Subtract(x=w1996, y=w1997) -> (x-y=w1998:dbl[])
                                n1366 = global read "G_rio.vi" "H"() -> (w2009:T11)
                                n1367 = global read "G_rio.vi" "R"() -> (w2010:T11)
                                n1368 = global read "G_rio.vi" "Pp"() -> (w2008:T11)
                                n1369 = call-poly <vilib>:"Add.vi"("Real Matrix B"=w2010, "Real Matrix A"=w2011) -> ("A + B"=w2005:T11)
                                n1370 = Square(x=w1998) -> (x^2=w1999:dbl[])
                                n1371 = Transpose Matrix(1:w2009) -> (0:w2007:T11)
                                n1372 = local read "heading error"() -> (w2002:dbl)
                                n1373 = call-poly <vilib>:"Multiply.vi"("Real Matrix B"=w2007, "Real Matrix A"=w2008) -> ("A * B"=w2006:T11)
                                n1374 = Add Array Elements(numeric array=w1999) -> (sum=w2000:dbl)
                                n1375 = call-poly <vilib>:"Inverse Matrix.vi"("Input Matrix"=w2005) -> ("Inverse Matrix"=w2004:T11)  [unwired: 1 in, 1 out]
                                n1376 = call-poly <vilib>:"Multiply.vi"("Real Matrix B"=w2004, "Real Matrix A"=w2006) -> ("A * B"=w2003:T11)
                                n1377 = Square Root(x=w2000) -> (sqrt(x)=w1989:dbl)
                                n1378 = global write "G_rio.vi" "K"(w2003) -> ()
                                n1379 = Less?(x=w1989, y=2.5) -> (x < y?=w1986:bool)
                                n1380 = Less?(x=w2002, y=0.05) -> (x < y?=w1987:bool)
                                n1381 = And(x=w1987, y=w1986) -> (x .and. y?=w1985:bool)
                                n1382 = case shown="True" w1985 {
                                frame False {
                                }
                                frame True {
                                n1383 = local write "POS init"(FALSE ("Kalman init")) -> ()
                                }
                                }
                                }
                                frame #2 {
                                n1384 = disable-structure shown="Enabled" {
                                disable-tunnel: [w2039 w2041] -> w2019
                                disable-tunnel: w2017 -> [_ w2050]
                                frame Disabled {
                                n1385 = local read "get position"() -> (w2039:bool)
                                }
                                frame Enabled {
                                n1386 = Array Subset(array=w2050, index=0, length=2) -> (w2048:dbl[])
                                n1387 = local read "pos_gps"() -> (w2053:dbl[])
                                n1388 = Array Subset(array=w2053, index=2, length=2) -> (w2049:dbl[])
                                n1389 = disable-structure shown="Enabled" {
                                disable-tunnel: [w2056 TRUE ("Kalman init")] -> w2043
                                frame Disabled {
                                n1390 = local read "POS init"() -> (w2056:bool)
                                }
                                frame Enabled {
                                }
                                }
                                n1391 = Subtract(x=w2049, y=w2048) -> (x-y=w2047:dbl[])
                                n1392 = Square(x=w2047) -> (x^2=w2046:dbl[])
                                n1393 = Add Array Elements(numeric array=w2046) -> (sum=w2045:dbl)
                                n1394 = Square Root(x=w2045) -> (sqrt(x)=w2040:dbl)
                                n1395 = local write "pos error"(w2040) -> ()
                                n1396 = Less?(x=w2040, y=3.0) -> (x < y?=w2042:bool)
                                n1397 = Or(x=w2043, y=w2042) -> (x .or. y?=w2041:bool)
                                }
                                }
                                n1398 = disable-structure shown="Enabled" {
                                disable-tunnel: [w2033 w2034] -> w2020
                                frame Disabled {
                                n1399 = local read "get heading"() -> (w2033:bool)
                                }
                                frame Enabled {
                                n1400 = local read "heading error"() -> (w2037:dbl)
                                n1401 = local read "POS init"() -> (w2035:bool)
                                n1402 = Less?(x=w2037, y=0.1) -> (x < y?=w2036:bool)
                                n1403 = Or(x=w2036, y=w2035) -> (x .or. y?=w2034:bool)
                                }
                                }
                                n1404 = Index Array(array=w2017, index=3) -> (element=w2024:dbl)
                                n1405 = global read "G_rio.vi" "K"() -> (w2032:T11)
                                n1406 = global read "G_rio.vi" "H"() -> (w2031:T11)
                                n1407 = global read "G_rio.vi" "Pp"() -> (w2029:T11)
                                n1408 = call-poly <vilib>:"Multiply.vi"("Real Matrix B"=w2031, "Real Matrix A"=w2032) -> ("A * B"=w2030:T11)
                                n1409 = global read "G_rio.vi" "Pp"() -> (w2027:T11)
                                n1410 = call-poly <vilib>:"Multiply.vi"("Real Matrix B"=w2029, "Real Matrix A"=w2030) -> ("A * B"=w2028:T11)
                                n1411 = call-poly <vilib>:"Subtract.vi"("Real Matrix B"=w2028, "Real Matrix A"=w2027) -> ("A - B"=w2026:T11)
                                n1412 = global write "G_rio.vi" "P"(w2026) -> ()
                                n1413 = case shown="True" w2020 {
                                tunnel: w2024 -> [w2082 w2089]
                                tunnel: [w2082 w2084] -> w2018
                                frame False {
                                }
                                frame True {
                                n1414 = global read "G_rio.vi" "K"() -> (w2088:T11)
                                n1415 = Index Array(array=w2088, index (row)=3, index (col)=2 ("disabled index (col)")) -> (element=w2085:dbl)
                                n1416 = local read "h_gps"() -> (w2083:dbl)
                                n1417 = call "headingweightsum2.vi"("a"=w2085, "h2"=w2083, "h1"=w2089) -> ("a*h2+(1-a)*h1"=w2084:dbl)  [unwired: 8 in]
                                }
                                }
                                n1418 = case shown="True" w2019 {
                                tunnel: w2017 -> [w2058 w2070]
                                tunnel: [w2058 w2069] -> w2023
                                tunnel: w2018 -> [_ w2059]
                                frame False {
                                }
                                frame True {
                                n1419 = disable-structure shown="Enabled" {
                                disable-tunnel: [w2080 w2081] -> w2060
                                disable-tunnel: w2059 -> [_ w2081]
                                frame Disabled {
                                n1420 = local read "h_gps"() -> (w2080:dbl)
                                }
                                frame Enabled {
                                }
                                }
                                n1421 = local read "pos_gps"() -> (w2064:dbl[])
                                n1422 = call-poly <vilib>:"Array To Matrix.vi"("Real 1D Array"=w2070) -> ("Real Matrix (Column Vector)"=w2074:T11)
                                n1423 = Array Subset(array=w2064, index=2, length=2) -> (w2065:dbl[])
                                n1424 = Build Array (concatenate)(w2065, w2060) -> (w2061:dbl[])
                                n1425 = global read "G_rio.vi" "H"() -> (w2079:T11)
                                n1426 = call-poly <vilib>:"Multiply.vi"("Real Matrix B"=w2074, "Real Matrix A"=w2079) -> ("A * B"=w2078:T11)
                                n1427 = call-poly <vilib>:"Array To Matrix.vi"("Real 1D Array"=w2061) -> ("Real Matrix (Column Vector)"=w2077:T11)
                                n1428 = call-poly <vilib>:"Subtract.vi"("Real Matrix B"=w2078, "Real Matrix A"=w2077) -> ("A - B"=w2075:T11)
                                n1429 = global read "G_rio.vi" "K"() -> (w2076:T11)
                                n1430 = call-poly <vilib>:"Multiply.vi"("Real Matrix B"=w2075, "Real Matrix A"=w2076) -> ("A * B"=w2068:T11)
                                n1431 = call-poly <vilib>:"Multiply.vi"("Real Matrix A"=w2068, "Real Scalar c"=0.5) -> ("c * A"=w2066:T11)
                                n1432 = call-poly <vilib>:"Add.vi"("Real Matrix B"=w2074, "Real Matrix A"=w2066) -> ("A + B"=w2073:T11)
                                n1433 = call-poly <vilib>:"Matrix To Array.vi"("Real Matrix"=w2073) -> ("Real 2D Array"=w2072:dbl[][])
                                n1434 = Index Array(array=w2072, index (col)=0 ("disabled index (col)")) -> (element=w2069:dbl[])  [unwired: 1 in]
                                }
                                }
                                n1435 = Replace Array Subset(array=w2023, new element=w2018, index=3) -> (w2021:dbl[])
                                }
                                }
                              }
                            }
                          }
                        }
                      }
                    }
                  }
                }
              }
              frame Disabled {
                n1436 = flat-sequence {
                  tunnel: [w2119] -> w2111
                  tunnel: w2112 -> [w2120]
                  tunnel: w2111 -> [w2146]
                  tunnel: [w2145] -> w2110
                  tunnel: [w2144] -> w2108
                  tunnel: [w2143] -> w2107
                  tunnel: w2110 -> [w2241]
                  tunnel: [w2241] -> w2109
                  tunnel: w2108 -> [w2233]
                  tunnel: w2107 -> [w2232]
                  tunnel: w2109 -> [w2254]
                  tunnel: [w2253] -> w2106
                  tunnel: w2106 -> [w2279]
                  tunnel: [w2279] -> w2105
                  tunnel: [w2278] -> w2104
                  tunnel: [w2277] -> w2103
                  tunnel: [w2276] -> w2102
                  tunnel: [w2275] -> w2101
                  tunnel: [w2274] -> w2100
                  tunnel: [w2382] -> w2099
                  tunnel: w2105 -> [w2382]
                  tunnel: w2104 -> [w2375]
                  tunnel: w2103 -> [w2376]
                  tunnel: w2102 -> [w2369]
                  tunnel: w2101 -> [w2368]
                  tunnel: w2100 -> [w2365]
                  frame #0 {
                    n1437 = Index Array(array=w2120, index=3) -> (element=w2125:dbl)
                    n1438 = global read "G_rio.vi" "VS_CAN"() -> (w2116:dbl)
                    n1439 = Equal To 0?(x=w2116) -> (x = 0?=w2115:bool)
                    n1440 = case shown="False" w2115 {
                      tunnel: [w2127 _] -> w2114
                      frame False {
                        n1441 = global read "G_rio.vi" "yaw_rate"() -> (w2130:dbl)
                        n1442 = local read "hbias"() -> (w2131:dbl)
                        n1443 = Subtract(x=w2130, y=w2131) -> (x-y=w2128:dbl)
                        n1444 = Negate(x=w2128) -> (-x=w2129:dbl)
                        n1445 = call "angleconv.vi"("deg"=w2129) -> ("rad"=w2127:dbl)  [unwired: 9 in, 1 out]
                      }
                      frame True {
                        w2135 = u64 18446744073709551615
                        n1446 = local read "hcount"() -> (w2138:u64)
                        n1447 = local read "hbias"() -> (w2141:dbl)
                        n1448 = Increment(x=w2138) -> (x+1=w2137:u64)
                        n1449 = global read "G_rio.vi" "yaw_rate"() -> (w2132:dbl)
                        n1450 = Not Equal?(x=w2138, y=w2135) -> (x != y?=w2136:bool)
                        n1451 = Multiply(x=w2141, y=w2138) -> (x*y=w2140:dbl)
                        n1452 = Add(x=w2132, y=w2140) -> (x+y=w2139:dbl)
                        n1453 = Select(t=w2137, s=w2136, f=w2135) -> (s? t:f=w2134:u64)
                        n1454 = local write "hcount"(w2134) -> ()
                        n1455 = Divide(x=w2139, y=w2134) -> (x/y=w2133:dbl)
                        n1456 = local write "hbias"(w2133) -> ()
                      }
                    }
                    n1457 = local read item#-1() -> (w2118)
                    n1458 = Subtract(x=w2114, y=w2118) -> (x-y=w2124:dbl)
                    n1459 = local read "dt"() -> (w2123:dbl)
                    n1460 = Multiply(x=w2124, y=w2123) -> (x*y=w2113:dbl)
                    n1461 = local write "rt"(w2113) -> ()
                    n1462 = call "headingoperater.vi"("h1"=w2113, "h2"=w2125) -> ("h2+h1"=w2122:dbl)  [unwired: 8 in, 1 out]
                    n1463 = Replace Array Subset(array=w2120, new element #1=w2122, index #1=3 ("index"), new element #2=w2114, index #2=4 ("index")) -> (w2119:dbl[])
                  }
                  frame #1 {
                    n1464 = global read "G_rio.vi" "gps_vel 1"() -> (w2173:dbl[])
                    n1465 = global read "G_rio.vi" "gps_vel 2"() -> (w2162:dbl[])
                    n1466 = global read "G_rio.vi" "VS_CAN"() -> (w2150:dbl)
                    n1467 = Index Array(array=w2173, index #1=1 ("index"), index #2=0 ("index"), index #3=0 ("index")) -> (element #1=w2168:dbl, element #2=w2157:dbl, element #3=w2151:dbl)
                    n1468 = Index Array(array=w2162, index #1=0 ("index"), index #2=1 ("index"), index #3=0 ("index")) -> (element #1=w2153:dbl, element #2=w2167:dbl, element #3=w2156:dbl)
                    n1469 = Equal?(x=w2151, y=w2153) -> (x = y?=w2155:bool)
                    n1470 = Absolute Value(x=w2150) -> (abs(x)=w2149:dbl)
                    n1471 = feedback-in #30(w2157) -> ()
                    n1472 = feedback #30(0.0 ("Real Matrix Element")) -> (w2170:dbl)
                    n1473 = feedback #31(0.0 ("Real Matrix Element")) -> (w2165:dbl)
                    n1474 = feedback-in #31(w2156) -> ()
                    n1475 = Greater?(x=w2157, y=w2170) -> (0:w2160:bool)
                    n1476 = Greater?(x=w2156, y=w2165) -> (0:w2158:bool)
                    n1477 = Not Equal To 0?(x=w2168) -> (x != 0?=w2161:bool)
                    n1478 = Not Equal To 0?(x=w2167) -> (x != 0?=w2159:bool)
                    n1479 = Greater?(x=w2149, y=5.0) -> (0:w2147:bool)
                    n1480 = Compound Arithmetic op=AND(w2147, w2161, w2160, w2155, w2159, w2158) -> (w2142:bool)
                    n1481 = case shown="True" w2142 {
                      tunnel: w2146 -> [w2180 w2206]
                      tunnel: [w2181 w2198] -> w2144
                      tunnel: [w2180 w2206] -> w2145
                      tunnel: [w2179 w2203] -> w2143
                      frame False {
                        n1482 = local read item#-1() -> (w2177)
                        n1483 = Multiply(x=0.9875 ("value"), y=w2177) -> (x*y=w2176:dbl)
                        n1484 = Add(x=0.011 ("value"), y=w2176) -> (x+y=w2174:dbl)
                        n1485 = local read item#-1() -> (w2179)
                        n1486 = Compound Arithmetic op=MULTIPLY(w2174, w2179) -> (w2181:dbl)
                      }
                      frame True {
                        w2205 = 0.001745329251994  # 0.1deg
                        n1487 = Index Array(array=w2206, index=3) -> (element=w2208:dbl)
                        n1488 = global read "G_rio.vi" "gps_vel 1"() -> (w2220:dbl[])
                        n1489 = global read "G_rio.vi" "gps_vel 2"() -> (w2218:dbl[])
                        n1490 = Index Array(array=w2220, index #1=4 ("index"), index #2=2 ("index")) -> (element #1=w2202:dbl, element #2=w2195:dbl)
                        n1491 = Index Array(array=w2218, index #1=4 ("index"), index #2=2 ("index")) -> (element #1=w2200:dbl, element #2=w2194:dbl)
                        n1492 = global read "G_rio.vi" "VS_CAN"() -> (w2187:dbl)
                        n1493 = global read "G_rio.vi" "VS_CAN"() -> (w2212:dbl)
                        n1494 = Add(x=w2195, y=w2194) -> (x+y=w2193:dbl)
                        n1495 = call "angleconv.vi"("deg"=w2202) -> ("rad"=w2201:dbl)  [unwired: 9 in, 1 out]
                        n1496 = call "angleconv.vi"("deg"=w2200) -> ("rad"=w2199:dbl)  [unwired: 9 in, 1 out]
                        n1497 = Absolute Value(x=w2187) -> (abs(x)=w2186:dbl)
                        n1498 = Greater Or Equal To 0?(x=w2212) -> (x >= 0?=w2213:bool)
                        n1499 = Multiply(x=w2193, y=0.5) -> (x*y=w2185:dbl)
                        n1500 = call "headingweightsum.vi"("a"=0.5, "h1"=w2199, "h2"=w2201) -> ("a*h2+(1-a)*h1"=w2211:dbl)  [unwired: 8 in]
                        n1501 = Divide(x=w2185, y=w2186) -> (x/y=w2184:dbl)
                        n1502 = Select(t=0.0, s=w2213, f=3.141592653589793) -> (s? t:f=w2210:dbl)
                        n1503 = Decrement(x=w2184) -> (x-1=w2191:dbl)
                        n1504 = call "headingoperater.vi"("h1"=w2210, "h2"=w2211) -> ("h2-h1"=w2183:dbl)  [unwired: 8 in, 1 out]
                        n1505 = local write "h_gps"(w2183) -> ()
                        n1506 = Absolute Value(x=w2191) -> (abs(x)=w2190:dbl)
                        n1507 = call "headingoperater.vi"("h1"=w2183, "h2"=w2208) -> ("h2-h1"=w2198:dbl)  [unwired: 8 in, 1 out]
                        n1508 = Less?(x=w2190, y=0.05) -> (x < y?=w2188:bool)
                        n1509 = case shown="True" w2188 {
                          tunnel: w2184 -> [_ w2228]
                          frame False {
                          }
                          frame True {
                            w2222 = u64 18446744073709551615
                            n1510 = local read "vcount"() -> (w2225:u64)
                            n1511 = local read "vgain"() -> (w2230:dbl)
                            n1512 = Increment(x=w2225) -> (x+1=w2224:u64)
                            n1513 = Not Equal?(x=w2225, y=w2222) -> (x != y?=w2223:bool)
                            n1514 = Multiply(x=w2230, y=w2225) -> (x*y=w2229:dbl)
                            n1515 = Add(x=w2228, y=w2229) -> (x+y=w2227:dbl)
                            n1516 = Select(t=w2224, s=w2223, f=w2222) -> (s? t:f=w2221:u64)
                            n1517 = Divide(x=w2227, y=w2221) -> (x/y=w2226:dbl)
                            n1518 = local write "vcount"(w2221) -> ()
                            n1519 = local write "vgain"(w2226) -> ()
                          }
                        }
                        n1520 = Absolute Value(x=w2198) -> (abs(x)=w2204:dbl)
                        n1521 = call "angleconv.vi"("rad"=w2198) -> ("deg"=w2182:dbl)  [unwired: 9 in, 1 out]
                        n1522 = Greater?(x=w2205, y=w2204) -> (0:w2207:bool)
                        n1523 = local write "heading error"(w2182) -> ()
                        n1524 = case shown="True" w2207 {
                          frame False {
                          }
                          frame True {
                            n1525 = local write item#-1(0.0 ("initH")) -> ()
                          }
                        }
                        n1526 = local read item#-1() -> (w2203)
                      }
                    }
                    n1527 = local write "get heading"(w2142) -> ()
                  }
                  frame #2 {
                    n1528 = local write item#-1(w2233) -> ()
                    n1529 = Multiply(x=w2233, y="heading gain") -> (x*y=w2240:dbl)
                    n1530 = Negate(x="heading gain") -> (-x=w2237:dbl)
                    n1531 = Multiply(x=w2237, y=w2232) -> (x*y=w2239:dbl)
                    n1532 = feedback #32(0.0) -> (w2234:dbl)
                    n1533 = Compound Arithmetic op=ADD(w2240, w2239, w2234) -> (w2236:dbl)
                    n1534 = local write item#-1(w2236) -> ()
                    n1535 = feedback-in #32(w2236) -> ()
                  }
                  frame #3 {
                    n1536 = global read "G_rio.vi" "VS_CAN"() -> (w2243:dbl)
                    n1537 = Index Array(array=w2254, index #1=1 ("index"), index #2=3 ("index"), index #3=0 ("index")) -> (element #1=w2258:dbl, element #2=w2270:dbl, element #3=w2256:dbl)
                    n1538 = local read "vgain"() -> (w2244:dbl)
                    n1539 = call "headingoperater.vi"("h1"=w2270, "h2"=1.5707963267948966) -> ("h2-h1"=w2269:dbl)  [unwired: 8 in, 1 out]
                    n1540 = Multiply(x=w2243, y=w2244) -> (x*y=w2242:dbl)
                    n1541 = Sine & Cosine(0:w2269) -> (1:w2266:dbl, 2:w2267:dbl)
                    n1542 = Divide(x=w2242, y=3.6) -> (x/y=w2247:dbl)
                    n1543 = Multiply(x=w2266, y=w2247) -> (x*y=w2264:dbl)
                    n1544 = Multiply(x=w2247, y=w2267) -> (x*y=w2265:dbl)
                    n1545 = local read item#-1() -> (w2246)
                    n1546 = local read item#-1() -> (w2245)
                    n1547 = Subtract(x=w2264, y=w2246) -> (x-y=w2263:dbl)
                    n1548 = Subtract(x=w2265, y=w2245) -> (x-y=w2261:dbl)
                    n1549 = local read "dt"() -> (w2262:dbl)
                    n1550 = Multiply(x=w2263, y=w2262) -> (x*y=w2259:dbl)
                    n1551 = Multiply(x=w2262, y=w2261) -> (x*y=w2257:dbl)
                    n1552 = Add(x=w2258, y=w2259) -> (x+y=w2251:dbl)
                    n1553 = Add(x=w2257, y=w2256) -> (x+y=w2249:dbl)
                    n1554 = Replace Array Subset(array=w2254, new element #1=w2251, index #1=1 ("index"), new element #2=w2249, index #2=0 ("index"), new element #3=w2247, index #3=2 ("index")) -> (w2253:dbl[])
                  }
                  frame #4 {
                    n1555 = global read "G_rio.vi" "gps_pos 1"() -> (w2306:dbl[])
                    n1556 = global read "G_rio.vi" "gps_pos 2"() -> (w2295:dbl[])
                    n1557 = global read "G_rio.vi" "VS_CAN"() -> (w2283:dbl)
                    n1558 = Index Array(array=w2306, index #1=1 ("index"), index #2=0 ("index"), index #3=0 ("index")) -> (element #1=w2301:dbl, element #2=w2290:dbl, element #3=w2284:dbl)
                    n1559 = Index Array(array=w2295, index #1=0 ("index"), index #2=1 ("index"), index #3=0 ("index")) -> (element #1=w2286:dbl, element #2=w2300:dbl, element #3=w2289:dbl)
                    n1560 = Equal?(x=w2284, y=w2286) -> (x = y?=w2288:bool)
                    n1561 = Absolute Value(x=w2283) -> (abs(x)=w2282:dbl)
                    n1562 = feedback #33(0.0 ("Real Matrix Element")) -> (w2303:dbl)
                    n1563 = feedback-in #33(w2290) -> ()
                    n1564 = feedback #34(0.0 ("Real Matrix Element")) -> (w2298:dbl)
                    n1565 = feedback-in #34(w2289) -> ()
                    n1566 = Greater?(x=w2290, y=w2303) -> (0:w2293:bool)
                    n1567 = Greater?(x=w2289, y=w2298) -> (0:w2291:bool)
                    n1568 = Not Equal To 0?(x=w2301) -> (x != 0?=w2294:bool)
                    n1569 = Not Equal To 0?(x=w2300) -> (x != 0?=w2292:bool)
                    n1570 = Greater?(x=w2282, y=5.0) -> (0:w2280:bool)
                    n1571 = Compound Arithmetic op=AND(w2280, w2294, w2293, w2288, w2292, w2291) -> (w2273:bool)
                    n1572 = case shown="True" w2273 {
                      tunnel: w2279 -> [_ w2359]
                      tunnel: [w2322 w2340] -> w2278
                      tunnel: [w2323 w2341] -> w2276
                      tunnel: [1.0 w2331] -> w2274
                      tunnel: [w2318 w2343] -> w2277
                      tunnel: [w2317 w2342] -> w2275
                      frame False {
                        n1573 = local read item#-1() -> (w2313)
                        n1574 = local read item#-1() -> (w2316)
                        n1575 = Multiply(x=0.9 ("value"), y=w2313) -> (x*y=w2312:dbl)
                        n1576 = Multiply(x=w2316, y=0.9) -> (x*y=w2309:dbl)
                        n1577 = Add(x=w2312, y=0.01 ("value")) -> (x+y=w2310:dbl)
                        n1578 = Add(x=w2309, y=0.01 ("value")) -> (x+y=w2307:dbl)
                        n1579 = local read item#-1() -> (w2321)
                        n1580 = local read item#-1() -> (w2319)
                        n1581 = Compound Arithmetic op=MULTIPLY(w2310, w2321) -> (w2323:dbl)
                        n1582 = Compound Arithmetic op=MULTIPLY(w2319, w2307) -> (w2322:dbl)
                        n1583 = local read item#-1() -> (w2317)
                        n1584 = local read item#-1() -> (w2318)
                      }
                      frame True {
                        n1585 = global read "G_rio.vi" "gps_pos 1"() -> (w2348:dbl[])
                        n1586 = global read "G_rio.vi" "gps_pos 2"() -> (w2347:dbl[])
                        n1587 = Add(x=w2348, y=w2347) -> (x+y=w2358:dbl[])
                        n1588 = Index Array(array=w2359, index #1=0 ("index"), index #2=1 ("index")) -> (element #1=w2349:dbl, element #2=w2351:dbl)
                        n1589 = Multiply(x=w2358, y=0.5) -> (x*y=w2325:dbl[])
                        "pos_gps" <- w2325
                        n1590 = Index Array(array=w2325, index #1=3 ("index"), index #2=2 ("index"), index #3=9 ("index")) -> (element #1=w2354:dbl, element #2=w2353:dbl, element #3=w2327:dbl)
                        n1591 = Subtract(x=w2351, y=w2353) -> (x-y=w2341:dbl)
                        n1592 = Subtract(x=w2349, y=w2354) -> (x-y=w2340:dbl)
                        n1593 = local read item#-1() -> (w2333)
                        n1594 = Divide(x=0.9, y=w2327) -> (x/y=w2345:dbl)
                        n1595 = Square(x=w2340) -> (x^2=w2336:dbl)
                        n1596 = Square(x=w2341) -> (x^2=w2335:dbl)
                        n1597 = Not Equal To 0?(x=w2333) -> (x != 0?=w2334:bool)
                        n1598 = Max & Min(x=w2345, y=1.0) -> (min(x,y)=w2332:dbl)  [unwired: 1 out]
                        n1599 = Add(x=w2336, y=w2335) -> (x+y=w2326:dbl)
                        n1600 = Select(t=w2333, s=w2334, f=w2332) -> (s? t:f=w2331:dbl)
                        n1601 = local read item#-1() -> (w2338)
                        n1602 = Square Root(x=w2326) -> (sqrt(x)=w2324:dbl)
                        n1603 = Equal To 0?(x=w2338) -> (x = 0?=w2330:bool)
                        n1604 = Less?(x=w2326, y=1.0) -> (x < y?=w2329:bool)
                        n1605 = local write "pos error"(w2324) -> ()
                        n1606 = And(x=w2330, y=w2329) -> (x .and. y?=w2337:bool)
                        n1607 = case shown="True" w2337 {
                          frame False {
                          }
                          frame True {
                            n1608 = local write "POS init"(FALSE ("Kalman init")) -> ()
                            n1609 = local write item#-1(0.0 ("initP")) -> ()
                          }
                        }
                        n1610 = local read item#-1() -> (w2342)
                        n1611 = local read item#-1() -> (w2343)
                      }
                    }
                    n1612 = local write "get position"(w2273) -> ()
                  }
                  frame #5 {
                    n1613 = local write item#-1(w2369) -> ()
                    n1614 = local write item#-1(w2375) -> ()
                    n1615 = Multiply(x=w2369, y="pos gain") -> (x*y=w2372:dbl)
                    n1616 = Multiply(x=w2375, y="pos gain") -> (x*y=w2379:dbl)
                    n1617 = Negate(x="pos gain") -> (-x=w2373:dbl)
                    n1618 = Negate(x="pos gain") -> (-x=w2378:dbl)
                    n1619 = Multiply(x=w2373, y=w2368) -> (x*y=w2374:dbl)
                    n1620 = Multiply(x=w2378, y=w2376) -> (x*y=w2377:dbl)
                    n1621 = feedback #35(0.0) -> (w2370:dbl)
                    n1622 = Compound Arithmetic op=ADD(w2372, w2374, w2370) -> (w2367:dbl)
                    n1623 = feedback-in #35(w2367) -> ()
                    n1624 = feedback #36(0.0) -> (w2381:dbl)
                    n1625 = Compound Arithmetic op=ADD(w2379, w2377, w2381) -> (w2364:dbl)
                    n1626 = feedback-in #36(w2364) -> ()
                    n1627 = Multiply(x=w2367, y=w2365) -> (x*y=w2366:dbl)
                    n1628 = Multiply(x=w2365, y=w2364) -> (x*y=w2363:dbl)
                    n1629 = local write item#-1(w2366) -> ()
                    n1630 = local write item#-1(w2363) -> ()
                  }
                }
                n1631 = Index Array(array=w2099, index #1=1 ("index"), index #2=0 ("index"), index #3=2 ("index")) -> (element #1=w2095:dbl, element #2=w2094:dbl, element #3=w2093:dbl, element #4=w2092:dbl, element #5=w2091:dbl)  [unwired: 2 in]
                n1632 = Build Array(w2095, w2094, w2093, w2092, w2091) -> (w2090:dbl[])
              }
            }
          }
          frame #2 {
            n1633 = flat-sequence {
              tunnel: w2384 -> [w2391]
              frame #0 {
                n1634 = local read "dt"() -> (w2388:dbl)
                n1635 = Array Subset(array=w2391, index=0, length=2) -> (w2399:dbl[])
                "pos" <- w2399
                n1636 = Index Array(array=w2391, index=3) -> (element=w2396:dbl)
                n1637 = Greater Than 0?(x=w2388) -> (x > 0?=w2386:bool)
                n1638 = call "angleconv.vi"("rad"=w2396) -> ("deg"=→"Heading":dbl)  [unwired: 9 in, 1 out]
                n1639 = Greater?(x=1.0, y=w2388) -> (0:w2390:bool)
                n1640 = local read "LCM"() -> (w2387:bool)
                n1641 = local read "h_gps"() -> (w2392:dbl)
                n1642 = Compound Arithmetic op=AND(w2390, w2386, w2387) -> (w2385:bool)
                n1643 = case shown="True" w2385 {
                  tunnel: w2399 -> [w2409 _]
                  tunnel: w2396 -> [w2405 _]
                  tunnel: w2392 -> [w2404 _]
                  tunnel: w2391 -> [_ w2416]
                  frame False {
                    n1644 = local read "pos_gps"() -> (w2408:dbl[])
                    n1645 = global read "G_rio.vi" "VS_CAN"() -> (w2402:dbl)
                    n1646 = Array Subset(array=w2408, index=5, length=10) -> (w2413:dbl[])
                    n1647 = Array Subset(array=w2408, index=12, length=3) -> (w2410:dbl[])
                    n1648 = local read "map"() -> (w2403:i32)
                    n1649 = local read "dt"() -> (w2407:dbl)
                    n1650 = Build Array (concatenate)(w2413, w2410, w2409, w2407, w2403, w2402, w2405, w2404) -> (w2406:dbl[])
                    n1651 = shared-variable "veloster\\sharedvari.lvlib\\RIONAV"(w2406) -> ()  [unwired: 1 in, 1 out]
                  }
                  frame True {
                    n1652 = flat-sequence {
                      tunnel: w2416 -> [w2441]
                      frame #0 {
                        n1653 = Get Date/Time In Seconds() -> (seconds since 1Jan1904=w2432:timestamp)
                        n1654 = To Double Precision Float(number=w2432) -> (double precision float=w2426:dbl)
                        n1655 = global read "G_rio.vi" "LCM_POS_T"() -> (w2440:T18)
                        n1656 = local read "POS init"() -> (w2421:bool)
                        n1657 = Unbundle By Name(w2440) -> ("hash"=w2437:i64)
                        n1658 = local read "dt"() -> (w2420:dbl)
                        n1659 = Multiply(x=w2426, y=1000000.0) -> (x*y=w2424:dbl)
                        n1660 = Array To Cluster(array=w2441) -> (cluster=w2439:T19)
                        n1661 = Select(t=0.0, s=w2421, f=w2420) -> (s? t:f=w2418:dbl)
                        n1662 = call "hash.vi"("input"=w2437) -> ("output"=w2436:i64)  [unwired: 10 in]
                        n1663 = To Quad Integer(1:w2424) -> (0:w2423:i64)
                        n1664 = Unbundle(w2439) -> ("Real 2D Array[0]"=w2431:dbl, "Real 2D Array[1]"=w2430:dbl, "Real 2D Array[2]"=w2429:dbl, "Real 2D Array[3]"=w2428:dbl, "Real 2D Array[4]"=w2427:dbl)
                        n1665 = local read "file write"() -> (w2422:bool)
                        n1666 = Bundle(cluster=w2440, "hash"=w2436, "sys time"=w2423, "dt"=w2418, "x"=w2431, "y"=w2430, "speed"=w2429, "heading"=w2428, "yaw_rate"=w2427) -> (w2417:T18)
                        n1667 = case shown="True" w2422 {
                          tunnel: w2417 -> [_ w2442]
                          frame False {
                          }
                          frame True {
                            n1668 = local read "data write"() -> (w2443:refnum<file>)
                            n1669 = Write to Binary File(file (use dialog)=w2443, data=w2442) -> ()  [unwired: 4 in, 3 out]
                          }
                        }
                        n1670 = Flatten To String(anything=w2417, prepend array or string size? (T)=FALSE) -> (data string=w2434:string)  [unwired: 2 in, 2 out]
                        n1671 = global read "G_rio.vi" "LCM"() -> (w2433:T4)
                        n1672 = call "LCM_send.vi"("DATA"=w2434, "ID"="POS_T", "LCM"=w2433) -> ()  [unwired: 7 in, 2 out]
                      }
                    }
                  }
                }
                n1673 = call "headingoperater.vi"("h1"=0.0, "h2"=w2392) -> ("h2+h1"=w2393:dbl)  [unwired: 8 in, 1 out]
                n1674 = call "angleconv.vi"("rad"=w2393) -> ("deg"=→"H_GPS":dbl)  [unwired: 9 in, 1 out]
              }
            }
          }
        }
      }
    }
  }
